vi "TLB Native Dynamic Events ver 0.18c.vi"() -> ()   [LabVIEW 2018]
uses:
  Labview Training Phase 2/Enum Controls/States for Action Engine.ctl
  TLB Type Definitions/State Type Definitions, for 0.26d versions and later.ctl
  TLB Type Definitions/Intruction Type Definitions.ctl
  TLB Type Definitions/Encoder cluster.ctl
  TLB Type Definitions/PING CLUSTER.ctl
  <vilib>/Studica/Studica Toolkit/NavX/NavX.lvlib
  <vilib>/Studica/Studica Toolkit/Background/DIO Channel.ctl
  Underlying VI's/NavX VI/navX type def.ctl
  <vilib>/Studica/Studica Toolkit/Background/I2C Channel.ctl
  TLB Type Definitions/Vision cluster.ctl
  <vilib>/NI_Real-Time Target Support.lvlib
  TLB Type Definitions/Stepper cluster.ctl
  Experimental VI's/Archived VI's/MOTOR CONTROL NO PID Type Def.ctl
  Underlying VI's/I2C Master VI/I2C MASTER Type Def.ctl
  Underlying VI's/I2C Master VI/I2C_MASTER_WRITE_NEW Type Def.ctl
  <vilib>/userdefined/High Color/IMAQdx.ctl
  Underlying VI's/I2C Master VI/Arduino_Interfacing.ctl
  TLB Type Definitions/Yaw Cluster.ctl
  TLB Type Definitions/Time cluster.ctl
  TLB Type Definitions/Y Stepper cluster.ctl
  Underlying VI's/Modified webcam FGV/Webcam AE.ctl
  Underlying VI's/Elasped Timer/Elapsed timer control.ctl
  Underlying VI's/Motor Control VI with PID/MOTOR CONTROL WITH PID AE DATA MODE TYPE DEF.ctl
  Underlying VI's/Motor Control VI with PID/MOTOR CONTROL WITH PID AE DIRECTION TYPE DEF.ctl
  TLB Type Definitions/IR Sensor Type Def.ctl
  <vilib>/myRIO/Common/Instrument Driver Framework/myRIO v1.0/AI/typedefs/AI Channels Enum.ctl
  <vilib>/myRIO/Common/Instrument Driver Framework/myRIO v1.0/AI/typedefs/AI Channels List.ctl
  TLB Type Definitions/Motor Speed Cluster.ctl
  Underlying VI's/IMAQ Create Reference AE/IMAQ Reference AE.ctl
  TLB Type Definitions/Line Sensor Cluster.ctl
  Underlying VI's/Line Sensor AE/Line Sensor AE Type Def.ctl
  <vilib>/Utility/RT CPU Load.ctl
  <vilib>/Studica/Studica Toolkit/NavX/TypeDefs/Flags/Z900_navX_Flags_CalibrationStatusTypeDef.ctl
  <vilib>/Studica/Studica Toolkit/NavX/TypeDefs/Flags/Z900_navX_Flags_OpStatusTypeDef.ctl
panel:
  out "Status":T3 {"OP Status" items=["INITIALIZING", "SELFTEST_IN_PROGRESS", "ERROR", "IMU_AUTOCAL_IN_PROGRESS", "NORMAL"]; "Calibration Status" items=["IMU_CAL_STATE_MASK"=3, "IMU_CAL_STATE_INPROGRESS"=0, "IMU_CAL_STATE_ACCUMULATE"=1, "IMU_CAL_STATE_COMPLETE"=2]}
  out "General Errors":errorcluster
  in  "Red LED":bool
  out "Arm IR Sensor":dbl
  out "Table obstruct":bool
  out "x-y":dbl
  out "Left IR Sensor":dbl
  out "Obstacle detected":bool
  out "Speed & distance":T4
  out "Object Center Coordinates":cluster{"x":sgl, "y":sgl}
  out "Object detection cluster":T5
  out "Time up flag":bool
  out "Task selection":u8
  in  "Object recognition mode":enum16{"Ball", "Soap", "Gel", "Pipe", "None"}(ring)
  out "NavX Readings":T6
  out "Arduino Data":T7
  out "CPU loads":T8[](array[typedef]) {"ISR (%)" format="%#.2f"; "Idle (%)" format="%#.2f"; "Background (%)" format="%#.2f"; "Normal (%)" format="%#.2f"; "Above Normal (%)" format="%#.2f"; "High (%)" format="%#.2g"; "Timed Structures (%)" format="%#.2g"; "Time Critical (%)" format="%#.2g"; "Total (%)" format="%#.2g"}
  out "TASK ENABLE":bool
  out "Rising Edge":bool
  in  "Green LED":bool
  out "State Logic":T9=enum."Startup"
  out "elements":T10[](array[typedef])
  in  "STOP TASK":bool
  in  "OK Button":bool
  in  "STOP":bool
  out "Queue Errors":errorcluster
  out "Action Queue Items":i32
  out "State Logic Queue Items":i32
  out "Action Queues items":string[](array[string])=["Hardware reset", "Software reset", ""]
  out "Action State":string
  # "System Health Status Update"
  # "VISION"
  # "TLB FRAMEWORK STATUS"
  # "Test Programme written by Calvin Loke    Dated: 28 Aug 2019\nTest Programme revised by Dr Alex See   Dated 30 Aug 2019\n\nRevision date: 20/03/2020\nProgramme version:   TLB Native Dynamic Events ver 0.14a"
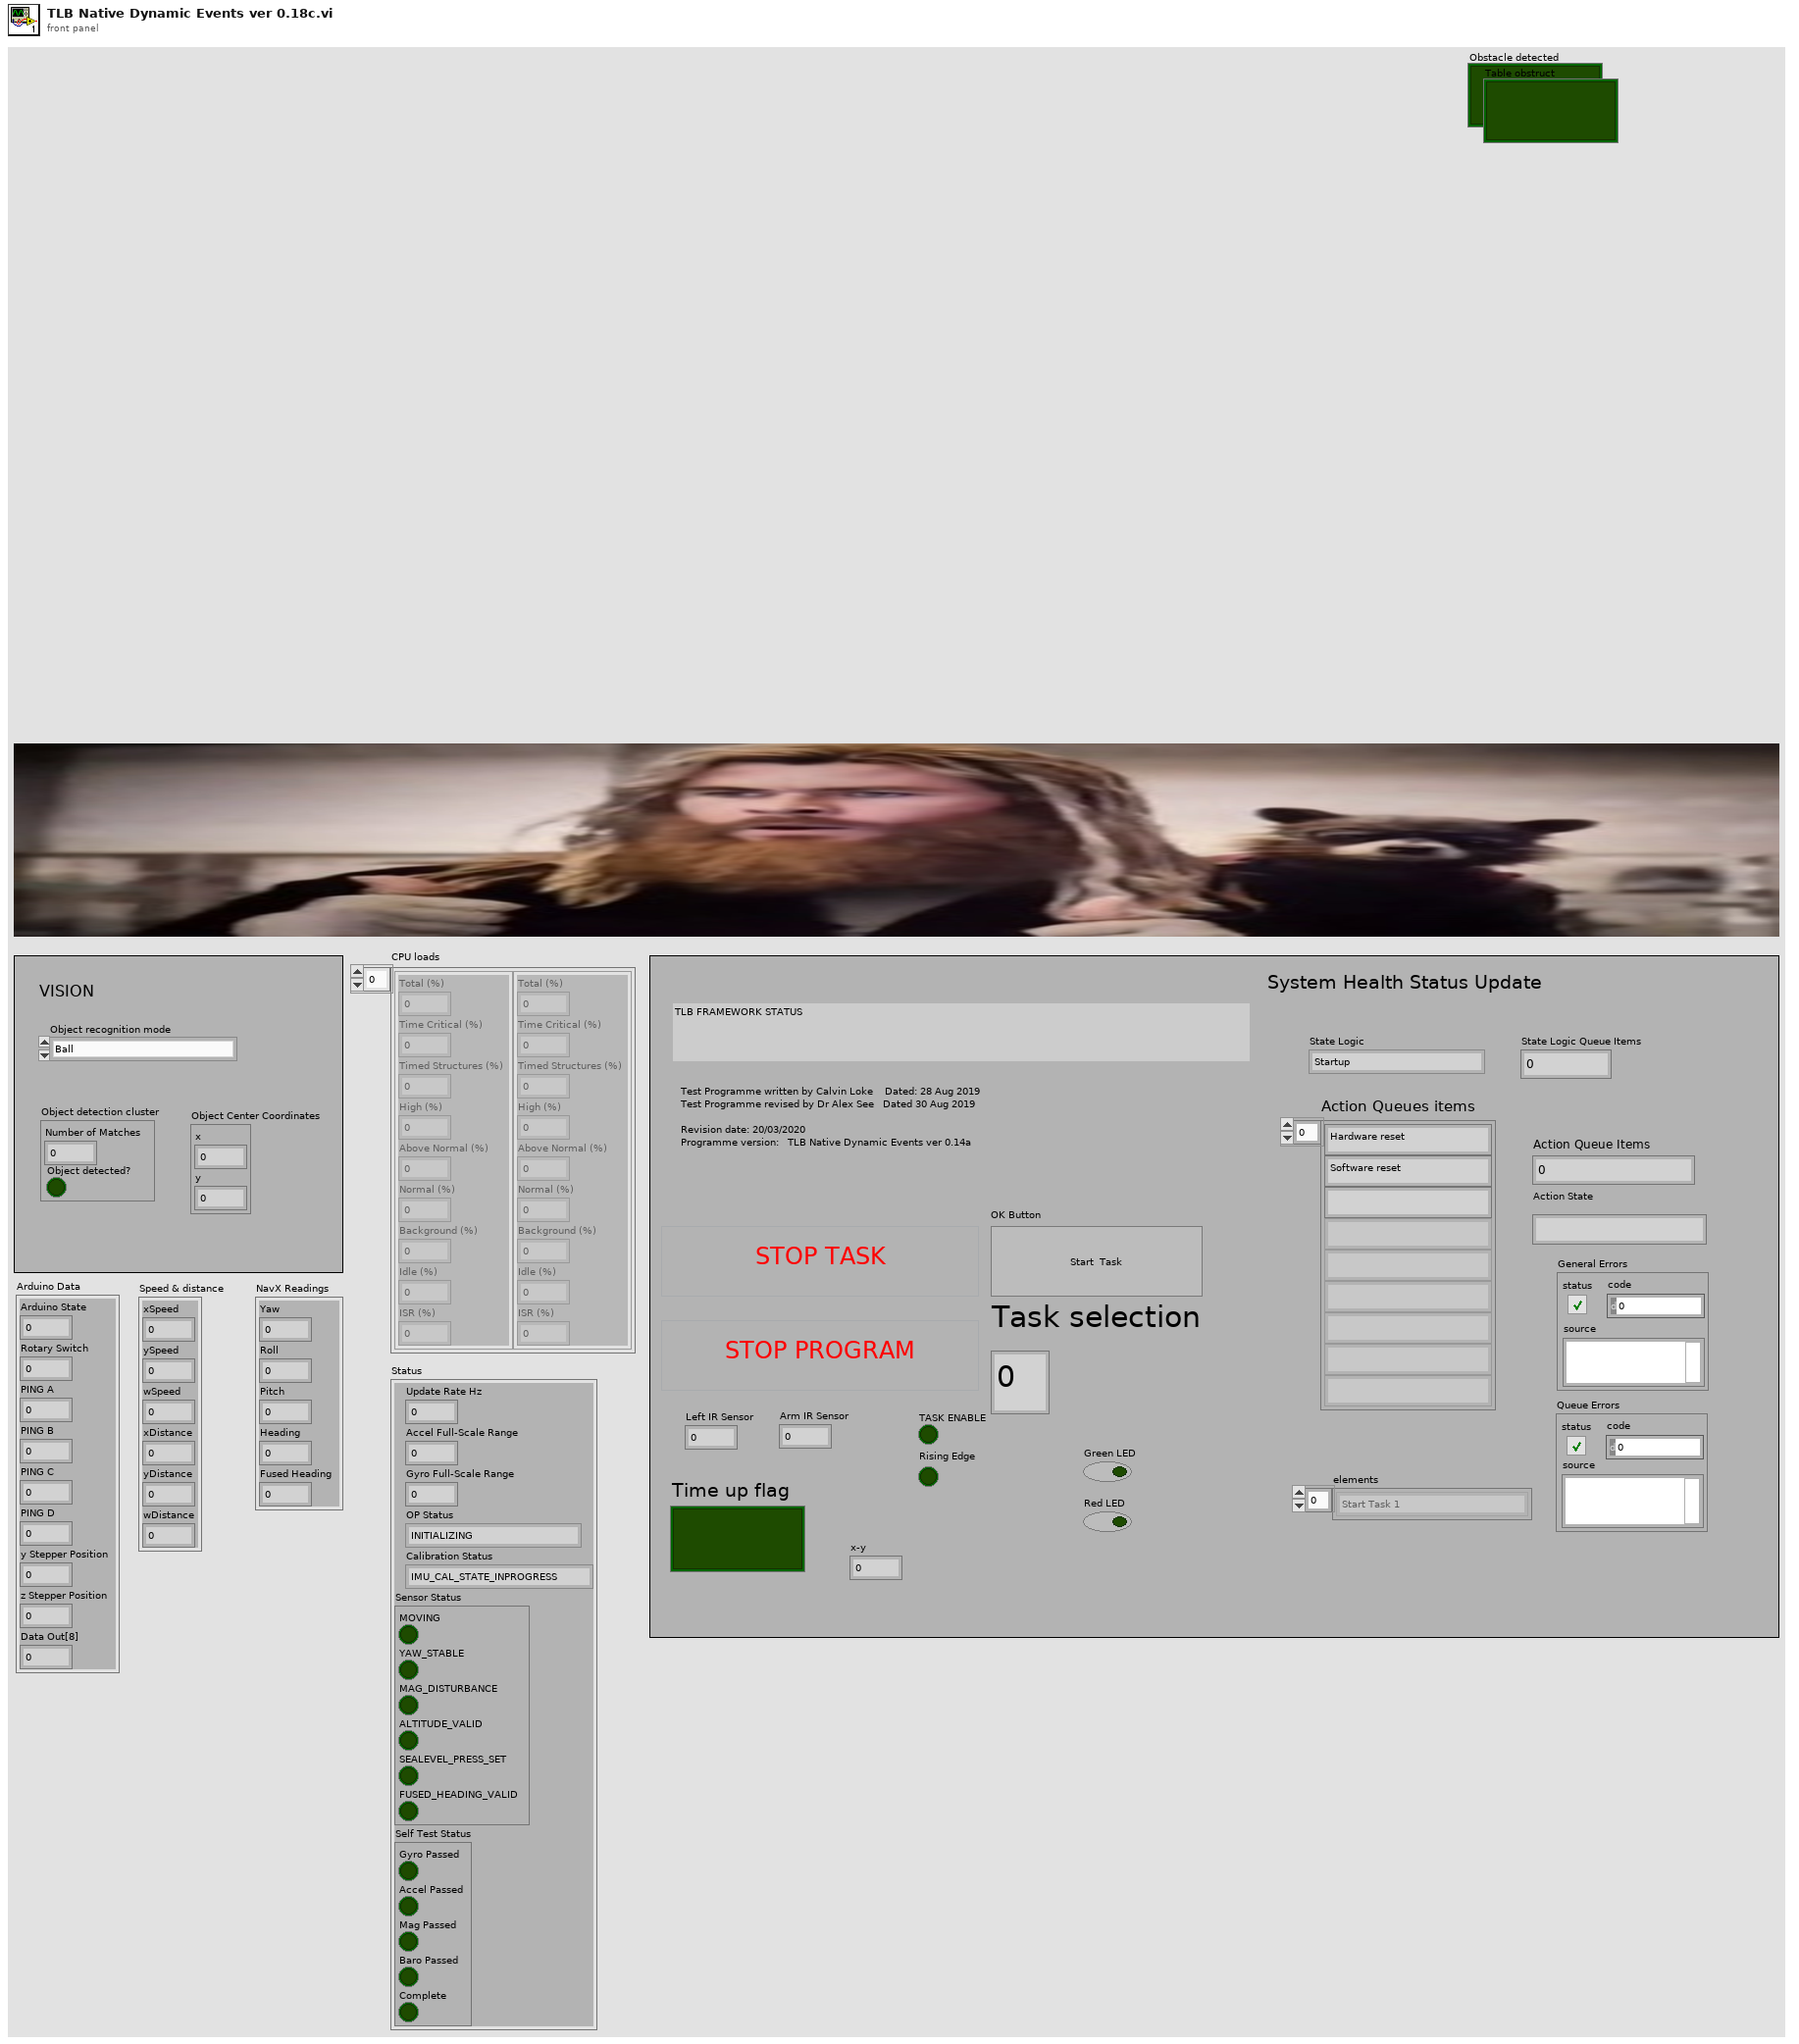
[diagram p1: front panel]
types:
  T1 = typedef "NavX.lvlib/Z900_navX_Flags_OpStatusTypeDef.ctl" = u8
  T2 = typedef "NavX.lvlib/Z900_navX_Flags_CalibrationStatusTypeDef.ctl" = u8
  T3 = cluster{"Update Rate Hz":u8, "Accel Full-Scale Range":u8, "Gyro Full-Scale Range":u16, "OP Status":T1, "Calibration Status":T2, "Sensor Status":cluster{"MOVING":bool, "YAW_STABLE":bool, "MAG_DISTURBANCE":bool, "ALTITUDE_VALID":bool, "SEALEVEL_PRESS_SET":bool, "FUSED_HEADING_VALID":bool}, "Self Test Status":cluster{"Gyro Passed":bool, "Accel Passed":bool, "Mag Passed":bool, "Baro Passed":bool, "Complete":bool}}
  T4 = cluster{"xSpeed":dbl, "ySpeed":dbl, "wSpeed":dbl, "xDistance":dbl, "yDistance":dbl, "wDistance":dbl}
  T5 = cluster{"Number of Matches":i32, "Object detected?":bool}
  T6 = cluster{"Yaw":dbl, "Roll":dbl, "Pitch":dbl, "Heading":dbl, "Fused Heading":dbl}
  T7 = cluster{"Arduino State":u8, "Rotary Switch":u8, "PING A":u8, "PING B":u8, "PING C":u8, "PING D":u8, "y Stepper Position":u8, "z Stepper Position":u8, "Data Out[8]":u8}
  T8 = typedef "NI_Real-Time Target Support.lvlib/RT CPU Load.ctl" = cluster{"Total (%)":dbl, "Time Critical (%)":dbl, "Timed Structures (%)":dbl, "High (%)":dbl, "Above Normal (%)":dbl, "Normal (%)":dbl, "Background (%)":dbl, "Idle (%)":dbl, "ISR (%)":dbl}
  T9 = typedef "State Type Definitions.ctl" = enum16{"None", "Startup", "Move to Angle", "True Stop", "Idle", "Shutdown", "Task 1A", "Task 1B", "Task 2:Raise Arm", "Task 2:Sensor Mode", "Task 2:Reverse Mode", "Task 3", "Task 4_A", "Task 4_B", "Task 4_C", "Task 4_D", "Task 5A", "Task 5B", "Task 5C", "Task 5D", "Task 5E: POSITION ARM", "Task 5F: ARM GRAB HEIGHT", "Task 5G: CLOSE CLAW", "Task 5H: RAISE ARM", "Task 6_A", "Task 6_B", "Task 7", "Task 8A: RAISE ARM", "Task 8B: MOVE TO BOX", "Task 8C: CAM BURST", "Task 8D: PROCESS IMAGE", "Task 8E: ROBOT ADJUST", "Task 8F: CAM BURST 2", "Task 8G: PROCESS IMAGE 2", "Task 8H: ARM ADJUST", "Task 8I: ARM GRAB HEIGHT", "Task 8J: CLOSE CLAW", "Task 8K: RAISE MY SWORD", "Task 9A: Raise Arm", "Task 9B: Rotate to Angle", "Task 9C: Detect Box", "Task 9D: MOVE FORWARD", "Task 9E: MOVE LEFT", "Task 9F: SCAN IMAGE", "Task 9G: PROCESS COLOUR", "Task 9H: MOVE RIGHT", "Task 9I: SCAN IMAGE", "Task 9J: PROCESS COLOUR", "Task 9K: ROTATE 90 CW", "Task 9L: MOVE FORWARD", "Task 9M: MOVE RIGHT", "Task 9N: SCAN IMAGE", "Task 9O: PROCESS COLOUR", "Task 9P: MOVE RIGHT", "Task 9Q: SCAN IMAGE", "Task 9R: PROCESS COLOUR", "Task A1: Raise Arm", "Task A2: Rotate to Angle", "Task A3: Move Forward", "Task A4: Rotate CW 90"}
  T10 = typedef "Intruction Type Definitions.ctl" = enum16{"None", "Start Task 1", "Start Task 2", "Start Task 3", "Start Task 4", "Start Task 5", "Start Task 6", "Start Task 7", "Start Task 8 - BALL", "Start Task 8 - Gel", "Start Task 8 - Pipe", "Start Task 8 - Soap", "Start Task 9", "Start Task A", "Start Task B", "Exit"}
  T11 = typedef "Line Sensor Cluster.ctl" = cluster{"Line Detected?":bool, "S1":dbl, "S2":dbl, "S3":dbl, "S4":dbl}
  T12 = typedef "Motor Speed Cluster.ctl" = cluster{"ySpeed":dbl, "xSpeed":dbl, "wSpeed":dbl}
  T13 = typedef "IR Sensor Type Def.ctl" = cluster{"Left IR Sensor":dbl, "Arm IR Sensor":dbl, "Bottom IR Sensor":dbl}
  T14 = typedef "Y Stepper cluster.ctl" = cluster{"yStepper desired":u8}
  T15 = typedef "Time cluster.ctl" = cluster{"Time up flag":bool, "SET TIME TO CHECK":dbl}
  T16 = typedef "Yaw Cluster.ctl" = cluster{"Yaw":dbl, "Compass":dbl}
  T17 = typedef "Stepper cluster.ctl" = cluster{"y Stepper Position":u8, "z Stepper Position":u8}
  T18 = typedef "DIO Channel.ctl" = enum16{"Not Connected", "A/DIO1", "A/DIO2", "A/DIO3", "A/DIO4", "A/DIO5", "A/DIO6", "A/DIO7", "A/DIO13", "B/DIO1", "B/DIO2", "B/DIO3", "B/DIO4", "B/DIO5", "B/DIO6", "B/DIO7", "B/DIO13", "C/DIO0", "C/DIO1", "C/DIO2", "C/DIO3", "C/DIO4", "C/DIO5", "C/DIO6", "C/DIO7"}
  T19 = typedef "Vision cluster.ctl" = cluster{"Recognized Object":bool, "Object X coordinate":dbl, "Object Y coordinate":dbl}
  T20 = typedef "PING CLUSTER.ctl" = cluster{"PING_A":u8, "PING_B":u8, "PING_C":u8, "PING_D":u8}
  T21 = typedef "Encoder cluster.ctl" = cluster{"xDistance":dbl, "yDistance":dbl, "wDistance":dbl}
  T22 = cluster{"DIO Channel":T18, "FPGA VI Reference Out":refnum<k20>}
  T23 = typedef "navX type def.ctl" = enum16{"Get i2C reference", "Read Values", "Zero Yaw"}
  T24 = typedef "Arduino_Interfacing.ctl" = enum16{"Initialize", "Write to Arduino", "Read From Arduino"}
  T25 = typedef "I2C Channel.ctl" = enum16{"Not Connected", "A", "B"}
  T26 = typedef "States for Action Engine.ctl" = enum16{"Initialize", "Write", "Read"}
  T27 = cluster{"I2C Ref Out":cluster{"I2C Channel":T25, "FPGA VI Reference Out":refnum<k20>}, "Connected":bool, "Slave Address (7-bit)":u8, "Registry":u8[]}
  T28 = typedef "Intruction Type Definitions.ctl" = enum16{"None", "Start Task 1", "Start Task 2", "Start Task 3", "Start Task 4", "Start Task 5", "Start Task 6", "Start Task 7", "Start Task 8", "Start Task 9", "Start Task A", "Start Task B", "Exit"}
  T29 = typedef "State Type Definitions.ctl" = enum16{"None", "Startup", "Move to Angle", "True Stop", "Idle", "Shutdown", "Task 1", "Task 2:Raise Arm", "Task 2:Sensor Mode", "Task 2:Reverse Mode", "Task 3", "Task 4_A", "Task 4_B", "Task 4_C", "Task 4_D", "Task 5A: ARM CAM HEIGHT", "Task 5B: MOVE TO BOX", "Task 5C: CAM BURST", "Task 5D: PROCESS IMAGE", "Task 5E: POSITION ARM", "Task 5F: ARM GRAB HEIGHT", "Task 5G: CLOSE CLAW", "Task 5H: RAISE ARM", "Task 6_A", "Task 6_B", "Task 7", "Task 8A: RAISE ARM", "Task 8B: MOVE TO BOX", "Task 8C: CAM BURST", "Task 8D: PROCESS IMAGE", "Task 8E: ROBOT ADJUST", "Task 8F: CAM BURST 2", "Task 8G: PROCESS IMAGE 2", "Task 8H: ARM ADJUST", "Task 8I: ARM GRAB HEIGHT", "Task 8J: CLOSE CLAW", "Task 8K: RAISE MY SWORD", "Task 9A: Raise Arm", "Task 9B: Rotate to Angle", "Task 9C: Rotation alignmnet", "Task 9D: Move Forward", "Task A: RAISE ARM TO HEIGHT", "Task A: MOVE FORWARD"}
  T30 = typedef "MOTOR CONTROL WITH PID AE DIRECTION TYPE DEF.ctl" = enum16{"y-axis movement", "x-axis movement", "rotation", "stop", "reset encoders"}
  T31 = typedef "MOTOR CONTROL WITH PID AE DATA MODE TYPE DEF.ctl" = enum16{"Init AE", "Write to AE", "Read from AE"}
  T32 = typedef "Line Sensor AE Type Def.ctl" = enum16{"INIT AE", "READ FROM LINE SENSORS"}
  T33 = typedef "IMAQ Reference AE.ctl" = enum16{"Initialize AE", "Get IMAQ Reference", "Dispose Processing Buffer"}
  T34 = typedef "Elapsed timer control.ctl" = enum16{"Start", "Pause", "Initialize"}
  T35 = typedef "I2C_MASTER_WRITE_NEW Type Def.ctl" = enum16{"Ultrasonic sensors", "Stepper origin", "zStepper 13.3k", "zStepper 13k", "zStepper 12k", "zStepper 11k", "zStepper 10k", "zStepper 9k", "zStepper 8k", "zStepper 7k", "zStepper 6k", "zStepper 5k", "zStepper 4k", "zStepper 3k", "zStepper 2k", "zStepper 1k", "zStepper 900", "zStepper 800", "zStepper 700", "zStepper 600", "zStepper 500", "zStepper 400", "zStepper 300", "zStepper 200", "zStepper 100", "zStepper 0", "yStepper control", "Open Claw", "Close Claw", "Soft Reset"}
  T36 = typedef "Webcam AE.ctl" = enum16{"Initialize Camera", "Open Camera", "Continuous Acquisition", "Close Camera", "Retrieve Image", "Dispose Camera Image Buffer"}
  T37 = typedef "IMAQdx.ctl" = refnum<k21>
  T38 = typedef "Webcam AE.ctl" = enum16{"Initialize Camera", "Open Camera", "Continuous Acquisition", "Close Camera", "Retrieve Image", "Dispose Image Buffers"}
  T39 = typedef "IMAQ Reference AE.ctl" = enum16{"Initialize AE", "Get IMAQ Reference", "Destroy ALL IMAQ"}
  T40 = typedef "MOTOR CONTROL NO PID Type Def.ctl" = enum16{"Init", "Front Back", "Left Right", "Rotate", "Stop", "Latch"}
  T41 = typedef "AI Channels List.ctl" = T42[]
  T42 = typedef "AI Channels Enum.ctl" = enum16{"Not Connected", "AudioIn/Left", "AudioIn/Right", "C/AI0", "C/AI1", "A/AI0", "A/AI1", "A/AI2", "A/AI3", "A/AI4", "A/AI5", "A/AI6", "A/AI7", "B/AI0", "B/AI1", "B/AI2", "B/AI3", "B/AI4", "B/AI5", "B/AI6", "B/AI7", "AI/AI0", "AI/AI1", "AI/AI2", "AI/AI3", "A/AI0 (DIFF)", "A/AI1 (DIFF)", "A/AI2 (DIFF)", "A/AI3 (DIFF)", "B/AI0 (DIFF)", "B/AI1 (DIFF)", "B/AI2 (DIFF)", "B/AI3 (DIFF)"}
  T43 = cluster{"S1":dbl, "S2":dbl, "S3":dbl, "S4":dbl, "Array[4]":dbl, "Array[5]":dbl, "Array[6]":dbl, "Array[7]":dbl, "Array[8]":dbl}
  T44 = typedef "I2C MASTER Type Def.ctl" = enum16{"Last State", "Mode 0", "Mode 1", "Mode 2", "Mode 3", "Mode 4", "Mode 5", "Mode 6", "Mode 7", "Mode 8", "Mode 9", "Mode 10"}
  T45 = typedef "IMAQ Image.ctl" = refnum<image>
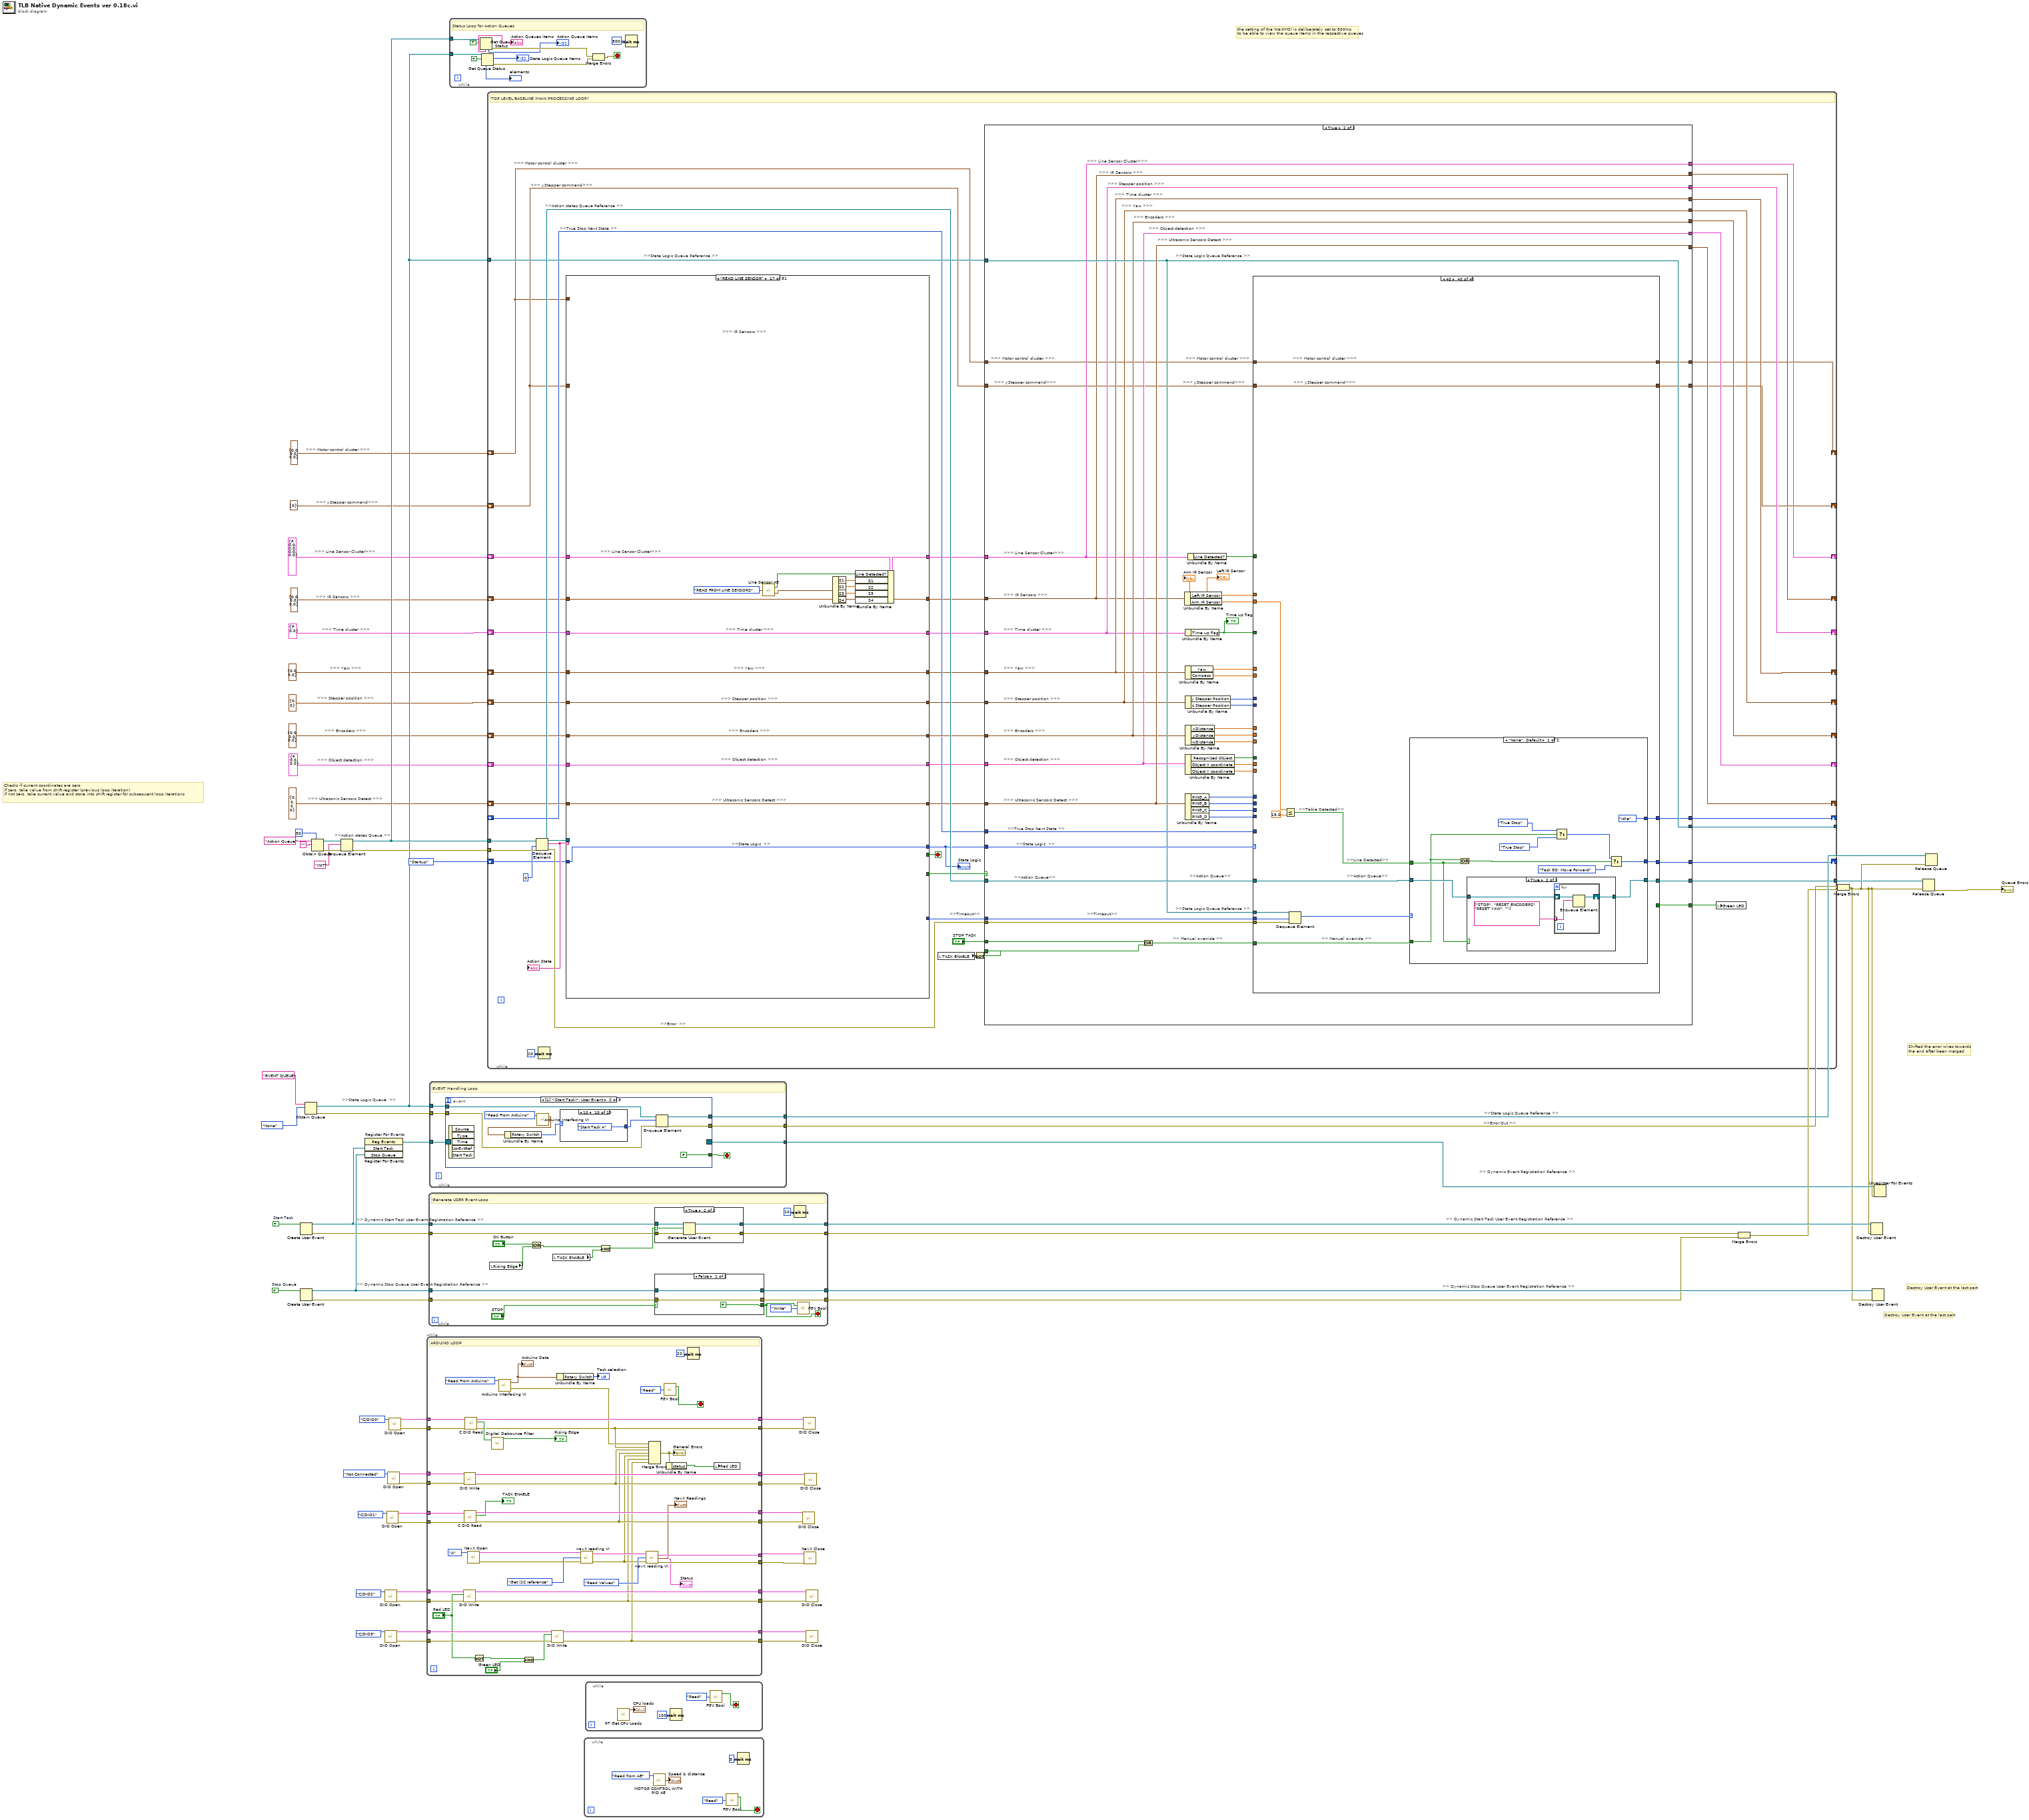
[diagram p0: block diagram]
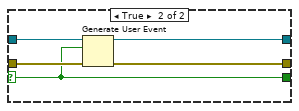
[diagram p2: hidden frame]
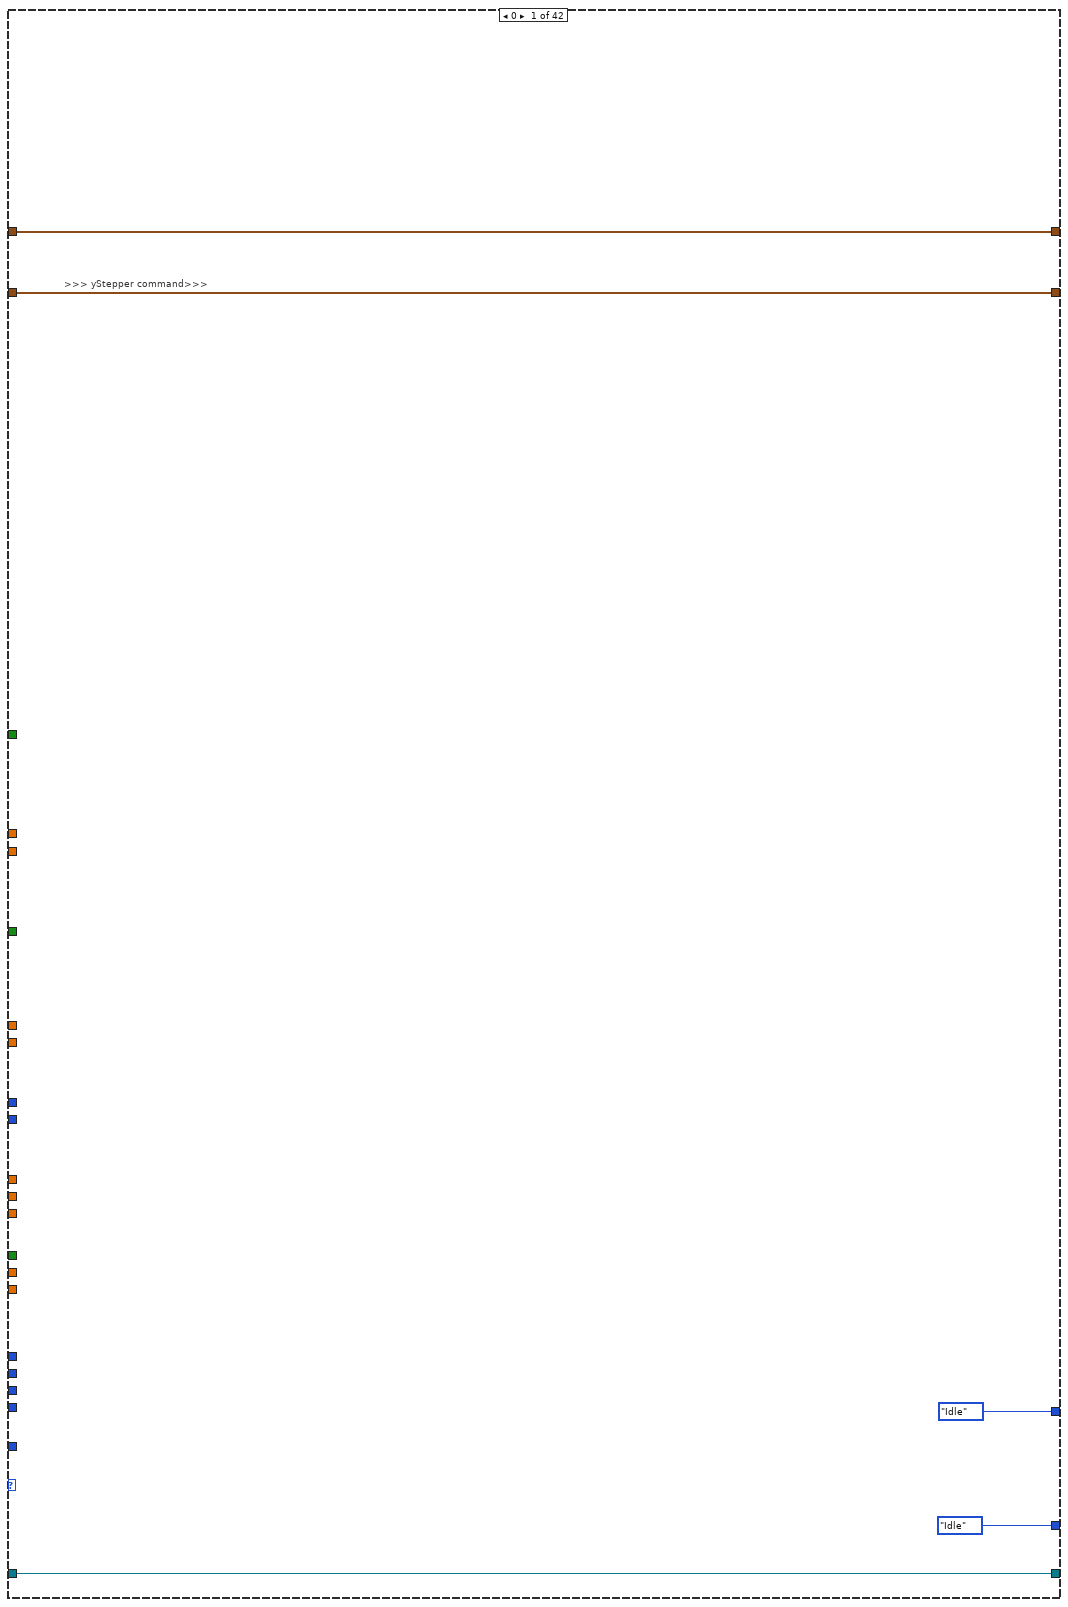
[diagram p5: hidden frame]
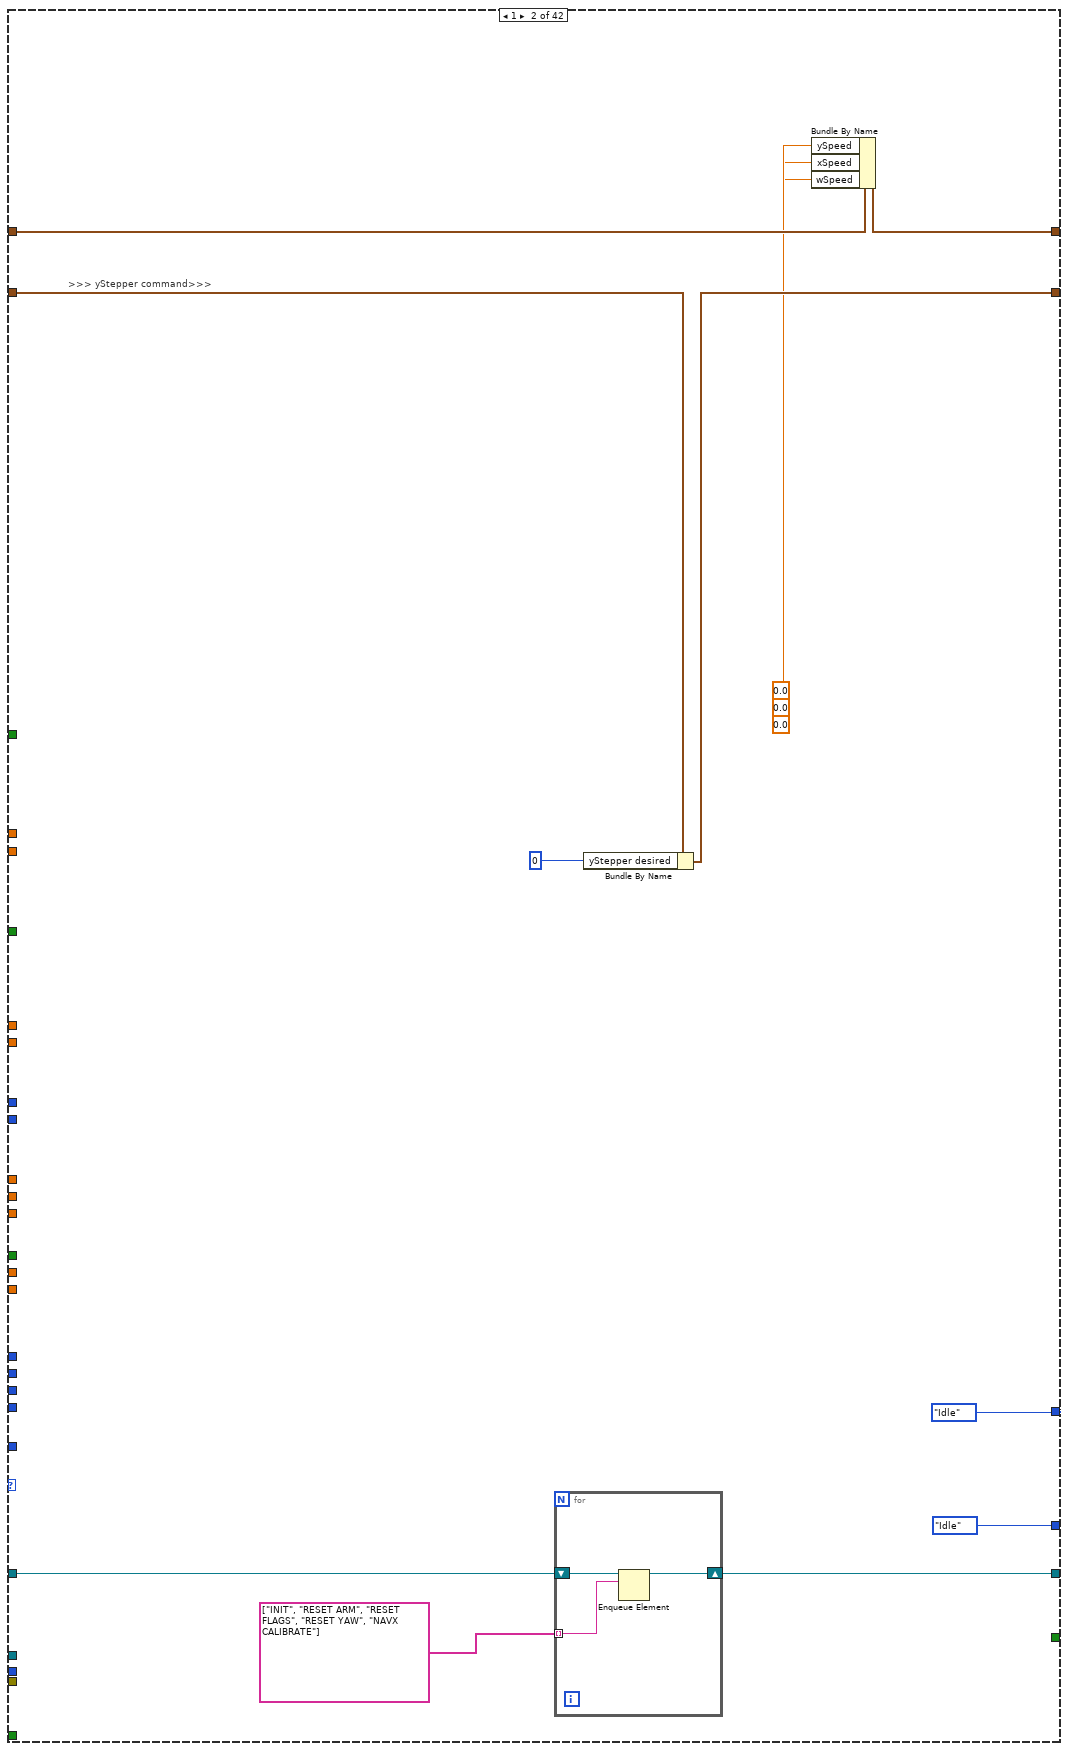
[diagram p6: hidden frame]
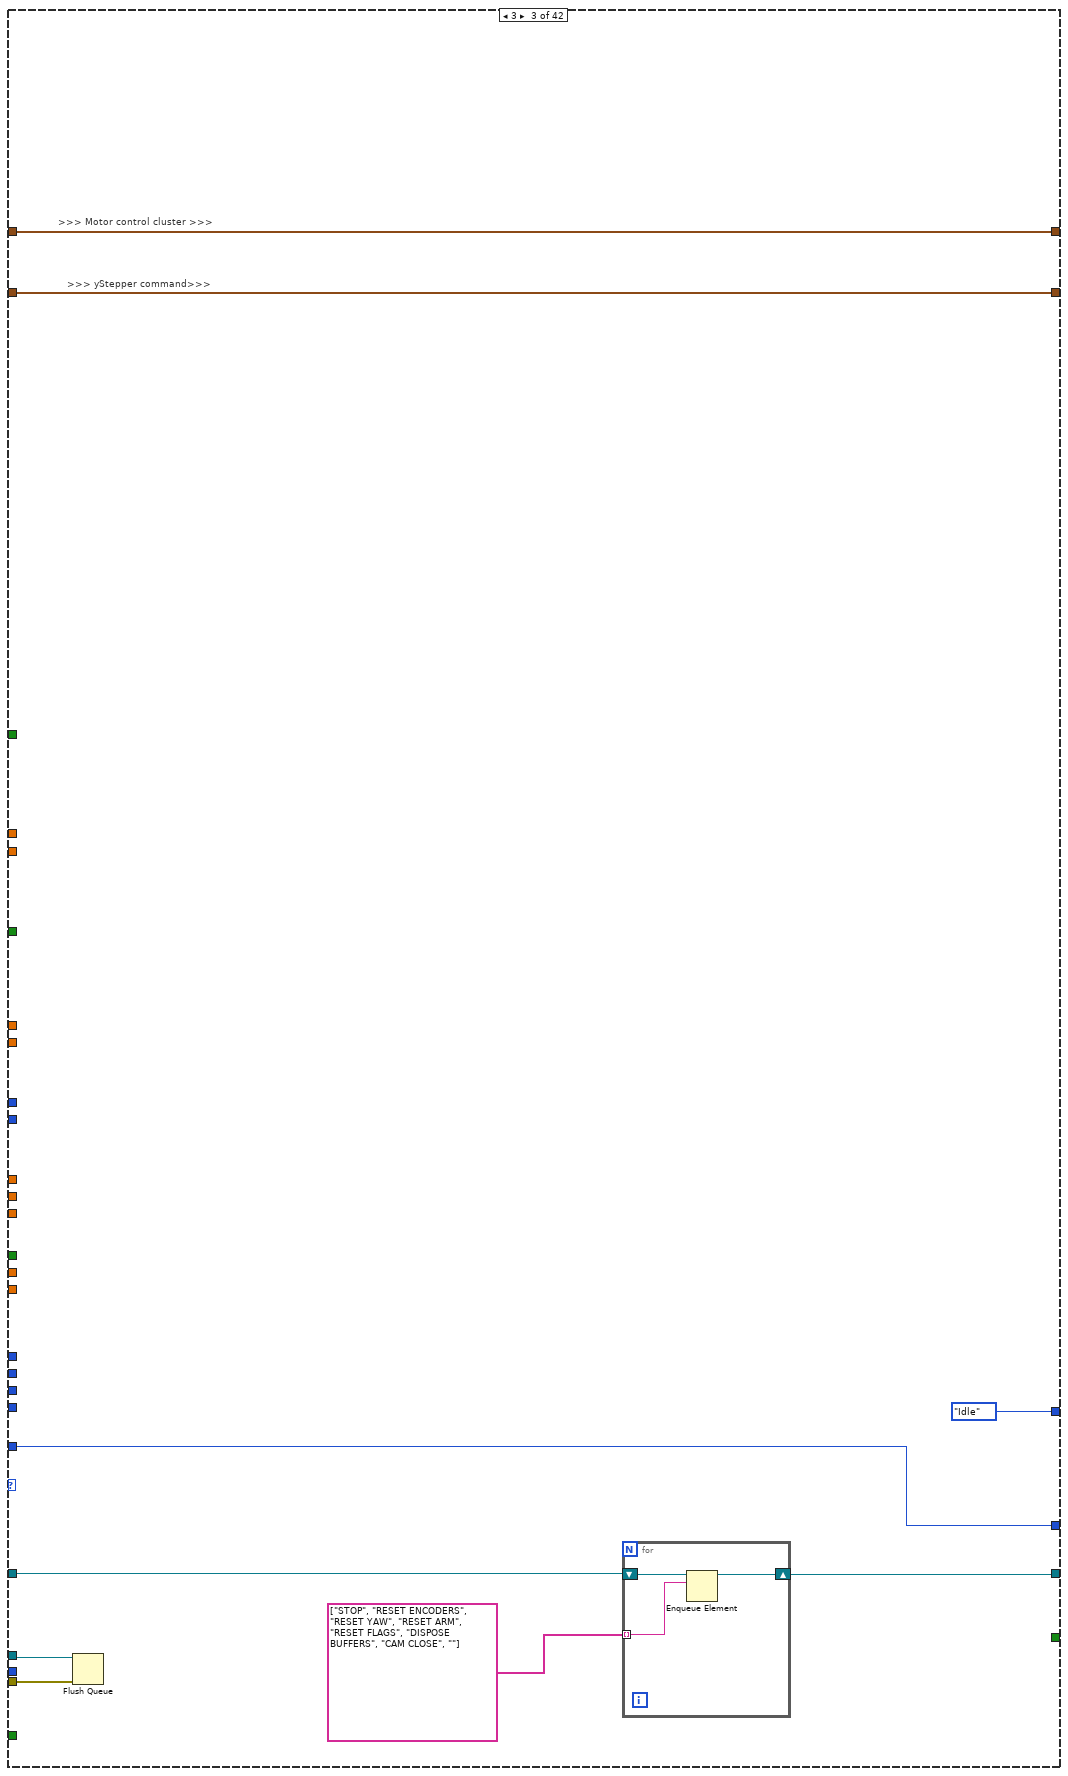
[diagram p7: hidden frame]
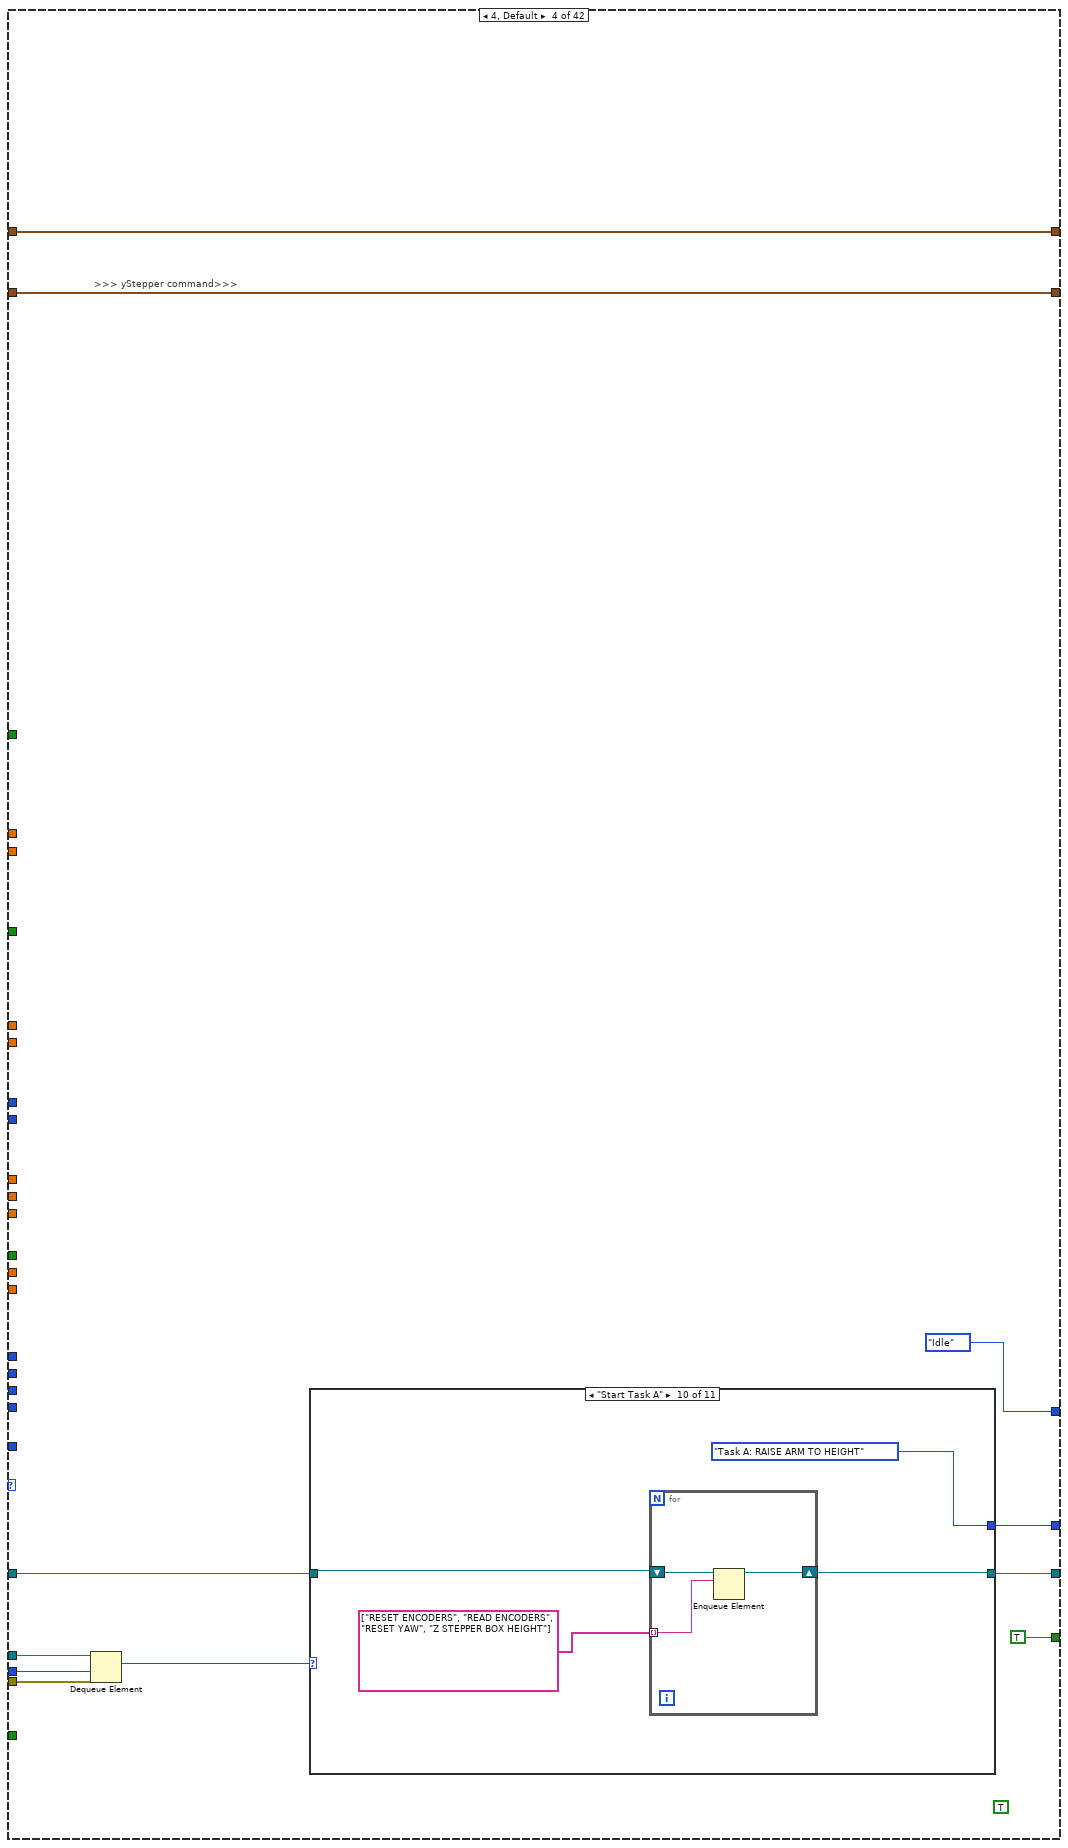
[diagram p8: hidden frame]
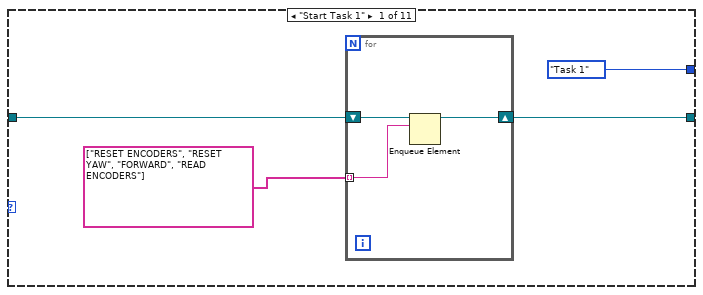
[diagram p9: hidden frame]
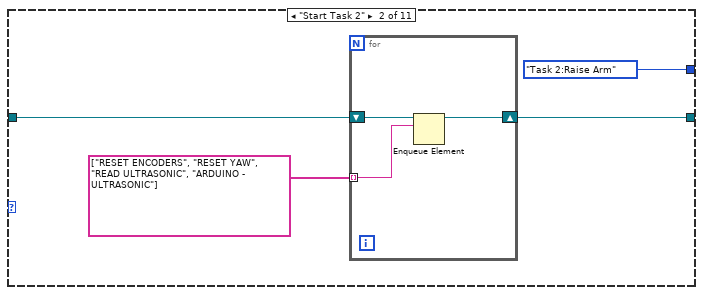
[diagram p10: hidden frame]
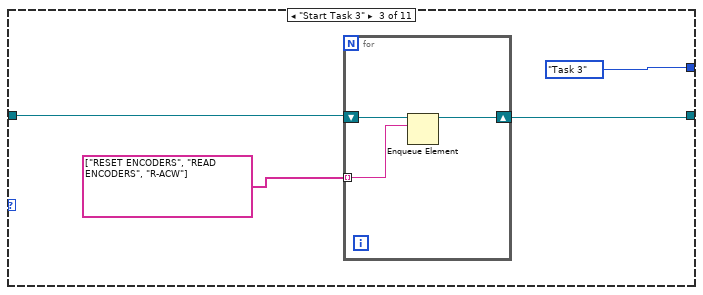
[diagram p11: hidden frame]
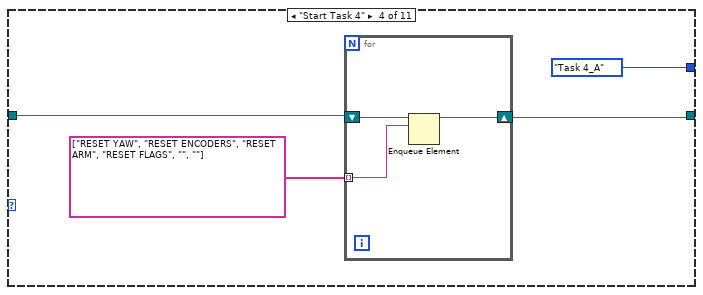
[diagram p12: hidden frame]
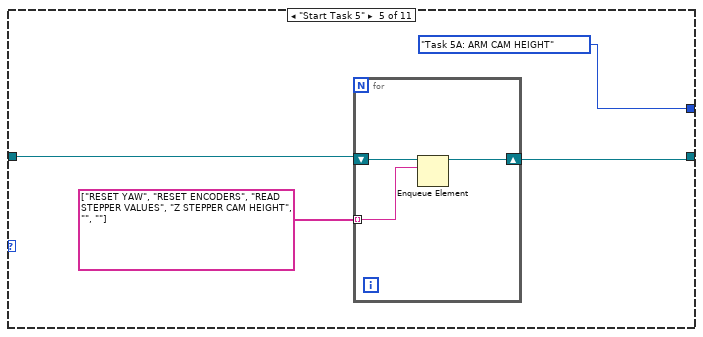
[diagram p13: hidden frame]
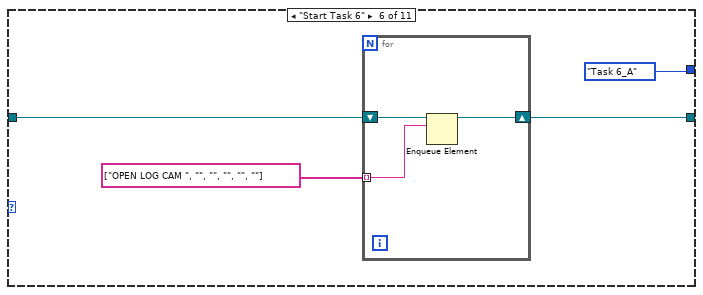
[diagram p14: hidden frame]
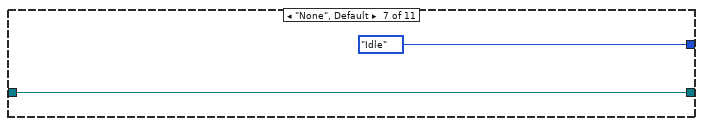
[diagram p15: hidden frame]
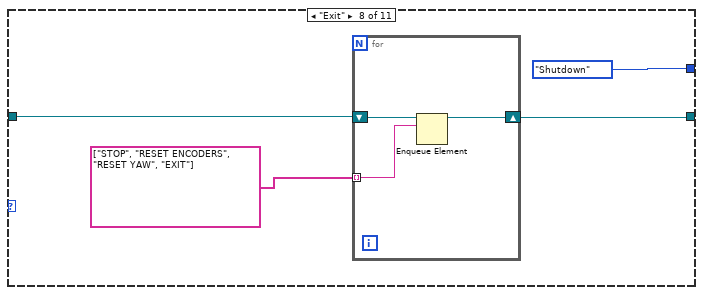
[diagram p16: hidden frame]
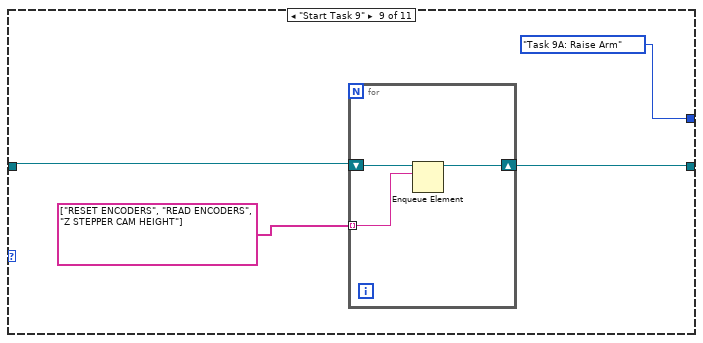
[diagram p17: hidden frame]
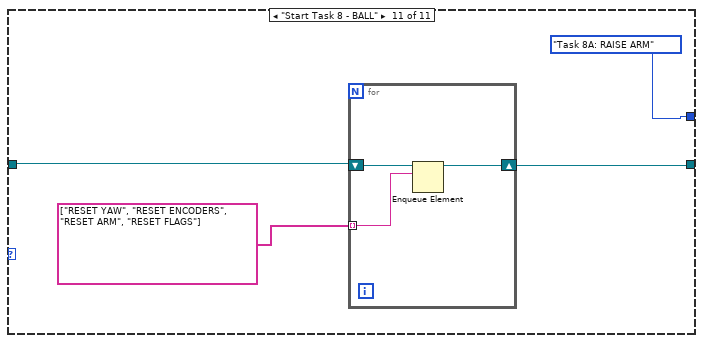
[diagram p18: hidden frame]
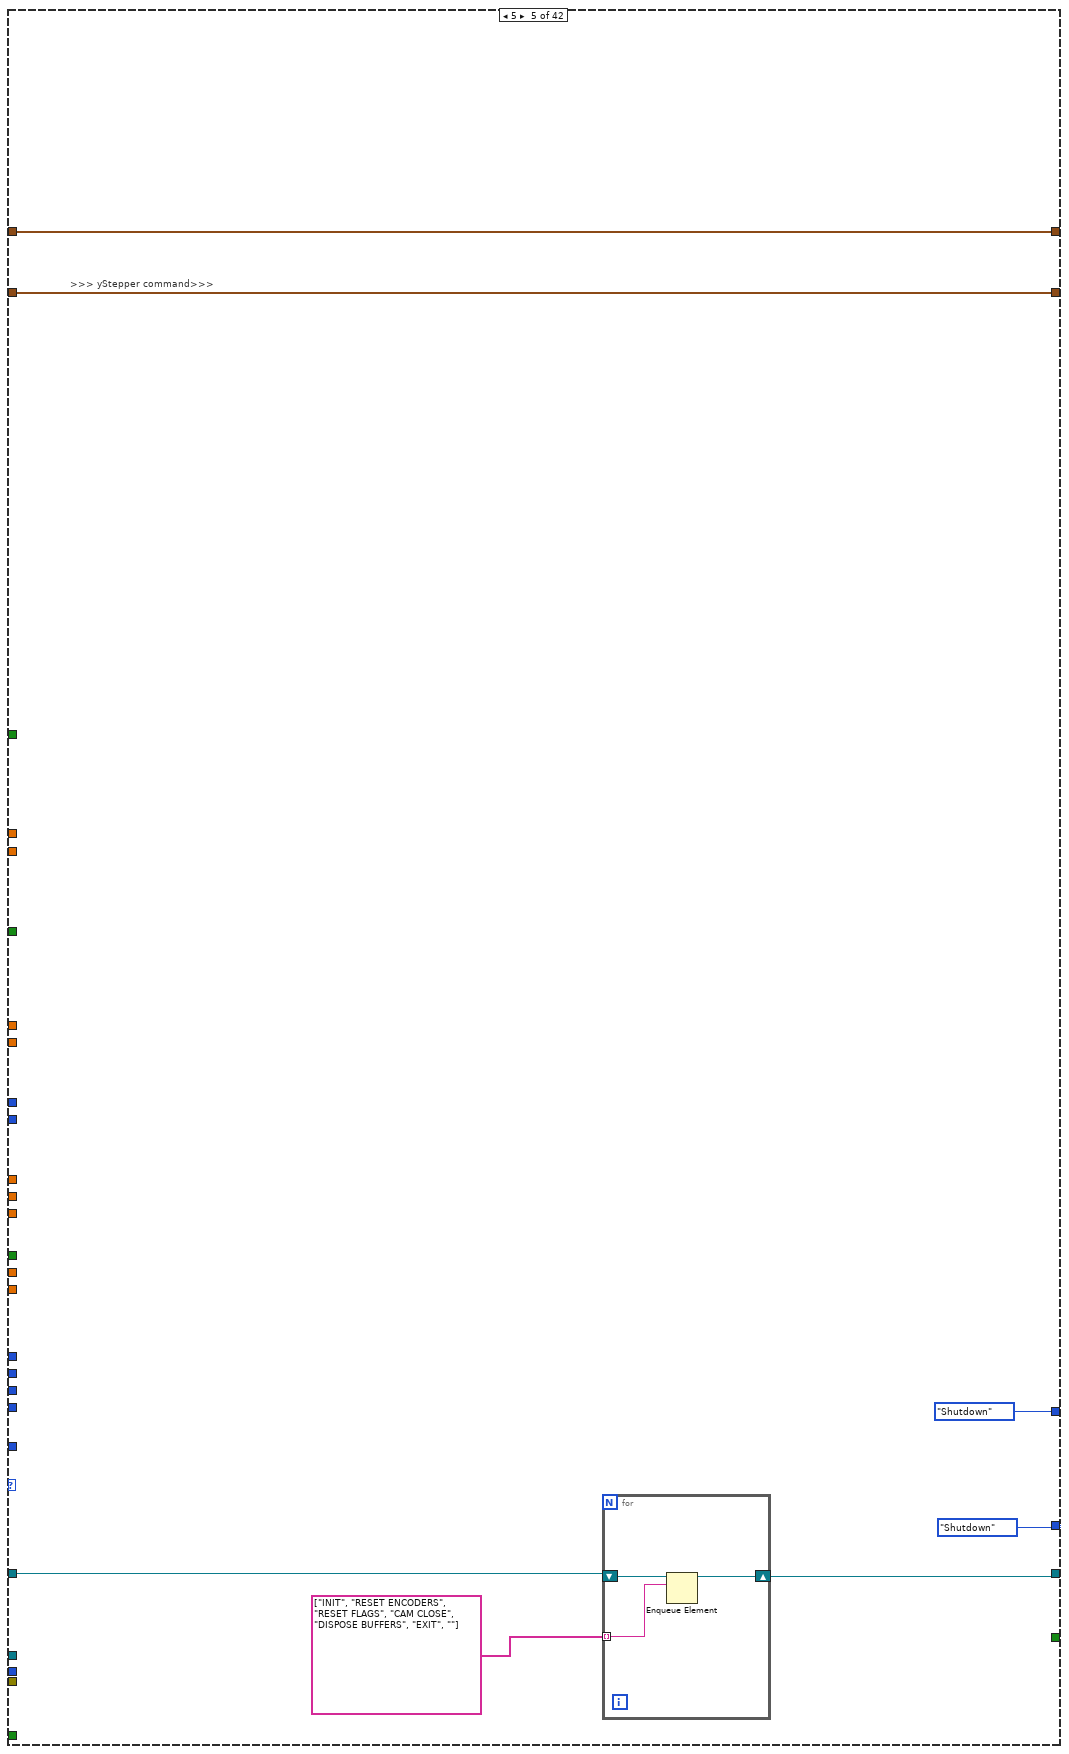
[diagram p19: hidden frame]
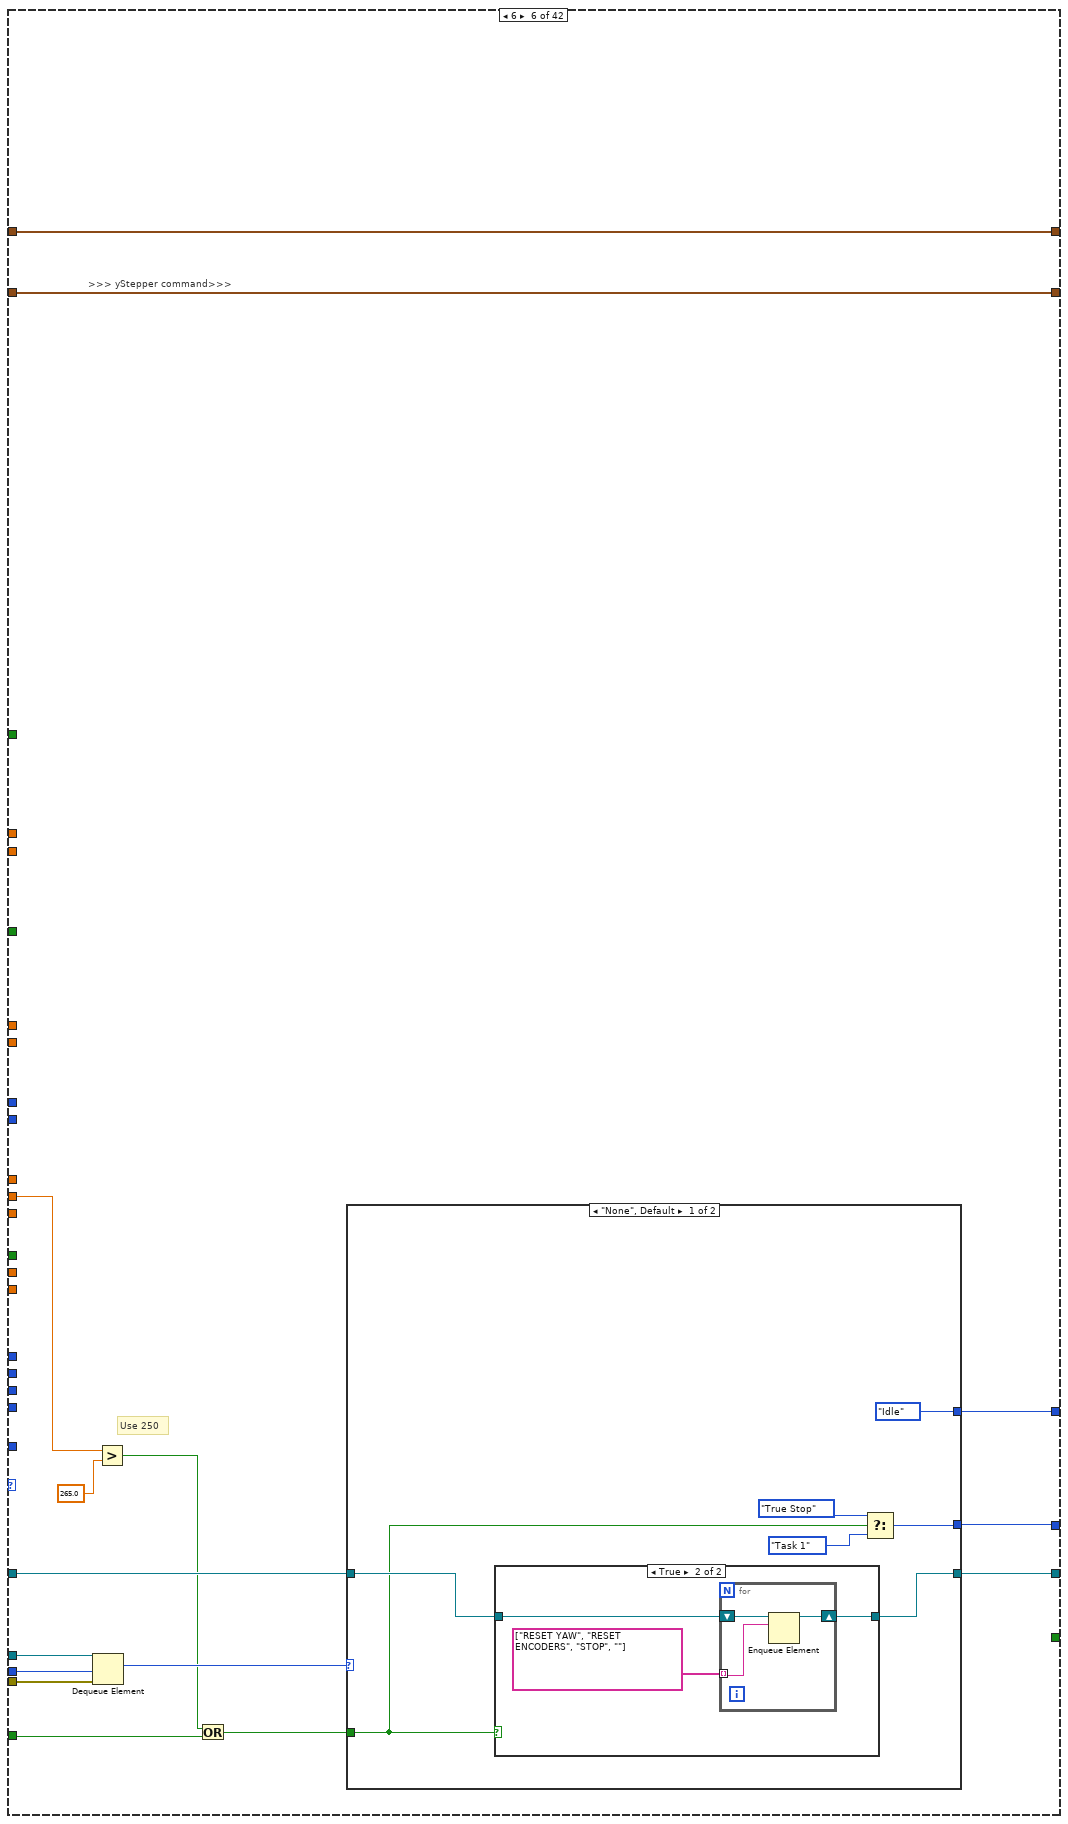
[diagram p20: hidden frame]
diagram:
  w68 = TRUE  # Stop Queue
  w67 = TRUE  # Start Task
  # ">>> Line Sensor Cluster>>>"
  # ">>> Motor control cluster >>>"
  # ">>> IR Sensors >>>"
  # "Checks if current coordinates are zero\nif zero, take value from shift register (previous loop iteration)\nif not zero, take current value and store into shift register for subsequent loop iterations"
  # ">>> yStepper command>>>"
  # ">>> Time cluster >>>"
  # ">>> Yaw >>>"
  # ">>> Stepper position >>>"
  # ">>> Encoders >>>"
  # ">>> Object detection >>>"
  # ">>> Ultrasonic Sensors Detect >>>"
  # "the setting of the Wait(MS) is deliberately set to 500ms\nto be able to view the queue items in the respective queues"
  # ">>Error Out >>"
  # ">> Dynamic Stop Queue User Event Registration Reference >>"
  # ">> Dynamic Start Task User Event Registration Reference >>"
  # ">> Dynamic Stop Queue User Event Registration Reference >>"
  # ">> Dynamic Start Task User Event Registration Reference >>"
  # ">> Dynamic Event Registration Reference >>"
  # ">>Action states Queue >>"
  # ">>State Logic Queue  >>"
  # ">>State Logic Queue Reference >>"
  # "Destroy User Event at the last part"
  # "Destroy User Event at the last part"
  # "Shifted the error wires towards\nthe end after been merged"
  n1 = Create User Event(user event datatype=w67) -> (user event=w59:refnum<user-event>, error out=w64:errorcluster)  [unwired: 1 in]
  n2 = Create User Event(user event datatype=w68) -> (user event=w60:refnum<user-event>, error out=w63:errorcluster)  [unwired: 1 in]
  n3 = Obtain Queue(name (unnamed)="EVENT QUEUE", element data type=Intruction_Type_Definitions."None" ("Enum")) -> (queue out=w45:refnum<queue>, error out=w51:errorcluster)  [unwired: 3 in, 1 out]
  n4 = Obtain Queue(max queue size (-1, unlimited)=50, name (unnamed)="Action Queue", element data type="") -> (queue out=w54:refnum<queue>, error out=w50:errorcluster)  [unwired: 2 in, 1 out]
  n5 = Enqueue Element(queue=w54, element="INIT", error in (no error)=w50) -> (queue out=w46:refnum<queue>, error out=w49:errorcluster)  [unwired: 1 in, 1 out]
  n6 = register-events "Register For Events"(w59, w60) -> (reference out=w58:refnum<event-registration>)  [unwired: 2 in, 1 out]
  n7 = call <vilib>:"DIO Open.vi"("DIO Channel"=DIO_Channel."C/DIO2") -> ("error out"=w18:errorcluster, "DIO Info Out"=w19:T22)  [unwired: 9 in]
  n8 = call <vilib>:"DIO Open.vi"("DIO Channel"=DIO_Channel."C/DIO3") -> ("error out"=w13:errorcluster, "DIO Info Out"=w14:T22)  [unwired: 9 in]
  n9 = call <vilib>:"DIO Open.vi"("DIO Channel"=DIO_Channel."C/DIO1") -> ("error out"=w23:errorcluster, "DIO Info Out"=w24:T22)  [unwired: 9 in]
  n10 = call <vilib>:"DIO Open.vi"("DIO Channel"=DIO_Channel."Not Connected") -> ("error out"=w28:errorcluster, "DIO Info Out"=w30:T22)  [unwired: 9 in]
  n11 = call <vilib>:"DIO Open.vi"("DIO Channel"=DIO_Channel."C/DIO0") -> ("error out"=w33:errorcluster, "DIO Info Out"=w36:T22)  [unwired: 9 in]
  n12 = while {
    tunnel: w36 -> [w112]
    tunnel: [w111] -> w34
    tunnel: w33 -> [w110]
    tunnel: [w81] -> w32
    tunnel: w30 -> [w107]
    tunnel: [w106] -> w29
    tunnel: w28 -> [w105]
    tunnel: [w80] -> w27
    tunnel: [w104] -> w25
    tunnel: w24 -> [w103]
    tunnel: w23 -> [w102]
    tunnel: [w79] -> w22
    tunnel: w19 -> [w96]
    tunnel: w18 -> [w95]
    tunnel: [w94] -> w17
    tunnel: [w77] -> w16
    tunnel: w14 -> [w93]
    tunnel: w13 -> [w92]
    tunnel: [w91] -> w12
    tunnel: [w76] -> w11
    tunnel: [w88] -> w8
    tunnel: [w87] -> w9
    stop <- w114 stop-if-true
    # "ARDUINO LOOP"
    n13 = call <vilib>:"DIO Write.vi"("error in (no error)"=w95, "Input"="Red LED", "DIO Info In"=w96) -> ("error out"=w77:errorcluster, "DIO Info Out"=w94:T22)  [unwired: 7 in]
    n14 = call <vilib>:"DIO Write.vi"("error in (no error)"=w105, "DIO Info In"=w107) -> ("error out"=w80:errorcluster, "DIO Info Out"=w106:T22)  [unwired: 8 in]
    n15 = call <vilib>:"C DIO Read.vi"("error in (no error)"=w102, "DIO Info In in"=w103) -> ("error out"=w79:errorcluster, "IN"=→"TASK ENABLE":bool, "DIO Info In out"=w104:T22)  [unwired: 7 in]
    n16 = call <vilib>:"C DIO Read.vi"("error in (no error)"=w110, "DIO Info In in"=w112) -> ("error out"=w81:errorcluster, "IN"=w109:bool, "DIO Info In out"=w111:T22)  [unwired: 7 in]
    n17 = call <vilib>:"NavX Open.vi"("I2C Channel"=I2C_Channel."A") -> ("error out"=w98:errorcluster, "NavX Info"=w100:T27)  [unwired: 9 in]
    n18 = Not(x="Red LED") -> (.not. x?=w70:bool)
    n19 = call "Digital Debounce Filter.vi"("Boolean input"=w109) -> ("Rising Edge"=→"Rising Edge":bool)  [unwired: 1 in, 2 out]
    n20 = call "Arduino Interfacing VI.vi"("AE Mode"=Arduino_Interfacing."Read From Arduino") -> ("error out"=w82:errorcluster, "Arduino Data"=w84:T7)  [unwired: 3 in]
    "Arduino Data" <- w84
    n21 = And(x=w70, y="Green LED") -> (x .and. y?=w73:bool)
    n22 = call <vilib>:"DIO Write.vi"("error in (no error)"=w92, "Input"=w73, "DIO Info In"=w93) -> ("error out"=w76:errorcluster, "DIO Info Out"=w91:T22)  [unwired: 7 in]
    n23 = Unbundle By Name(w84) -> ("Rotary Switch"=→"Task selection":u8)
    n24 = call "navX reading VI.vi"("NavX Info In"=w100, "Mode"=navX_type_def."Get i2C reference", "error in (no error)"=w98) -> ("NavX Info Out"=w89:T27, "Error Out"=w78:errorcluster)  [unwired: 2 out]
    n25 = call "navX reading VI.vi"("NavX Info In"=w89, "Mode"=navX_type_def."Read Values", "error in (no error)"=w78) -> ("NavX Info Out"=w88:T27, "NavX Readings"=→"NavX Readings":T6, "Status"=→"Status":T3, "Error Out"=w87:errorcluster)
    n26 = Merge Errors(w82, w81, w80, w79, w78, w77, w76) -> (w74:errorcluster)
    "General Errors" <- w74
    n27 = call "FGV Bool.vi"("Init/Read/Write State"=States_for_Action_Engine."Read") -> ("Output node"=w114:bool)  [unwired: 2 in, 1 out]
    n28 = Unbundle By Name(w74) -> ("status"=w71:bool)
    n29 = Wait (ms)(milliseconds to wait=u32 20) -> ()  [unwired: 1 out]
    n30 = local write "Red LED"(w71) -> ()
  }
  n31 = while {
    tunnel: w59 -> [w132]
    tunnel: w60 -> [w131]
    tunnel: [w130] -> w66
    tunnel: [w129] -> w65
    tunnel: w64 -> [w128]
    tunnel: [w127] -> w62
    tunnel: w63 -> [w126]
    tunnel: [w125] -> w61
    stop <- w123 stop-if-true
    # "Generate USER Event Loop"
    n32 = local read "Rising Edge"() -> (w120:bool)
    n33 = Or(x="OK Button", y=w120) -> (x .or. y?=w119:bool)
    n34 = local read "TASK ENABLE"() -> (w118:bool)
    n35 = And(x=w119, y=w118) -> (x .and. y?=w117:bool)
    n36 = case shown="True" w117 {
      selector: w117 -> [_ w143]
      tunnel: w132 -> [w142 w147]
      tunnel: [w142 w146] -> w129
      tunnel: w128 -> [w141 w145]
      tunnel: [w141 w144] -> w127
      frame False {
      }
      frame True {
        n37 = Generate User Event(user event=w147, event data cluster=w143, error in=w145) -> (user event out=w146:refnum<user-event>, error out=w144:errorcluster)  [unwired: 1 in]
      }
    }
    n38 = case shown="False" "STOP" {
      selector: "STOP" -> [_ w136]
      tunnel: w131 -> [w135 w140]
      tunnel: [w135 w139] -> w130
      tunnel: w126 -> [w134 w138]
      tunnel: [w134 w137] -> w125
      tunnel: [FALSE w136] -> w123
      frame False {
      }
      frame True {
        n39 = Generate User Event(user event=w140, event data cluster=w136, error in=w138) -> (user event out=w139:refnum<user-event>, error out=w137:errorcluster)  [unwired: 1 in]
      }
    }
    n40 = Wait (ms)(milliseconds to wait=u32 10) -> ()  [unwired: 1 out]
    n41 = call "FGV Bool.vi"("Init/Read/Write State"=States_for_Action_Engine."Write", "Input Node"=w123) -> ()  [unwired: 1 in, 2 out]
  }
  n42 = while {
    tunnel: w58 -> [w154]
    tunnel: [w153] -> w57
    tunnel: w45 -> [w151]
    tunnel: [w150] -> w56
    tunnel: w51 -> [w149]
    tunnel: [w148] -> w48
    stop <- w152 stop-if-true
    # "EVENT Handling Loop"
    n43 = event shown="[1] <Start Task>: User Event" {
      selector: w154 -> [_ _ _]
      dyn-events: [_ _ _] -> w153
      timeout: _ -> [_ _ _]
      tunnel: [FALSE FALSE w185] -> w152
      tunnel: w151 -> [w159 w168 w183]
      tunnel: [w158 w167 w184] -> w150
      tunnel: w149 -> [w157 w166 w182]
      tunnel: [w156 w165 w181] -> w148
      event Timeout {
        n44 = event-data() -> ()  [unwired: 1 in, 3 out]
        n45 = Enqueue Element(queue=w159, element=Intruction_Type_Definitions."None" ("Enum"), error in (no error)=w157) -> (queue out=w158:refnum<queue>, error out=w156:errorcluster)  [unwired: 1 in, 1 out]
      }
      event User Event {
        n46 = event-data() -> ()  [unwired: 1 in, 5 out]
        n47 = call "Arduino Interfacing VI.vi"("AE Mode"=Arduino_Interfacing."Read From Arduino") -> ("Arduino Data"=w162:T7)  [unwired: 3 in, 1 out]
        n48 = Unbundle By Name(w162) -> ("Rotary Switch"=w161:u8)
        n49 = case shown="10" w161 {
          tunnel: [Intruction_Type_Definitions."None" ("Enum") Intruction_Type_Definitions."Start Task 1" ("Enum") Intruction_Type_Definitions."Start Task 2" ("Enum") Intruction_Type_Definitions."Start Task 3" ("Enum") Intruction_Type_Definitions."Start Task 4" ("Enum") Intruction_Type_Definitions."Start Task 5" ("Enum") Intruction_Type_Definitions."Start Task 6" ("Enum") Intruction_Type_Definitions."Start Task 8" ("Enum") Intruction_Type_Definitions."Start Task 9" ("Enum") Intruction_Type_Definitions."Start Task A" ("Enum")] -> w164
          frame 0, Default {
          }
          frame 1 {
          }
          frame 2 {
          }
          frame 3 {
          }
          frame 4 {
          }
          frame 5 {
          }
          frame 6 {
          }
          frame 8 {
          }
          frame 9 {
          }
          frame 10 {
          }
        }
        n50 = Enqueue Element(queue=w168, element=w164, error in (no error)=w166) -> (queue out=w167:refnum<queue>, error out=w165:errorcluster)  [unwired: 1 in, 1 out]
      }
      event User Event {
        n51 = event-data() -> ("Stop Queue"=w185:bool)  [unwired: 1 in, 4 out]
        n52 = Enqueue Element At Opposite End(queue=w183, element=Intruction_Type_Definitions."Exit" ("Enum"), error in (no error)=w182) -> (queue out=w184:refnum<queue>, error out=w181:errorcluster)  [unwired: 1 in, 1 out]
      }
    }
  }
  n53 = while {
    tunnel: w46 -> [w195]
    tunnel: w45 -> [w192]
    stop <- w189 stop-if-true
    # "Status Loop for Action Queues"
    n54 = Get Queue Status(queue=w195, return elements? (F)=TRUE) -> (error out=w191:errorcluster, # elements in queue=→"Action Queue Items":i32, elements=→"Action Queues items":string[])  [unwired: 1 in, 5 out]
    n55 = Get Queue Status(queue=w192, return elements? (F)=TRUE) -> (# pending remove=→"State Logic Queue Items":i32, error out=w190:errorcluster, elements=→"elements":T10[])  [unwired: 1 in, 5 out]
    n56 = Merge Errors(w191, w190) -> (w189:errorcluster)
    n57 = Wait (ms)(milliseconds to wait=u32 500) -> ()  [unwired: 1 out]
  }
  n58 = while {
    tunnel: w45 -> [w235]
    tunnel: w46 -> [w247]
    tunnel: w49 -> [w245]
    tunnel: [w244] -> _
    tunnel: [w243] -> w39
    shift-right: [w236] -> _
    shift-left: T20 {"PING_A"=0, "PING_B"=0, "PING_C"=0, "PING_D"=0} -> [w238]
    shift-right: [w229] -> _
    shift-left: State_Type_Definitions."Startup" ("Enum") -> [w232]
    shift-right: [w225] -> _
    shift-left: T21 {"xDistance"=0.0, "yDistance"=0.0, "wDistance"=0.0} -> [w227]
    shift-right: [w222] -> _
    shift-left: _ -> [w221]
    shift-right: [w218] -> _
    shift-left: T19 {"Recognized Object"=FALSE, "Object X coordinate"=0.0, "Object Y coordinate"=0.0} -> [w220]
    shift-right: [w215] -> _
    shift-left: T17 {"y Stepper Position"=0, "z Stepper Position"=0} -> [w217]
    shift-right: [w212] -> _
    shift-left: T16 {"Yaw"=0.0, "Compass"=0.0} -> [w214]
    shift-right: [w209] -> _
    shift-left: T15 {"Time up flag"=FALSE, "SET TIME TO CHECK"=0.0} -> [w211]
    shift-right: [w207] -> _
    shift-left: T14 {"yStepper desired"=0} -> [w208]
    shift-right: [w203] -> _
    shift-left: T13 {"Left IR Sensor"=0.0, "Arm IR Sensor"=0.0, "Bottom IR Sensor"=0.0} -> [w205]
    shift-right: [w201] -> _
    shift-left: T12 {"ySpeed"=0.0, "xSpeed"=0.0, "wSpeed"=0.0} -> [w202]
    shift-right: [w198] -> _
    shift-left: T11 {"Line Detected?"=FALSE, "S1"=0.0, "S2"=0.0, "S3"=0.0, "S4"=0.0} -> [w200]
    stop <- w234 stop-if-true
    # ">>> Motor control cluster >>>"
    # ">>> yStepper command>>>"
    # ">>True Stop Next State >>"
    # ">>Error  >>"
    # ">>Timeout>>"
    # ">>Action states Queue Reference >>"
    # ">>State Logic Queue Reference >>"
    # "TOP LEVEL BASELINE (MAIN PROCESSING LOOP)"
    n59 = Dequeue Element(queue=w247, timeout in ms (-1)=0, error in (no error)=w245) -> (queue out=w239:refnum<queue>, element=w246:string, error out=w240:errorcluster)  [unwired: 1 out]
    "Action State" <- w246
    n60 = Wait (ms)(milliseconds to wait=u32 20) -> ()  [unwired: 1 out]
    n61 = case shown="\"READ LINE SENSOR\"" w246 {
      tunnel: [_ _ _ _ _ _ _ _ _ _ _ _ _ _ _ _ _ _ _ _ 0 w2354 _ _ _ _ _ _ _ _ _ _ _ _ _ _ _ _ _ _ _ _ _ _ _ _ _ _ _ _ _] -> w242
      tunnel: w239 -> [_ _ _ _ _ _ _ _ _ _ _ _ _ _ _ _ _ _ _ _ _ _ _ _ _ _ _ _ _ _ _ _ _ _ _ _ _ _ _ _ _ _ _ _ _ _ _ _ _ _ _]
      tunnel: w238 -> [w2071 w2081 w2094 w2106 w2124 w2136 w2148 w2161 w2175 w2188 w2200 w2208 w2224 w2239 w2252 w2263 w2285 w2293 w2321 w2332 w2344 w2355 w2365 w2376 w2407 w2419 w2428 w2438 w2449 w2462 w2476 w2486 w2496 w2514 w2523 w2537 w2545 w2556 w2567 w2578 w2586 w2602 w2610 w2627 w2634 w2647 w2660 w2673 w2686 w2699 w2711]
      tunnel: [w2071 w2081 w2094 w2106 w2124 w2136 w2148 w2161 w2175 w2188 w2200 w2208 w2224 w2240 w2252 w2263 w2285 w2293 w2322 w2332 w2344 w2355 w2365 w2376 w2406 w2419 w2428 w2438 w2449 w2462 w2476 w2486 w2496 w2514 w2523 w2537 w2545 w2556 w2567 w2578 w2586 w2602 w2610 w2627 w2634 w2647 w2660 w2673 w2686 w2699 w2711] -> w237
      tunnel: [TRUE TRUE _ _ _ _ _ _ _ _ _ _ _ _ _ _ _ _ _ _ _ _ _ _ _ _ _ _ _ _ _ _ _ _ _ _ _ _ _ _ _ _ _ _ _ _ _ _ _ _ _] -> w234
      tunnel: w232 -> [w2069 w2079 w2093 w2105 w2123 w2135 w2147 w2160 w2174 w2187 w2199 w2207 w2223 w2238 w2251 w2261 w2278 w2292 w2320 w2331 w2341 w2352 w2364 w2375 w2405 w2418 w2427 w2437 w2441 w2461 w2475 w2485 w2495 w2513 w2522 w2531 w2544 w2555 w2566 w2577 w2585 w2593 w2609 w2626 w2633 w2646 w2659 w2672 w2685 w2698 w2710]
      tunnel: [_ _ _ _ _ _ _ _ _ _ _ _ _ _ _ _ _ _ _ _ _ TRUE _ _ _ _ _ _ _ _ _ _ _ _ _ _ _ _ _ _ _ _ _ _ _ _ _ _ _ _ _] -> w231
      tunnel: [w2069 w2079 w2093 w2105 w2123 w2135 w2147 w2160 w2174 w2187 w2199 w2207 w2223 w2238 w2251 w2261 w2278 w2292 w2320 w2331 w2341 w2352 w2364 w2375 w2405 w2418 w2427 w2437 w2441 w2461 w2475 w2485 w2495 w2513 w2522 w2531 w2544 w2555 w2566 w2577 w2585 w2593 w2609 w2626 w2633 w2646 w2659 w2672 w2685 w2698 w2710] -> w230
      tunnel: w227 -> [w2068 w2078 w2092 w2108 w2122 w2134 w2146 w2159 w2173 w2186 w2198 w2209 w2222 w2237 w2253 w2265 w2280 w2294 w2319 w2333 w2340 w2351 w2366 w2377 w2395 w2417 w2430 w2439 w2446 w2463 w2477 w2487 w2497 w2515 w2525 w2535 w2547 w2558 w2569 w2580 w2588 w2597 w2612 w2629 w2636 w2649 w2662 w2675 w2688 w2701 w2713]
      tunnel: [w2068 w2078 w2092 w2108 w2122 w2134 w2146 w2159 w2173 w2186 w2198 w2209 w2221 w2237 w2253 w2265 w2280 w2294 w2318 w2333 w2340 w2351 w2366 w2377 w2394 w2417 w2430 w2439 w2446 w2463 w2477 w2487 w2497 w2515 w2525 w2535 w2547 w2558 w2569 w2580 w2588 w2597 w2612 w2629 w2636 w2649 w2662 w2675 w2688 w2701 w2713] -> w226
      tunnel: w220 -> [w2067 w2077 w2091 w2107 w2121 w2133 w2145 w2158 w2172 w2185 w2196 w2206 w2220 w2236 w2246 w2264 w2279 w2291 w2310 w2330 w2339 w2350 w2363 w2374 w2400 w2415 w2429 w2436 w2447 w2460 w2474 w2481 w2494 w2508 w2524 w2536 w2546 w2557 w2568 w2579 w2587 w2596 w2611 w2628 w2635 w2648 w2661 w2674 w2687 w2700 w2712]
      tunnel: [w2067 w2077 w2091 w2107 w2121 w2133 w2145 w2158 w2172 w2185 w2196 w2206 w2220 w2236 w2246 w2264 w2279 w2291 w2309 w2330 w2339 w2350 w2363 w2374 w2399 w2415 w2429 w2436 w2447 w2460 w2474 w2481 w2494 w2507 w2524 w2536 w2546 w2557 w2568 w2579 w2587 w2596 w2611 w2628 w2635 w2648 w2661 w2674 w2687 w2700 w2712] -> w219
      tunnel: w217 -> [w2066 w2076 w2090 w2109 w2120 w2132 w2144 w2157 w2171 w2184 w2195 w2205 w2219 w2235 w2254 w2266 w2281 w2290 w2315 w2329 w2338 w2349 w2362 w2373 w2390 w2414 w2426 w2435 w2445 w2459 w2473 w2484 w2493 w2516 w2526 w2534 w2543 w2554 w2565 w2576 w2589 w2598 w2613 w2625 w2637 w2650 w2663 w2676 w2689 w2702 w2714]
      tunnel: [w2066 w2076 w2090 w2109 w2120 w2132 w2144 w2157 w2171 w2184 w2195 w2205 w2219 w2235 w2254 w2266 w2281 w2290 w2314 w2329 w2338 w2349 w2362 w2373 w2389 w2414 w2426 w2435 w2445 w2459 w2473 w2484 w2493 w2516 w2526 w2534 w2543 w2554 w2565 w2576 w2589 w2598 w2613 w2624 w2637 w2650 w2663 w2676 w2689 w2702 w2714] -> w216
      tunnel: w214 -> [w2065 w2075 w2088 w2110 w2118 w2130 w2143 w2155 w2169 w2182 w2194 w2204 w2218 w2228 w2249 w2267 w2282 w2289 w2305 w2328 w2337 w2348 w2361 w2372 w2386 w2413 w2423 w2434 w2444 w2458 w2472 w2483 w2492 w2517 w2527 w2533 w2542 w2551 w2562 w2573 w2590 w2599 w2614 w2619 w2638 w2651 w2664 w2677 w2690 w2703 w2715]
      tunnel: [w2065 w2075 w2088 w2110 w2118 w2130 w2143 w2155 w2169 w2182 w2194 w2204 w2218 w2228 w2248 w2267 w2282 w2289 w2304 w2328 w2337 w2348 w2361 w2372 w2385 w2413 w2423 w2434 w2444 w2458 w2472 w2483 w2492 w2517 w2527 w2533 w2542 w2551 w2562 w2573 w2590 w2599 w2614 w2619 w2638 w2651 w2664 w2677 w2690 w2703 w2715] -> w213
      tunnel: w211 -> [w2063 w2074 w2089 w2111 w2119 w2131 w2142 w2156 w2170 w2183 w2193 w2203 w2217 w2227 w2245 w2268 w2283 w2288 w2301 w2325 w2336 w2347 w2360 w2371 w2383 w2411 w2422 w2433 w2443 w2457 w2471 w2482 w2491 w2518 w2528 w2532 w2541 w2550 w2561 w2572 w2591 w2600 w2615 w2618 w2632 w2645 w2658 w2671 w2684 w2697 w2709]
      tunnel: [w2063 w2074 w2089 w2111 w2119 w2131 w2142 w2156 w2170 w2183 w2193 w2203 w2217 w2227 w2245 w2268 w2283 w2288 w2301 w2325 w2336 w2347 w2360 w2371 w2382 w2411 w2422 w2433 w2443 w2457 w2471 w2482 w2491 w2518 w2528 w2532 w2541 w2550 w2561 w2572 w2591 w2600 w2615 w2618 w2632 w2643 w2656 w2669 w2682 w2695 w2708] -> w210
      tunnel: w208 -> [_ _ _ _ _ _ _ _ _ _ _ _ _ _ _ _ _ _ _ _ _ _ _ _ _ _ _ _ _ _ _ _ _ _ _ _ _ _ _ _ _ _ w2606 _ _ _ _ _ _ _ _]
      tunnel: [w2062 w2073 w2083 w2101 w2113 w2126 w2138 w2150 w2165 w2177 w2190 w2202 w2211 w2226 w2242 w2259 w2284 w2287 w2298 w2324 w2335 w2346 w2359 w2368 w2379 w2410 w2421 w2432 w2448 w2451 w2465 w2479 w2489 w2501 w2520 w2538 w2540 w2549 w2560 w2571 w2582 w2601 w2604 w2617 w2631 w2640 w2653 w2666 w2679 w2692 w2705] -> w204
      tunnel: w205 -> [w2062 w2073 w2083 w2101 w2113 w2126 w2138 w2150 w2165 w2177 w2190 w2202 w2211 w2226 w2242 w2260 w2284 w2287 w2298 w2324 w2335 w2346 w2359 w2368 w2379 w2410 w2421 w2432 w2448 w2451 w2465 w2479 w2489 w2501 w2520 w2538 w2540 w2549 w2560 w2571 w2582 w2601 w2604 w2617 w2631 w2640 w2653 w2666 w2679 w2692 w2705]
      tunnel: w202 -> [_ _ _ _ _ _ _ _ w2164 _ _ _ _ _ _ _ _ _ _ _ _ _ _ _ _ _ _ _ _ _ _ _ _ _ _ _ _ _ _ _ _ _ _ _ _ _ _ _ _ _ _]
      tunnel: w200 -> [w2061 w2072 w2082 w2095 w2112 w2125 w2137 w2149 w2162 w2176 w2189 w2201 w2210 w2225 w2241 w2255 w2277 w2286 w2296 w2323 w2334 w2345 w2358 w2367 w2378 w2409 w2420 w2431 w2440 w2450 w2464 w2478 w2488 w2498 w2519 w2529 w2539 w2548 w2559 w2570 w2581 w2592 w2603 w2616 w2630 w2639 w2652 w2665 w2678 w2691 w2704]
      tunnel: [w2061 w2072 w2082 w2095 w2112 w2125 w2137 w2149 w2162 w2176 w2189 w2201 w2210 w2225 w2241 w2255 w2276 w2286 w2296 w2323 w2334 w2345 w2358 w2367 w2378 w2409 w2420 w2431 w2440 w2450 w2464 w2478 w2488 w2498 w2519 w2529 w2539 w2548 w2559 w2570 w2581 w2592 w2603 w2616 w2630 w2639 w2652 w2665 w2678 w2691 w2704] -> w199
      frame "Exit" {
        # ">>State Logic  >>"
        # ">>> Time cluster >>>"
        # ">>> Yaw >>>"
        # ">>> Stepper position >>>"
        # ">>> Encoders >>>"
        # ">>> Object detection >>>"
        # ">>> Ultrasonic Sensors Detect >>>"
        n62 = call "Imaq Dispose"("All Images? (No)"=TRUE) -> ()  [unwired: 5 in, 1 out]
      }
      frame "----Movement States----" {
        # ">>State Logic  >>"
        # ">>> Time cluster >>>"
        # ">>> Yaw >>>"
        # ">>> Stepper position >>>"
        # ">>> Encoders >>>"
        # ">>> Object detection >>>"
        # ">>> Ultrasonic Sensors Detect >>>"
      }
      frame "FORWARD" {
        # ">>State Logic  >>"
        # ">>> Time cluster >>>"
        # ">>> Yaw >>>"
        # ">>> Stepper position >>>"
        # ">>> Encoders >>>"
        # ">>> Object detection >>>"
        # ">>> Ultrasonic Sensors Detect >>>"
        n63 = Unbundle By Name(w2088) -> ("Yaw"=w2084:dbl)
        n64 = call "MOTOR CONTROL WITH PID AE.vi"("Yaw"=w2084, "Speed"=50.0, "Direction"=MOTOR_CONTROL_WITH_PID_AE_DIRECTION_TYPE_DEF."y-axis movement", "AE Mode"=MOTOR_CONTROL_WITH_PID_AE_DATA_MODE_TYPE_DEF."Write to AE") -> ()  [unwired: 1 out]
      }
      frame "FORWARD - IR ASSIST" {
        # ">>State Logic  >>"
        # ">>> Time cluster >>>"
        # ">>> Yaw >>>"
        # ">>> Stepper position >>>"
        # ">>> Encoders >>>"
        # ">>> Object detection >>>"
        # ">>> Ultrasonic Sensors Detect >>>"
        n65 = Unbundle By Name(w2101) -> ("Left IR Sensor"=w2100:dbl)
        n66 = Subtract(x=w2100, y=15.0) -> (x-y=w2098:dbl)
        n67 = Multiply(x=w2098, y=0.5) -> (x*y=w2096:dbl)
        n68 = call "MOTOR CONTROL WITH PID AE.vi"("Yaw"=w2096, "Speed"=30.0, "Direction"=MOTOR_CONTROL_WITH_PID_AE_DIRECTION_TYPE_DEF."y-axis movement", "AE Mode"=MOTOR_CONTROL_WITH_PID_AE_DATA_MODE_TYPE_DEF."Write to AE") -> ()  [unwired: 1 out]
      }
      frame "LEFT" {
        # ">>State Logic  >>"
        # ">>> Time cluster >>>"
        # ">>> Yaw >>>"
        # ">>> Stepper position >>>"
        # ">>> Encoders >>>"
        # ">>> Object detection >>>"
        # ">>> Ultrasonic Sensors Detect >>>"
        n69 = Unbundle By Name(w2118) -> ("Yaw"=w2115:dbl)
        n70 = call "MOTOR CONTROL WITH PID AE.vi"("Yaw"=w2115, "Speed"=-25.0, "Direction"=MOTOR_CONTROL_WITH_PID_AE_DIRECTION_TYPE_DEF."x-axis movement", "AE Mode"=MOTOR_CONTROL_WITH_PID_AE_DATA_MODE_TYPE_DEF."Write to AE") -> ()  [unwired: 1 out]
      }
      frame "R-ACW" {
        # ">>> IR Sensors >>>"
        # ">>> Time cluster >>>"
        # ">>> Yaw >>>"
        # ">>> Stepper position >>>"
        # ">>> Encoders >>>"
        # ">>> Object detection >>>"
        # ">>> Ultrasonic Sensors Detect >>>"
        n71 = call "MOTOR CONTROL WITH PID AE.vi"("Speed"=-10.0, "Direction"=MOTOR_CONTROL_WITH_PID_AE_DIRECTION_TYPE_DEF."rotation", "AE Mode"=MOTOR_CONTROL_WITH_PID_AE_DATA_MODE_TYPE_DEF."Write to AE") -> ()  [unwired: 1 in, 1 out]
      }
      frame "R-CW" {
        (unwired) -0.2 ("Speed")
        # ">>> Time cluster >>>"
        # ">>> Yaw >>>"
        # ">>> Stepper position >>>"
        # ">>> Encoders >>>"
        # ">>> Object detection >>>"
        # ">>> Ultrasonic Sensors Detect >>>"
        n72 = call "MOTOR CONTROL WITH PID AE.vi"("Speed"=10.0, "Direction"=MOTOR_CONTROL_WITH_PID_AE_DIRECTION_TYPE_DEF."rotation", "AE Mode"=MOTOR_CONTROL_WITH_PID_AE_DATA_MODE_TYPE_DEF."Write to AE") -> ()  [unwired: 1 in, 1 out]
      }
      frame "RIGHT" {
        # ">>> Time cluster >>>"
        # ">>> Yaw >>>"
        # ">>> Stepper position >>>"
        # ">>> Encoders >>>"
        # ">>> Object detection >>>"
        # ">>> Ultrasonic Sensors Detect >>>"
        n73 = Unbundle By Name(w2155) -> ("Yaw"=w2151:dbl)
        n74 = call "MOTOR CONTROL WITH PID AE.vi"("Yaw"=w2151, "Speed"=50.0, "Direction"=MOTOR_CONTROL_WITH_PID_AE_DIRECTION_TYPE_DEF."x-axis movement", "AE Mode"=MOTOR_CONTROL_WITH_PID_AE_DATA_MODE_TYPE_DEF."Write to AE") -> ()  [unwired: 1 out]
      }
      frame "X AXIS - SLOW" {
        # ">>> IR Sensors >>>"
        # ">>> Time cluster >>>"
        # ">>> Yaw >>>"
        # ">>> Stepper position >>>"
        # ">>> Encoders >>>"
        # ">>> Object detection >>>"
        # ">>> Ultrasonic Sensors Detect >>>"
        n75 = Unbundle By Name(w2164) -> ("xSpeed"=w2163:dbl)
        n76 = Unbundle By Name(w2169) -> ("Yaw"=w2166:dbl)
        n77 = call "MOTOR CONTROL WITH PID AE.vi"("Yaw"=w2166, "Speed"=w2163, "Direction"=MOTOR_CONTROL_WITH_PID_AE_DIRECTION_TYPE_DEF."x-axis movement", "AE Mode"=MOTOR_CONTROL_WITH_PID_AE_DATA_MODE_TYPE_DEF."Write to AE") -> ()  [unwired: 1 out]
      }
      frame "REVERSE" {
        # ">>> Time cluster >>>"
        # ">>> Yaw >>>"
        # ">>> Stepper position >>>"
        # ">>> Encoders >>>"
        # ">>> Object detection >>>"
        # ">>> Ultrasonic Sensors Detect >>>"
        n78 = Unbundle By Name(w2182) -> ("Yaw"=w2178:dbl)
        n79 = call "MOTOR CONTROL WITH PID AE.vi"("Yaw"=w2178, "Speed"=-50.0, "Direction"=MOTOR_CONTROL_WITH_PID_AE_DIRECTION_TYPE_DEF."y-axis movement", "AE Mode"=MOTOR_CONTROL_WITH_PID_AE_DATA_MODE_TYPE_DEF."Write to AE") -> ()  [unwired: 1 out]
      }
      frame "STOP" {
        n80 = Wait (ms)(milliseconds to wait=u32 100) -> ()  [unwired: 1 out]
        n81 = call "MOTOR CONTROL WITH PID AE.vi"("Direction"=MOTOR_CONTROL_WITH_PID_AE_DIRECTION_TYPE_DEF."stop", "AE Mode"=MOTOR_CONTROL_WITH_PID_AE_DATA_MODE_TYPE_DEF."Write to AE") -> ()  [unwired: 2 in, 1 out]
      }
      frame "----SENSOR READING---- " {
      }
      frame "READ ENCODERS" {
        # ">>> Time cluster >>>"
        # ">>> Yaw >>>"
        # ">>> Stepper position >>>"
        # ">>> Object detection >>>"
        # ">>> Current encoder distance >>>"
        # ">>> Ultrasonic Sensors Detect >>>"
        n82 = call "MOTOR CONTROL WITH PID AE.vi"("AE Mode"=MOTOR_CONTROL_WITH_PID_AE_DATA_MODE_TYPE_DEF."Read from AE") -> ("Speed & distance"=w2215:T4)  [unwired: 3 in]
        n83 = Unbundle By Name(w2215) -> ("xDistance"=w2214:dbl, "yDistance"=w2213:dbl, "wDistance"=w2212:dbl)
        n84 = Bundle By Name(cluster=w2222, "xDistance"=w2214, "yDistance"=w2213, "wDistance"=w2212) -> (w2221:T21)
      }
      frame "READ ULTRASONIC" {
        (unwired) navX_type_def."Read Values" ("Mode")
        (unwired) MOTOR_CONTROL_NO_PID_Type_Def."Latch" ("Direction")
        # ">>State Logic  >>"
        # ">>> Time cluster >>>"
        # ">>> Ultrasonic Sensors Detect >>>"
        # ">>> Object detection >>>"
        # ">>> Encoders >>>"
        # ">>> Stepper position >>>"
        # ">>> Yaw >>>"
        n85 = call "Arduino Interfacing VI.vi"("AE Mode"=Arduino_Interfacing."Read From Arduino") -> ("Arduino Data"=w2233:T7)  [unwired: 3 in, 1 out]
        n86 = Unbundle By Name(w2233) -> ("PING A"=w2232:u8, "PING B"=w2231:u8, "PING C"=w2230:u8, "PING D"=w2229:u8)
        n87 = Bundle By Name(cluster=w2239, "PING_A"=w2232, "PING_B"=w2231, "PING_C"=w2230, "PING_D"=w2229) -> (w2240:T20)
      }
      frame "READ NAVX" {
        # ">>> Time cluster >>>"
        # ">>> Yaw >>>"
        # ">>> Ultrasonic Sensors Detect >>>"
        # ">>> Object detection >>>"
        # ">>> Encoders >>>"
        # ">>> Stepper position >>>"
        n88 = call "navX reading VI.vi"("Mode"=navX_type_def."Read Values") -> ("NavX Readings"=w2244:T6)  [unwired: 2 in, 3 out]
        n89 = Unbundle By Name(w2244) -> ("Heading"=w2243:dbl)
        n90 = Unbundle By Name(w2244) -> ("Yaw"=w2247:dbl)
        n91 = Bundle By Name(cluster=w2249, "Yaw"=w2247, "Compass"=w2243) -> (w2248:T16)
      }
      frame "READ IR" {
        w2257 = T41 [enum."B/AI1"] items=["Not Connected", "AudioIn/Left", "AudioIn/Right", "C/AI0", "C/AI1", "A/AI0", "A/AI1", "A/AI2", "A/AI3", "A/AI4", "A/AI5", "A/AI6", "A/AI7", "B/AI0", "B/AI1", "B/AI2", "B/AI3", "B/AI4", "B/AI5", "B/AI6", "B/AI7", "AI/AI0", "AI/AI1", "AI/AI2", "AI/AI3", "A/AI0 (DIFF)", "A/AI1 (DIFF)", "A/AI2 (DIFF)", "A/AI3 (DIFF)", "B/AI0 (DIFF)", "B/AI1 (DIFF)", "B/AI2 (DIFF)", "B/AI3 (DIFF)"] ("AI Channel")
        w2262 = T41 [enum."B/AI0"] items=["Not Connected", "AudioIn/Left", "AudioIn/Right", "C/AI0", "C/AI1", "A/AI0", "A/AI1", "A/AI2", "A/AI3", "A/AI4", "A/AI5", "A/AI6", "A/AI7", "B/AI0", "B/AI1", "B/AI2", "B/AI3", "B/AI4", "B/AI5", "B/AI6", "B/AI7", "AI/AI0", "AI/AI1", "AI/AI2", "AI/AI3", "A/AI0 (DIFF)", "A/AI1 (DIFF)", "A/AI2 (DIFF)", "A/AI3 (DIFF)", "B/AI0 (DIFF)", "B/AI1 (DIFF)", "B/AI2 (DIFF)", "B/AI3 (DIFF)"] ("AI Channel")
        # ">>State Logic  >>"
        # ">>> Time cluster >>>"
        # ">>> Ultrasonic Sensors Detect >>>"
        # ">>> Object detection >>>"
        # ">>> Encoders >>>"
        # ">>> Stepper position >>>"
        # ">>> Yaw >>>"
        n92 = call <vilib>:"Sharp IR.vi"("AI Channel"=w2262) -> ("Sharp IR Distance"=w2258:dbl)  [unwired: 8 in, 2 out]
        n93 = call <vilib>:"Sharp IR.vi"("AI Channel"=w2257) -> ("Sharp IR Distance"=w2256:dbl)  [unwired: 8 in, 2 out]
        n94 = Bundle By Name(cluster=w2260, "Left IR Sensor"=w2258, "Arm IR Sensor"=w2256) -> (w2259:T13)
      }
      frame "READ LINE SENSOR" {
        # ">>> IR Sensors >>>"
        # ">>> Line Sensor Cluster>>>"
        # ">>State Logic  >>"
        # ">>> Time cluster >>>"
        # ">>> Object detection >>>"
        # ">>> Yaw >>>"
        # ">>> Ultrasonic Sensors Detect >>>"
        # ">>> Encoders >>>"
        # ">>> Stepper position >>>"
        n95 = call "Line Sensor AE.vi"("AE State"=Line_Sensor_AE_Type_Def."READ FROM LINE SENSORS") -> ("Line Detected?"=w2274:bool, "Line Sensor Raw Values"=w2273:T43)
        n96 = Unbundle By Name(w2273) -> ("S1"=w2272:dbl, "S2"=w2271:dbl, "S3"=w2270:dbl, "S4"=w2269:dbl)
        n97 = Bundle By Name(cluster=w2277, "Line Detected?"=w2274, "S1"=w2272, "S2"=w2271, "S3"=w2270, "S4"=w2269) -> (w2276:T11)
      }
      frame "----SYSTEM MODES----" {
        (unwired) I2C_MASTER_Type_Def."Last State" ("Arduino Mode")
        # ">>> Object detection >>>"
        # ">>> Yaw >>>"
        # ">>> Ultrasonic Sensors Detect >>>"
        # ">>> Encoders >>>"
        # ">>> Stepper position >>>"
      }
      frame "INIT" {
        w2316 = u8 0
        w2317 = 0.0
        # ">>> IR Sensors >>>"
        # ">>> IR Sensors >>>"
        # ">>> Line Sensor Cluster>>>"
        # ">>> Time cluster >>>"
        # ">>> Object detection >>>"
        # ">>> Yaw >>>"
        # ">>> Ultrasonic Sensors Detect >>>"
        # ">>> Encoders >>>"
        # ">>> Stepper position >>>"
        # ">>State Logic  >>"
        n98 = call "Arduino Interfacing VI.vi"("AE Mode"=Arduino_Interfacing."Initialize") -> ()  [unwired: 3 in, 2 out]
        n99 = call "FGV Bool.vi"("Init/Read/Write State"=States_for_Action_Engine."Initialize") -> ()  [unwired: 2 in, 2 out]
        n100 = call "Elasped Timer.vi"("Action"=Elapsed_timer_control."Initialize") -> ()  [unwired: 7 in, 4 out]
        n101 = call "MOTOR CONTROL WITH PID AE.vi"("AE Mode"=MOTOR_CONTROL_WITH_PID_AE_DATA_MODE_TYPE_DEF."Init AE") -> ()  [unwired: 3 in, 1 out]
        n102 = call "IMAQ Reference AE.vi"("IMAQ AE States"=IMAQ_Reference_AE."Initialize AE") -> ()  [unwired: 1 in, 2 out]
        n103 = call "Line Sensor AE.vi"("AE State"=Line_Sensor_AE_Type_Def."INIT AE") -> ()  [unwired: 2 out]
        n104 = Bundle By Name(cluster=w2310, "Recognized Object"=FALSE, "Object X coordinate"=0.0, "Object Y coordinate"=0.0) -> (w2309:T19)
        n105 = Bundle By Name(cluster=w2315, "y Stepper Position"=u8 0, "z Stepper Position"=u8 0) -> (w2314:T17)
        n106 = Bundle By Name(cluster=w2319, "xDistance"=w2317, "yDistance"=w2317, "wDistance"=w2317) -> (w2318:T21)
        n107 = Bundle By Name(cluster=w2321, "PING_A"=w2316, "PING_B"=w2316, "PING_C"=w2316, "PING_D"=w2316) -> (w2322:T20)
        n108 = Bundle By Name(cluster=w2305, "Yaw"=0.0) -> (w2304:T16)
      }
      frame "ARDUINO - ULTRASONIC" {
        # ">>> Time cluster >>>"
        # ">>> Line Sensor Cluster>>>"
        # ">>> Object detection >>>"
        # ">>> Yaw >>>"
        # ">>> Ultrasonic Sensors Detect >>>"
        # ">>> Encoders >>>"
        # ">>> Stepper position >>>"
        # ">>State Logic  >>"
        n109 = call "Arduino Interfacing VI.vi"("Data to Write"=I2C_MASTER_WRITE_NEW_Type_Def."Ultrasonic sensors", "AE Mode"=Arduino_Interfacing."Write to Arduino") -> ()  [unwired: 2 in, 2 out]
      }
      frame "NAVX CALIBRATE" {
        # ">>> Object detection >>>"
        # ">>> Yaw >>>"
        # ">>> Ultrasonic Sensors Detect >>>"
        # ">>> Encoders >>>"
        # ">>> Stepper position >>>"
        # ">>State Logic  >>"
        # "Adds a 15 second delay to the startup process \nfor the NavX to calibrate"
        n110 = Wait (ms)(milliseconds to wait=u32 1000) -> ()  [unwired: 1 out]
      }
      frame "NO ACTION", Default {
        (unwired) u8 0 ("y Stepper value")
        (unwired) TRUE ("Latch")
        (unwired) navX_type_def."Read Values" ("Mode")
        (unwired) MOTOR_CONTROL_NO_PID_Type_Def."Latch" ("Direction")
        # ">>> Object detection >>>"
        # ">>> Yaw >>>"
        # ">>> Ultrasonic Sensors Detect >>>"
        # ">>> Encoders >>>"
        # ">>> Stepper position >>>"
        # ">>State Logic  >>"
        n111 = case shown="4" w2352 {
          tunnel: [0 100] -> w2354
          frame 1, Default {
          }
          frame 4 {
          }
        }
      }
      frame "----RESET CASES----" {
        (unwired) I2C_MASTER_Type_Def."Last State" ("Arduino Mode")
        # ">>> Object detection >>>"
        # ">>> Yaw >>>"
        # ">>> Ultrasonic Sensors Detect >>>"
        # ">>> Encoders >>>"
        # ">>> Stepper position >>>"
        # ">>State Logic  >>"
      }
      frame "RESET ENCODERS" {
        # ">>> Object detection >>>"
        # ">>> Yaw >>>"
        # ">>> Ultrasonic Sensors Detect >>>"
        # ">>> Encoders >>>"
        # ">>> Stepper position >>>"
        # ">>State Logic  >>"
        n112 = call "MOTOR CONTROL WITH PID AE.vi"("Direction"=MOTOR_CONTROL_WITH_PID_AE_DIRECTION_TYPE_DEF."reset encoders", "AE Mode"=MOTOR_CONTROL_WITH_PID_AE_DATA_MODE_TYPE_DEF."Write to AE") -> ()  [unwired: 2 in, 1 out]
      }
      frame "RESET FLAGS" {
        (unwired) I2C_MASTER_Type_Def."Last State" ("Arduino Mode")
        # "Resets any software variables\nand/or non-critical states"
        n113 = Wait (ms)(milliseconds to wait=u32 20) -> ()  [unwired: 1 out]
        n114 = Bundle By Name(cluster=w2383, "Time up flag"=FALSE, "SET TIME TO CHECK"=0.0) -> (w2382:T15)
        n115 = Bundle By Name(cluster=w2400, "Recognized Object"=FALSE, "Object X coordinate"=0.0, "Object Y coordinate"=0.0) -> (w2399:T19)
        n116 = Bundle By Name(cluster=w2390, "y Stepper Position"=u8 0, "z Stepper Position"=u8 0) -> (w2389:T17)
        n117 = Bundle By Name(cluster=w2395, "xDistance"=0.0, "yDistance"=0.0, "wDistance"=0.0) -> (w2394:T21)
        n118 = Bundle By Name(cluster=w2407, "PING_A"=u8 0, "PING_B"=u8 0, "PING_C"=u8 0, "PING_D"=u8 0) -> (w2406:T20)
        n119 = Bundle By Name(cluster=w2386, "Yaw"=0.0) -> (w2385:T16)
      }
      frame "RESET YAW" {
        n120 = Wait (ms)(milliseconds to wait=u32 100) -> ()  [unwired: 1 out]
        n121 = call "navX reading VI.vi"("Mode"=navX_type_def."Zero Yaw") -> ()  [unwired: 2 in, 4 out]
      }
      frame "RESET ARM" {
        n122 = call "Arduino Interfacing VI.vi"("Data to Write"=I2C_MASTER_WRITE_NEW_Type_Def."Soft Reset", "AE Mode"=Arduino_Interfacing."Write to Arduino") -> ()  [unwired: 2 in, 2 out]
      }
      frame "--------CAM STATES-------" {
      }
      frame "OPEN IMAQ REF" {
        # ">>State Logic  >>"
        # ">>> Time cluster >>>"
        # ">>> Object detection >>>"
        # ">>> Yaw >>>"
        # ">>> Ultrasonic Sensors Detect >>>"
        # ">>> Encoders >>>"
        # ">>> Stepper position >>>"
        # ">>> IR Sensors >>>"
        n123 = call "IMAQ Reference AE.vi"("IMAQ AE States"=IMAQ_Reference_AE."Initialize AE") -> ()  [unwired: 1 in, 2 out]
      }
      frame "OPEN LOG CAM" {
        n124 = call "Webcam AE.vi"("Session In"=T37 "cam0", "Camera states"=Webcam_AE."Initialize Camera") -> ("error out"=w2454:errorcluster, "Session Out"=w2453:T37)  [unwired: 1 in, 1 out]
        n125 = call "Webcam AE.vi"("error in (no error)"=w2454, "Session In"=w2453, "Camera states"=Webcam_AE."Open Camera") -> ()  [unwired: 3 out]
      }
      frame "OPEN LIFE CAM" {
        n126 = call "Webcam AE.vi"("Session In"=T37 "cam1", "Camera states"=Webcam_AE."Initialize Camera") -> ("error out"=w2468:errorcluster, "Session Out"=w2467:T37)  [unwired: 1 in, 1 out]
        n127 = call "Webcam AE.vi"("error in (no error)"=w2468, "Session In"=w2467, "Camera states"=Webcam_AE."Open Camera") -> ()  [unwired: 3 out]
      }
      frame "CAM ACQ" {
        # ">>State Logic  >>"
        # ">>> Time cluster >>>"
        # ">>> Yaw >>>"
        # ">>> Stepper position >>>"
        # ">>> Encoders >>>"
        # ">>> Object detection >>>"
        # ">>> Ultrasonic Sensors Detect >>>"
        n128 = call "Webcam AE.vi"("Camera states"=Webcam_AE."Continuous Acquisition") -> ()  [unwired: 2 in, 3 out]
      }
      frame "CAM CLOSE" {
        # ">>State Logic  >>"
        # ">>> Time cluster >>>"
        # ">>> Yaw >>>"
        # ">>> Stepper position >>>"
        # ">>> Encoders >>>"
        # ">>> Object detection >>>"
        # ">>> Ultrasonic Sensors Detect >>>"
        n129 = call "Webcam AE.vi"("Camera states"=Webcam_AE."Close Camera") -> ()  [unwired: 2 in, 3 out]
      }
      frame "PROCESS IMAGE" {
        # ">>State Logic  >>"
        # ">>> Time cluster >>>"
        # ">>> Yaw >>>"
        # ">>> Stepper position >>>"
        # ">>> Encoders >>>"
        # ">>> Object detection >>>"
        # ">>> Ultrasonic Sensors Detect >>>"
        n130 = call "Webcam AE.vi"("Camera states"=Webcam_AE."Retrieve Image") -> ("error out"=w2509:errorcluster, "Image Out"=w2511:T45)  [unwired: 2 in, 1 out]
        n131 = call "IMAQ Reference AE.vi"("IMAQ AE States"=IMAQ_Reference_AE."Get IMAQ Reference") -> ("Image Out"=w2499:T45)  [unwired: 1 in, 1 out]
        n132 = call "Object Detection SubVI.vi"("Error In"=w2509, "Mode"="Object recognition mode", "Image Dest"=w2499, "Image in"=w2511) -> ("Object Center Coordinates"=w2506:cluster{"x":sgl, "y":sgl}, "Object detection cluster"=w2502:T5)  [unwired: 2 out]
        "Object detection cluster" <- w2502
        "Object Center Coordinates" <- w2506
        n133 = Unbundle By Name(w2502) -> ("Object detected?"=w2503:bool)
        n134 = Unbundle By Name(w2506) -> ("x"=w2505:sgl, "y"=w2504:sgl)
        n135 = Bundle By Name(cluster=w2508, "Recognized Object"=w2503, "Object X coordinate"=w2505, "Object Y coordinate"=w2504) -> (w2507:T19)
      }
      frame "DISPOSE BUFFERS" {
        # ">>> Line Sensor Cluster>>>"
        # ">>> IR Sensors >>>"
        # ">>State Logic  >>"
        # ">>> Time cluster >>>"
        # ">>> Yaw >>>"
        # ">>> Stepper position >>>"
        # ">>> Encoders >>>"
        # ">>> Object detection >>>"
        # ">>> Ultrasonic Sensors Detect >>>"
        n136 = call "Webcam AE.vi"("Camera states"=Webcam_AE."Dispose Image Buffers") -> ()  [unwired: 2 in, 3 out]
      }
      frame "DISPOSE ALL BUFFERS" {
        # ">>State Logic  >>"
        # ">>> IR Sensors >>>"
        # ">>> Time cluster >>>"
        # ">>> Object detection >>>"
        # ">>> Yaw >>>"
        # ">>> Ultrasonic Sensors Detect >>>"
        # ">>> Encoders >>>"
        # ">>> Stepper position >>>"
        n137 = call "IMAQ Reference AE.vi"("IMAQ AE States"=IMAQ_Reference_AE."Destroy ALL IMAQ") -> ()  [unwired: 1 in, 2 out]
      }
      frame "-----ARM ACTIONS-----" {
      }
      frame "CLOSE CLAW" {
        n138 = call "Arduino Interfacing VI.vi"("Data to Write"=I2C_MASTER_WRITE_NEW_Type_Def."Close Claw", "AE Mode"=Arduino_Interfacing."Write to Arduino") -> ()  [unwired: 2 in, 2 out]
      }
      frame "OPEN CLAW" {
        n139 = call "Arduino Interfacing VI.vi"("Data to Write"=I2C_MASTER_WRITE_NEW_Type_Def."Open Claw", "AE Mode"=Arduino_Interfacing."Write to Arduino") -> ()  [unwired: 2 in, 2 out]
      }
      frame "Z STEPPER CAM HEIGHT" {
        n140 = call "Arduino Interfacing VI.vi"("Data to Write"=I2C_MASTER_WRITE_NEW_Type_Def."zStepper 6k", "AE Mode"=Arduino_Interfacing."Write to Arduino") -> ()  [unwired: 2 in, 2 out]
      }
      frame "Z STEPPER GRAB HEIGHT" {
        # ">>State Logic  >>"
        # ">>> Time cluster >>>"
        # ">>> Yaw >>>"
        # ">>> Stepper position >>>"
        # ">>> Encoders >>>"
        # ">>> Object detection >>>"
        # ">>> Ultrasonic Sensors Detect >>>"
        n141 = call "Arduino Interfacing VI.vi"("Data to Write"=I2C_MASTER_WRITE_NEW_Type_Def."zStepper 100", "AE Mode"=Arduino_Interfacing."Write to Arduino") -> ()  [unwired: 2 in, 2 out]
      }
      frame "Z STEPPER BOX HEIGHT" {
        # ">>> IR Sensors >>>"
        # ">>> Time cluster >>>"
        # ">>> Yaw >>>"
        # ">>> Stepper position >>>"
        # ">>> Encoders >>>"
        # ">>> Object detection >>>"
        # ">>> Ultrasonic Sensors Detect >>>"
        n142 = call "Arduino Interfacing VI.vi"("Data to Write"=I2C_MASTER_WRITE_NEW_Type_Def."zStepper 4k", "AE Mode"=Arduino_Interfacing."Write to Arduino") -> ()  [unwired: 2 in, 2 out]
      }
      frame "Y STEPPER CONTROL" {
        # ">>State Logic  >>"
        # ">>> yStepper command>>>"
        # ">>> Time cluster >>>"
        # ">>> Yaw >>>"
        # ">>> Stepper position >>>"
        # ">>> Encoders >>>"
        # ">>> Object detection >>>"
        # ">>> Ultrasonic Sensors Detect >>>"
        n143 = Unbundle By Name(w2606) -> ("yStepper desired"=w2605:u8)
        n144 = call "Arduino Interfacing VI.vi"("y Stepper value"=w2605, "Data to Write"=I2C_MASTER_WRITE_NEW_Type_Def."yStepper control", "AE Mode"=Arduino_Interfacing."Write to Arduino") -> ()  [unwired: 1 in, 2 out]
      }
      frame "READ STEPPER VALUES" {
        # ">>State Logic  >>"
        # ">>> Time cluster >>>"
        # ">>> Yaw >>>"
        # ">>> Stepper position >>>"
        # ">>> Encoders >>>"
        # ">>> Object detection >>>"
        # ">>> Ultrasonic Sensors Detect >>>"
        n145 = call "Arduino Interfacing VI.vi"("AE Mode"=Arduino_Interfacing."Read From Arduino") -> ("Arduino Data"=w2622:T7)  [unwired: 3 in, 1 out]
        n146 = Unbundle By Name(w2622) -> ("y Stepper Position"=w2621:u8, "z Stepper Position"=w2620:u8)
        n147 = Bundle By Name(cluster=w2625, "y Stepper Position"=w2621, "z Stepper Position"=w2620) -> (w2624:T17)
      }
      frame " -----TIMING-----" {
        # ">>State Logic  >>"
        # ">>> Time cluster >>>"
        # ">>> Yaw >>>"
        # ">>> Stepper position >>>"
        # ">>> Encoders >>>"
        # ">>> Object detection >>>"
        # ">>> Ultrasonic Sensors Detect >>>"
      }
      frame "SET TIMER 1" {
        # ">>State Logic  >>"
        # ">>> Time cluster >>>"
        # ">>> Yaw >>>"
        # ">>> Stepper position >>>"
        # ">>> Encoders >>>"
        # ">>> Object detection >>>"
        # ">>> Ultrasonic Sensors Detect >>>"
        n148 = call "Elasped Timer.vi"("Time Setting"=1.0, "Action"=Elapsed_timer_control."Initialize") -> ()  [unwired: 6 in, 4 out]
        n149 = Bundle By Name(cluster=w2645, "Time up flag"=FALSE) -> (w2643:T15)
      }
      frame "SET TIMER 2" {
        # ">>State Logic  >>"
        # ">>> Time cluster >>>"
        # ">>> Yaw >>>"
        # ">>> Stepper position >>>"
        # ">>> Encoders >>>"
        # ">>> Object detection >>>"
        # ">>> Ultrasonic Sensors Detect >>>"
        n150 = call "Elasped Timer.vi"("Time Setting"=2.0, "Action"=Elapsed_timer_control."Initialize") -> ()  [unwired: 6 in, 4 out]
        n151 = Bundle By Name(cluster=w2658, "Time up flag"=FALSE) -> (w2656:T15)
      }
      frame "SET TIMER 3" {
        # ">>State Logic  >>"
        # ">>> Time cluster >>>"
        # ">>> Yaw >>>"
        # ">>> Stepper position >>>"
        # ">>> Encoders >>>"
        # ">>> Object detection >>>"
        # ">>> Ultrasonic Sensors Detect >>>"
        n152 = call "Elasped Timer.vi"("Time Setting"=3.0, "Action"=Elapsed_timer_control."Initialize") -> ()  [unwired: 6 in, 4 out]
        n153 = Bundle By Name(cluster=w2671, "Time up flag"=FALSE) -> (w2669:T15)
      }
      frame "SET TIMER 4" {
        # ">>State Logic  >>"
        # ">>> Time cluster >>>"
        # ">>> Yaw >>>"
        # ">>> Stepper position >>>"
        # ">>> Encoders >>>"
        # ">>> Object detection >>>"
        # ">>> Ultrasonic Sensors Detect >>>"
        n154 = call "Elasped Timer.vi"("Time Setting"=4.0, "Action"=Elapsed_timer_control."Initialize") -> ()  [unwired: 6 in, 4 out]
        n155 = Bundle By Name(cluster=w2684, "Time up flag"=FALSE) -> (w2682:T15)
      }
      frame "SET TIMER 5" {
        # ">>State Logic  >>"
        # ">>> Time cluster >>>"
        # ">>> Yaw >>>"
        # ">>> Stepper position >>>"
        # ">>> Encoders >>>"
        # ">>> Object detection >>>"
        # ">>> Ultrasonic Sensors Detect >>>"
        n156 = call "Elasped Timer.vi"("Time Setting"=5.0, "Action"=Elapsed_timer_control."Initialize") -> ()  [unwired: 6 in, 4 out]
        n157 = Bundle By Name(cluster=w2697, "Time up flag"=FALSE) -> (w2695:T15)
      }
      frame "START TIMER" {
        # ">>State Logic  >>"
        # ">>> Time cluster >>>"
        # ">>> Yaw >>>"
        # ">>> Stepper position >>>"
        # ">>> Encoders >>>"
        # ">>> Object detection >>>"
        # ">>> Ultrasonic Sensors Detect >>>"
        n158 = call "Elasped Timer.vi"("Action"=Elapsed_timer_control."Start") -> ("Time Out?!"=w2706:bool)  [unwired: 7 in, 3 out]
        n159 = Bundle By Name(cluster=w2709, "Time up flag"=w2706) -> (w2708:T15)
      }
    }
    "State Logic" <- w230
    n160 = local read "TASK ENABLE"() -> (w224:bool)
    n161 = Not(x=w224) -> (.not. x?=w223:bool)
    n162 = case shown="True" w231 {
      tunnel: w235 -> [w261 w299]
      tunnel: w239 -> [w257 w301]
      tunnel: [w261 w299] -> w244
      tunnel: [w257 w302] -> w243
      tunnel: w240 -> [_ w297]
      tunnel: w242 -> [_ w298]
      tunnel: w237 -> [w260 w304]
      tunnel: [w260 w304] -> w236
      tunnel: "STOP TASK" -> [_ w287]
      tunnel: w230 -> [w259 w303]
      tunnel: [w259 w300] -> w229
      tunnel: w226 -> [w258 w293]
      tunnel: [w258 w293] -> w225
      tunnel: w223 -> [_ w288]
      tunnel: [w256 w285] -> w222
      tunnel: w221 -> [w256 w284]
      tunnel: w219 -> [w255 w281]
      tunnel: [w255 w281] -> w218
      tunnel: w216 -> [w254 w277]
      tunnel: [w254 w277] -> w215
      tunnel: w213 -> [w253 w275]
      tunnel: [w253 w275] -> w212
      tunnel: w210 -> [w252 w273]
      tunnel: [w252 w273] -> w209
      tunnel: w208 -> [w251 w272]
      tunnel: [w251 w271] -> w207
      tunnel: [_ w269] -> w206
      tunnel: w204 -> [w250 w267]
      tunnel: [w250 w267] -> w203
      tunnel: w202 -> [w249 w266]
      tunnel: [w249 w265] -> w201
      tunnel: w199 -> [w248 w262]
      tunnel: [w248 w262] -> w198
      frame False {
        # ">>> Line Sensor Cluster>>>"
        # ">>> Line Sensor Cluster>>>"
        # ">>> Motor control cluster >>>"
        # ">>> yStepper command>>>"
        # ">>> Motor control cluster >>>"
        # ">>> yStepper command>>>"
        # ">>> Motor control cluster >>>"
        # ">>> IR Sensors >>>"
        # ">>> IR Sensors >>>"
        # ">>> yStepper command>>>"
        # ">>> Time cluster >>>"
        # ">>> Yaw >>>"
        # ">>> Stepper position >>>"
        # ">>> Encoders >>>"
        # ">>> Object detection >>>"
        # ">>> Ultrasonic Sensors Detect >>>"
        # ">>> Time cluster >>>"
        # ">>> Yaw >>>"
        # ">>> Stepper position >>>"
        # ">>> Encoders >>>"
        # ">>> Object detection >>>"
        # ">>> Ultrasonic Sensors Detect >>>"
      }
      frame True {
        # ">>> IR Sensors >>>"
        # ">>> Line Sensor Cluster>>>"
        # ">>> Line Sensor Cluster>>>"
        # ">>> Motor control cluster >>>"
        # ">>> yStepper command>>>"
        # ">>> IR Sensors >>>"
        # ">>> Motor control cluster >>>"
        # ">>State Logic Queue Reference >>"
        # ">>Timeout>>"
        # ">>> yStepper command>>>"
        # ">>> Time cluster >>>"
        # ">>> Object detection >>>"
        # ">>> Yaw >>>"
        # ">>> Ultrasonic Sensors Detect >>>"
        # ">>> Encoders >>>"
        # ">>> Stepper position >>>"
        # ">>State Logic  >>"
        # ">>True Stop Next State >>"
        # ">>Action Queue>>"
        # ">> Manual override >>"
        # ">>> Time cluster >>>"
        # ">>> Yaw >>>"
        # ">>> Stepper position >>>"
        # ">>> Encoders >>>"
        # ">>> Object detection >>>"
        # ">>> Ultrasonic Sensors Detect >>>"
        # ">>Action Queue>>"
        # ">>State Logic Queue Reference >>"
        n163 = Or(x=w287, y=w288) -> (x .or. y?=w286:bool)
        n164 = Unbundle By Name(w267) -> ("Left IR Sensor"=w268:dbl, "Arm IR Sensor"=w264:dbl)
        "Left IR Sensor" <- w268
        "Arm IR Sensor" <- w264
        n165 = Unbundle By Name(w273) -> ("Time up flag"=w274:bool)
        "Time up flag" <- w274
        n166 = Unbundle By Name(w275) -> ("Yaw"=w276:dbl, "Compass"=w270:dbl)
        n167 = Unbundle By Name(w277) -> ("y Stepper Position"=w279:u8, "z Stepper Position"=w278:u8)
        n168 = Unbundle By Name(w293) -> ("xDistance"=w290:dbl, "yDistance"=w291:dbl, "wDistance"=w292:dbl)
        n169 = Unbundle By Name(w281) -> ("Recognized Object"=w280:bool, "Object X coordinate"=w283:dbl, "Object Y coordinate"=w282:dbl)
        n170 = Unbundle By Name(w304) -> ("PING_A"=w296:u8, "PING_B"=w295:u8, "PING_C"=w294:u8, "PING_D"=w289:u8)
        n171 = Unbundle By Name(w262) -> ("Line Detected?"=w263:bool)
        n172 = case shown="40" w303 {
          tunnel: [w308 w319 w332 w342 w424 w438 w474 w527 w569 w616 w659 w713 w760 w800 w860 w905 w945 w993 w1035 w1087 w1124 w1175 w1218 w1261 w1290 w1307 w1352 w1392 w1440 w1492 w1530 w1578 w1620 w1672 w1709 w1760 w1795 w1843 w1885 w1930 w1973 w2027] -> w302
          tunnel: w301 -> [w308 w322 w333 w345 w426 w439 w483 w525 w573 w617 w665 w706 w763 w807 w850 w908 w951 w992 w1038 w1077 w1130 w1165 w1213 w1252 w1290 w1297 w1355 w1398 w1439 w1491 w1536 w1577 w1623 w1662 w1715 w1750 w1799 w1850 w1890 w1935 w1977 w2025]
          tunnel: [State_Type_Definitions."Idle" ("Enum") State_Type_Definitions."Idle" ("Enum") w328 w344 State_Type_Definitions."Shutdown" ("Enum") w440 w481 w528 w570 w615 w660 w712 w761 w802 w859 w906 w952 w994 w1037 w1086 w1131 w1174 w1219 w1253 State_Type_Definitions."Idle" ("Enum") w1306 w1353 w1399 w1441 w1493 w1537 w1579 w1622 w1671 w1716 w1759 w1796 w1844 w1886 w1931 w1974 w2028] -> w300
          tunnel: w299 -> [_ _ w331 w348 _ w445 w477 w524 w574 w624 w664 w710 w764 w806 w857 w903 w950 w990 w1039 w1084 w1129 w1172 w1216 w1260 _ w1304 w1350 w1397 w1437 w1489 w1535 w1575 w1624 w1669 w1714 w1757 w1803 w1849 w1893 w1938 w1981 w2024]
          tunnel: w298 -> [_ _ _ w347 _ w444 w476 w523 w575 w623 w663 w709 w757 w805 w856 w902 w949 w989 w1040 w1083 w1128 w1171 w1215 w1258 _ w1303 w1349 w1396 w1436 w1488 w1534 w1574 w1625 w1668 w1713 w1756 w1798 w1848 w1892 w1937 w1976 w2023]
          tunnel: w297 -> [_ _ w330 w343 _ w443 w475 w522 w576 w622 w662 w708 w756 w804 w858 w904 w948 w988 w1041 w1085 w1127 w1173 w1214 w1259 _ w1305 w1351 w1395 w1435 w1487 w1533 w1573 w1626 w1670 w1712 w1758 w1802 w1847 w1891 w1936 w1980 w2022]
          tunnel: w286 -> [_ _ _ _ _ w437 w482 w521 w577 w619 w658 w711 w762 w808 w851 w909 w946 w991 w1042 w1078 w1125 w1166 w1217 w1256 _ w1298 w1356 w1393 w1438 w1490 w1531 w1576 w1627 w1663 w1710 w1751 w1801 w1842 w1889 w1934 w1979 w2021]
          tunnel: w296 -> [_ _ _ _ _ _ _ _ _ _ _ _ _ _ _ _ _ _ _ _ _ _ _ _ _ _ _ _ _ _ _ _ _ _ _ _ _ _ _ _ _ _]
          tunnel: w295 -> [_ _ _ _ _ _ _ w520 _ _ _ w702 w745 w798 _ w895 _ _ _ _ _ _ _ _ _ _ w1342 _ _ _ _ _ _ _ _ _ _ _ _ _ _ _]
          tunnel: w294 -> [_ _ _ _ _ _ _ w519 _ _ _ w703 w746 w799 _ w896 _ _ _ _ _ _ _ _ _ _ w1343 _ _ _ _ _ _ _ _ _ _ _ _ _ _ _]
          tunnel: w292 -> [_ _ _ _ _ _ _ _ _ w621 _ _ _ _ _ _ _ _ _ _ _ _ _ _ _ _ _ _ _ _ _ _ _ _ _ _ _ _ _ _ _ _]
          tunnel: w291 -> [_ _ _ _ _ w436 _ _ w568 _ _ _ _ w803 _ _ _ _ _ _ _ _ _ _ _ _ _ _ _ _ _ _ _ _ _ _ _ _ _ _ _ _]
          tunnel: w290 -> [_ _ _ _ _ _ _ _ _ _ _ _ w751 _ _ _ _ _ _ _ _ _ _ _ _ _ _ _ _ w1478 _ _ _ _ _ _ _ _ _ _ _ _]
          tunnel: w289 -> [_ _ _ _ _ _ _ _ _ _ _ _ _ _ _ _ _ _ _ _ _ _ _ _ _ _ _ _ _ _ _ _ _ _ _ _ _ _ _ _ _ _]
          tunnel: [State_Type_Definitions."Idle" ("Enum") State_Type_Definitions."Idle" ("Enum") State_Type_Definitions."Idle" ("Enum") State_Type_Definitions."Idle" ("Enum") State_Type_Definitions."Shutdown" ("Enum") w433 w480 w526 w571 w612 w657 w705 w759 w801 w861 w907 w944 w995 w1036 w1088 w1123 w1176 w1220 w1254 w1292 w1308 w1354 w1391 w1442 w1494 w1529 w1580 w1621 w1673 w1708 w1761 w1797 w1845 w1888 w1933 w1975 w2026] -> w285
          tunnel: w284 -> [_ _ w328 _ _ _ _ _ _ _ _ _ _ _ _ _ _ _ _ _ _ _ _ _ w1292 _ _ _ _ _ _ _ _ _ _ _ _ _ _ _ _ _]
          tunnel: w280 -> [_ _ _ _ _ _ _ _ _ _ _ _ _ _ _ _ _ _ _ _ _ _ _ w1255 _ _ _ _ _ _ _ _ _ _ _ _ _ _ _ _ _ _]
          tunnel: w283 -> [_ _ _ _ _ _ _ _ _ _ _ _ _ _ _ _ _ _ _ _ _ _ _ _ _ _ _ _ _ w1484 _ _ _ _ _ _ _ _ _ _ _ _]
          tunnel: w282 -> [_ _ _ _ _ _ _ _ _ _ _ _ _ _ _ _ _ _ w1031 _ _ _ _ _ _ _ _ _ _ _ _ _ w1616 _ _ _ _ _ _ _ _ _]
          tunnel: w279 -> [_ _ _ _ _ _ _ _ _ _ _ _ _ _ _ _ _ _ w1030 _ _ _ _ _ _ _ _ _ _ _ _ _ w1615 _ _ _ _ _ _ _ _ _]
          tunnel: w278 -> [_ _ _ _ _ _ w479 _ _ _ w655 _ _ _ w854 _ _ _ _ w1081 _ w1169 w1212 _ _ w1301 _ _ _ _ _ _ _ w1666 _ w1754 w1800 _ _ _ w1978 _]
          tunnel: w276 -> [_ _ _ _ _ _ _ _ _ _ _ _ _ _ _ _ _ _ _ _ _ _ _ _ _ _ _ _ _ _ _ _ _ _ _ _ _ _ _ _ _ _]
          tunnel: w274 -> [_ _ _ _ _ _ _ _ _ _ _ _ _ _ _ _ w942 w985 _ _ w1121 _ _ _ _ _ _ w1389 w1432 _ w1527 w1570 _ _ w1706 _ _ _ _ _ _ _]
          tunnel: w272 -> [w306 w317 w327 w340 w422 w432 w478 w518 w572 w611 w656 w704 w755 w797 w849 w900 w943 w986 w1033 w1076 w1122 w1164 w1209 w1251 w1293 w1296 w1347 w1390 w1433 w1485 w1528 w1571 w1618 w1661 w1707 w1749 w1794 w1846 w1887 w1932 w1972 w2020]
          tunnel: [w306 w316 w327 w340 w422 w432 w478 w518 w572 w611 w656 w704 w755 w797 w849 w900 w943 w986 w1032 w1076 w1122 w1164 w1209 w1251 w1293 w1296 w1347 w1390 w1433 w1485 w1528 w1571 w1617 w1661 w1707 w1749 w1794 w1846 w1887 w1932 w1972 w2020] -> w271
          tunnel: w270 -> [_ _ _ _ _ _ _ _ _ _ _ _ _ _ _ _ _ _ _ _ _ _ _ _ _ _ _ _ _ _ _ _ _ _ _ _ _ w1841 _ _ _ _]
          tunnel: [_ _ _ TRUE _ _ _ _ _ _ _ _ _ _ _ _ _ _ _ _ _ _ _ _ _ _ _ _ _ _ _ _ _ _ _ _ _ _ _ _ _ _] -> w269
          tunnel: w268 -> [_ _ _ _ _ _ _ _ _ _ _ _ _ _ _ _ _ _ _ _ _ _ _ _ _ _ _ _ _ _ _ _ _ _ _ _ _ _ _ _ _ _]
          tunnel: w266 -> [w305 w314 w326 w338 w421 w431 w473 w517 w565 w610 w652 w697 w744 w796 w848 w893 w941 w984 w1027 w1075 w1120 w1163 w1208 w1250 w1294 w1295 w1340 w1388 w1431 w1481 w1526 w1569 w1612 w1660 w1705 w1748 w1793 w1837 w1884 w1929 w1971 w2019]
          tunnel: [w305 w313 w326 w338 w421 w431 w473 w517 w565 w610 w652 w697 w744 w796 w848 w893 w941 w984 w1027 w1075 w1120 w1163 w1208 w1250 w1294 w1295 w1340 w1388 w1431 w1480 w1526 w1569 w1612 w1660 w1705 w1748 w1793 w1837 w1884 w1929 w1971 w2019] -> w265
          tunnel: w264 -> [_ _ _ _ _ _ _ _ _ _ _ _ _ _ _ _ _ _ _ _ _ _ _ _ _ _ _ _ _ _ _ _ _ _ _ _ _ _ _ w1927 _ w2018]
          tunnel: w263 -> [_ _ _ _ _ _ _ _ _ _ _ _ _ _ _ _ _ _ _ _ _ _ _ _ _ _ _ _ _ _ _ _ _ _ _ _ _ _ w1883 _ _ _]
          frame 0 {
            # ">>> yStepper command>>>"
          }
          frame 1 {
            # ">>> yStepper command>>>"
            n173 = for {
              shift-right: [w325] -> w319
              shift-left: w322 -> [w324]
              tunnel: string[] ["INIT", "RESET ARM", "RESET FLAGS", "RESET YAW", "NAVX CALIBRATE"] -> [w323] mode=indexing
              n174 = Enqueue Element(queue=w324, element=w323) -> (queue out=w325:refnum<queue>)  [unwired: 2 in, 2 out]
            }
            n175 = Bundle By Name(cluster=w317, "yStepper desired"=u8 0) -> (w316:T14)
            n176 = Bundle By Name(cluster=w314, "ySpeed"=0.0, "xSpeed"=0.0, "wSpeed"=0.0) -> (w313:T12)
          }
          frame 3 {
            # ">>> Motor control cluster >>>"
            # ">>> yStepper command>>>"
            n177 = Flush Queue(queue=w331, error in (no error)=w330) -> ()  [unwired: 3 out]
            n178 = for {
              shift-right: [w337] -> w332
              shift-left: w333 -> [w336]
              tunnel: string[] ["STOP", "RESET ENCODERS", "RESET YAW", "RESET ARM", "RESET FLAGS", "DISPOSE BUFFERS", "CAM CLOSE", ""] -> [w335] mode=indexing
              n179 = Enqueue Element(queue=w336, element=w335) -> (queue out=w337:refnum<queue>)  [unwired: 2 in, 2 out]
            }
          }
          frame 4, Default {
            (unwired) TRUE ("Green LED")
            # ">>> yStepper command>>>"
            n180 = Dequeue Element(queue=w348, timeout in ms (-1)=w347, error in (no error)=w343) -> (element=w346:T10)  [unwired: 3 out]
            n181 = case shown="\"Start Task A\"" w346 {
              tunnel: [w350 w357 w364 w371 w378 w385 w392 w394 w402 w409 w415] -> w342
              tunnel: w345 -> [w351 w358 w365 w372 w379 w386 w392 w395 w401 w408 w416]
              tunnel: [State_Type_Definitions."Task 1" ("Enum") State_Type_Definitions."Task 2:Raise Arm" ("Enum") State_Type_Definitions."Task 3" ("Enum") State_Type_Definitions."Task 4_A" ("Enum") State_Type_Definitions."Task 5A: ARM CAM HEIGHT" ("Enum") State_Type_Definitions."Task 6_A" ("Enum") State_Type_Definitions."Idle" ("Enum") State_Type_Definitions."Shutdown" ("Enum") State_Type_Definitions."Task 9A: Raise Arm" ("Enum") State_Type_Definitions."Task A: RAISE ARM TO HEIGHT" ("Enum") State_Type_Definitions."Task 8A: RAISE ARM" ("Enum")] -> w344
              frame "Start Task 1" {
                n182 = for {
                  shift-right: [w355] -> w350
                  shift-left: w351 -> [w354]
                  tunnel: string[] ["RESET ENCODERS", "RESET YAW", "FORWARD", "READ ENCODERS"] -> [w353] mode=indexing
                  n183 = Enqueue Element(queue=w354, element=w353) -> (queue out=w355:refnum<queue>)  [unwired: 2 in, 2 out]
                }
              }
              frame "Start Task 2" {
                n184 = for {
                  shift-right: [w362] -> w357
                  shift-left: w358 -> [w361]
                  tunnel: string[] ["RESET ENCODERS", "RESET YAW", "READ ULTRASONIC", "ARDUINO - ULTRASONIC"] -> [w360] mode=indexing
                  n185 = Enqueue Element(queue=w361, element=w360) -> (queue out=w362:refnum<queue>)  [unwired: 2 in, 2 out]
                }
              }
              frame "Start Task 3" {
                n186 = for {
                  shift-right: [w369] -> w364
                  shift-left: w365 -> [w368]
                  tunnel: string[] ["RESET ENCODERS", "READ ENCODERS", "R-ACW"] -> [w367] mode=indexing
                  n187 = Enqueue Element(queue=w368, element=w367) -> (queue out=w369:refnum<queue>)  [unwired: 2 in, 2 out]
                }
              }
              frame "Start Task 4" {
                n188 = for {
                  shift-right: [w376] -> w371
                  shift-left: w372 -> [w375]
                  tunnel: string[] ["RESET YAW", "RESET ENCODERS", "RESET ARM", "RESET FLAGS", "", ""] -> [w374] mode=indexing
                  n189 = Enqueue Element(queue=w375, element=w374) -> (queue out=w376:refnum<queue>)  [unwired: 2 in, 2 out]
                }
              }
              frame "Start Task 5" {
                n190 = for {
                  shift-right: [w383] -> w378
                  shift-left: w379 -> [w382]
                  tunnel: string[] ["RESET YAW", "RESET ENCODERS", "READ STEPPER VALUES", "Z STEPPER CAM HEIGHT", "", ""] -> [w381] mode=indexing
                  n191 = Enqueue Element(queue=w382, element=w381) -> (queue out=w383:refnum<queue>)  [unwired: 2 in, 2 out]
                }
              }
              frame "Start Task 6" {
                n192 = for {
                  shift-right: [w390] -> w385
                  shift-left: w386 -> [w389]
                  tunnel: string[] ["OPEN LOG CAM ", "", "", "", "", ""] -> [w388] mode=indexing
                  n193 = Enqueue Element(queue=w389, element=w388) -> (queue out=w390:refnum<queue>)  [unwired: 2 in, 2 out]
                }
              }
              frame "None", Default {
              }
              frame "Exit" {
                n194 = for {
                  shift-right: [w399] -> w394
                  shift-left: w395 -> [w398]
                  tunnel: string[] ["STOP", "RESET ENCODERS", "RESET YAW", "EXIT"] -> [w397] mode=indexing
                  n195 = Enqueue Element(queue=w398, element=w397) -> (queue out=w399:refnum<queue>)  [unwired: 2 in, 2 out]
                }
              }
              frame "Start Task 9" {
                n196 = for {
                  shift-right: [w406] -> w402
                  shift-left: w401 -> [w405]
                  tunnel: string[] ["RESET ENCODERS", "READ ENCODERS", "Z STEPPER CAM HEIGHT"] -> [w404] mode=indexing
                  n197 = Enqueue Element(queue=w405, element=w404) -> (queue out=w406:refnum<queue>)  [unwired: 2 in, 2 out]
                }
              }
              frame "Start Task A" {
                n198 = for {
                  shift-right: [w413] -> w409
                  shift-left: w408 -> [w412]
                  tunnel: string[] ["RESET ENCODERS", "READ ENCODERS", "RESET YAW", "Z STEPPER BOX HEIGHT"] -> [w411] mode=indexing
                  n199 = Enqueue Element(queue=w412, element=w411) -> (queue out=w413:refnum<queue>)  [unwired: 2 in, 2 out]
                }
              }
              frame "Start Task 8 - BALL" {
                n200 = for {
                  shift-right: [w420] -> w415
                  shift-left: w416 -> [w419]
                  tunnel: string[] ["RESET YAW", "RESET ENCODERS", "RESET ARM", "RESET FLAGS"] -> [w418] mode=indexing
                  n201 = Enqueue Element(queue=w419, element=w418) -> (queue out=w420:refnum<queue>)  [unwired: 2 in, 2 out]
                }
              }
            }
          }
          frame 5 {
            # ">>> yStepper command>>>"
            n202 = for {
              shift-right: [w430] -> w424
              shift-left: w426 -> [w429]
              tunnel: string[] ["INIT", "RESET ENCODERS", "RESET FLAGS", "CAM CLOSE", "DISPOSE BUFFERS", "EXIT", ""] -> [w428] mode=indexing
              n203 = Enqueue Element(queue=w429, element=w428) -> (queue out=w430:refnum<queue>)  [unwired: 2 in, 2 out]
            }
          }
          frame 6 {
            # ">>> yStepper command>>>"
            # "Use 250"
            n204 = Dequeue Element(queue=w445, timeout in ms (-1)=w444, error in (no error)=w443) -> (element=w442:T10)  [unwired: 3 out]
            n205 = Greater?(x=w436, y=265.0) -> (0:w434:bool)
            n206 = Or(x=w434, y=w437) -> (x .or. y?=w441:bool)
            n207 = case shown="\"None\", Default" w442 {
              tunnel: w441 -> [w448 _]
              tunnel: [w452 State_Type_Definitions."True Stop" ("Enum")] -> w440
              tunnel: w439 -> [w449 w467]
              tunnel: [w447 w466] -> w438
              tunnel: [State_Type_Definitions."Idle" ("Enum") State_Type_Definitions."Shutdown" ("Enum")] -> w433
              frame "None", Default {
                n208 = case shown="True" w448 {
                  tunnel: w449 -> [w455 w461]
                  tunnel: [w454 w459] -> w447
                  frame False {
                    n209 = for {
                      shift-right: [w457] -> w454
                      shift-left: w455 -> [w458]
                      tunnel: string[] ["READ ENCODERS", "READ NAVX", "FORWARD"] ("element") -> [w456] mode=indexing
                      n210 = Enqueue Element(queue=w458, element=w456) -> (queue out=w457:refnum<queue>)  [unwired: 2 in, 2 out]
                    }
                  }
                  frame True {
                    n211 = for {
                      shift-right: [w463] -> w459
                      shift-left: w461 -> [w464]
                      tunnel: string[] ["RESET YAW", "RESET ENCODERS", "STOP", ""] -> [w462] mode=indexing
                      n212 = Enqueue Element(queue=w464, element=w462) -> (queue out=w463:refnum<queue>)  [unwired: 2 in, 2 out]
                    }
                  }
                }
                n213 = Select(t=State_Type_Definitions."True Stop" ("Enum"), s=w448, f=State_Type_Definitions."Task 1" ("Enum")) -> (s? t:f=w452:u16)
              }
              frame "Exit" {
                n214 = for {
                  shift-right: [w471] -> w466
                  shift-left: w467 -> [w472]
                  tunnel: string[] ["STOP", "RESET ENCODERS", "RESET YAW", ""] -> [w470] mode=indexing
                  n215 = Enqueue Element(queue=w472, element=w470) -> (queue out=w471:refnum<queue>)  [unwired: 2 in, 2 out]
                }
              }
            }
          }
          frame 8 {
            # ">> Stepper height reeached >>"
            # ">>> yStepper command>>>"
            # ">> Manual override >>"
            n216 = Dequeue Element(queue=w477, timeout in ms (-1)=w476, error in (no error)=w475) -> (element=w486:T10)  [unwired: 3 out]
            n217 = Equal?(x=w479, y=u8 60) -> (x = y?=w484:bool)
            n218 = case shown="\"None\", Default" w486 {
              tunnel: [w497 State_Type_Definitions."True Stop" ("Enum")] -> w481
              tunnel: [w495 w512] -> w474
              tunnel: w483 -> [w494 _]
              tunnel: w482 -> [w488 _]
              tunnel: [State_Type_Definitions."Idle" ("Enum") State_Type_Definitions."Shutdown" ("Enum")] -> w480
              tunnel: w484 -> [w487 _]
              frame "None", Default {
                # ">> WIill proceed to part ii if not manual override >>"
                # ">>If ENABLE or Trigger is set to true>>"
                n219 = Or(x=w487, y=w488) -> (x .or. y?=w489:bool)
                n220 = case shown="True" w487 {
                  tunnel: [w500 w506] -> w495
                  tunnel: w494 -> [w499 w505]
                  frame False {
                    n221 = for {
                      shift-right: [w502] -> w500
                      shift-left: w499 -> [w503]
                      tunnel: string[] ["Z STEPPER CAM HEIGHT", "READ STEPPER VALUES"] ("element") -> [w501] mode=indexing
                      n222 = Enqueue Element(queue=w503, element=w501) -> (queue out=w502:refnum<queue>)  [unwired: 2 in, 2 out]
                    }
                  }
                  frame True {
                    n223 = for {
                      shift-right: [w508] -> w506
                      shift-left: w505 -> [w509]
                      tunnel: string[] ["ARDUINO - ULTRASONIC", "READ ULTRASONIC", "", "", "", ""] -> [w507] mode=indexing
                      n224 = Enqueue Element(queue=w509, element=w507) -> (queue out=w508:refnum<queue>)  [unwired: 2 in, 2 out]
                    }
                  }
                }
                n225 = Select(t=State_Type_Definitions."True Stop" ("Enum"), s=w488, f=State_Type_Definitions."Task 2:Sensor Mode" ("Enum")) -> (s? t:f=w491:T9)
                n226 = Select(t=w491, s=w489, f=State_Type_Definitions."Task 2:Raise Arm" ("Enum")) -> (s? t:f=w497:T9)
              }
              frame "Exit" {
                n227 = for {
                  shift-right: [w515] -> w512
                  shift-left: _ -> [w516]
                  tunnel: string[] ["STOP", "RESET ENCODERS", "RESET YAW", ""] -> [w514] mode=indexing
                  n228 = Enqueue Element(queue=w516, element=w514) -> (queue out=w515:refnum<queue>)  [unwired: 2 in, 2 out]
                }
              }
            }
          }
          frame 9 {
            w532 = u8 20 ("y")
            # ">>> yStepper command>>>"
            # ">>Object detected>>"
            n229 = Dequeue Element(queue=w524, timeout in ms (-1)=w523, error in (no error)=w522) -> (element=w533:T10)  [unwired: 3 out]
            n230 = Less?(x=w520, y=w532) -> (x < y?=w531:bool)
            n231 = Less?(x=w519, y=w532) -> (x < y?=w530:bool)
            n232 = Or(x=w531, y=w530) -> (x .or. y?=w529:bool)
            "Obstacle detected" <- w529
            n233 = case shown="\"None\", Default" w533 {
              tunnel: w529 -> [w536 _]
              tunnel: [w543 State_Type_Definitions."True Stop" ("Enum")] -> w528
              tunnel: w521 -> [w535 _]
              tunnel: w525 -> [w542 w559]
              tunnel: [w541 w560] -> w527
              tunnel: [State_Type_Definitions."Idle" ("Enum") State_Type_Definitions."Shutdown" ("Enum")] -> w526
              frame "None", Default {
                n234 = case shown="True" w536 {
                  tunnel: w542 -> [w546 w553]
                  tunnel: [w547 w552] -> w541
                  frame False {
                    n235 = for {
                      tunnel: string[] ["READ ULTRASONIC", "STOP"] ("element") -> [w548] mode=indexing
                      shift-right: [w550] -> w547
                      shift-left: w546 -> [w549]
                      n236 = Enqueue Element(queue=w549, element=w548) -> (queue out=w550:refnum<queue>)  [unwired: 2 in, 2 out]
                    }
                  }
                  frame True {
                    n237 = for {
                      shift-right: [w555] -> w552
                      shift-left: w553 -> [w556]
                      tunnel: string[] ["RESET ENCODERS", "READ NAVX", "READ ENCODERS"] -> [w554] mode=indexing
                      n238 = Enqueue Element(queue=w556, element=w554) -> (queue out=w555:refnum<queue>)  [unwired: 2 in, 2 out]
                    }
                  }
                }
                n239 = Or(x=w536, y=w535) -> (x .or. y?=w534:bool)
                n240 = Select(t=State_Type_Definitions."True Stop" ("Enum"), s=w535, f=State_Type_Definitions."Task 2:Reverse Mode" ("Enum")) -> (s? t:f=w537:T9)
                n241 = Select(t=w537, s=w534, f=State_Type_Definitions."Task 2:Sensor Mode" ("Enum")) -> (s? t:f=w543:T9)
              }
              frame "Exit" {
                n242 = for {
                  shift-right: [w563] -> w560
                  shift-left: w559 -> [w564]
                  tunnel: string[] ["STOP", "RESET ENCODERS", "RESET YAW", "ARDUINO MODE 0"] -> [w562] mode=indexing
                  n243 = Enqueue Element(queue=w564, element=w562) -> (queue out=w563:refnum<queue>)  [unwired: 2 in, 2 out]
                }
              }
            }
          }
          frame 10 {
            # ">>> yStepper command>>>"
            n244 = Dequeue Element(queue=w574, timeout in ms (-1)=w575, error in (no error)=w576) -> (element=w578:T10)  [unwired: 3 out]
            n245 = Less?(x=w568, y=-50.0) -> (x < y?=w566:bool)
            n246 = case shown="\"None\", Default" w578 {
              tunnel: [w588 State_Type_Definitions."True Stop" ("Enum")] -> w570
              tunnel: w577 -> [w581 _]
              tunnel: w573 -> [w587 w604]
              tunnel: [w586 w605] -> w569
              tunnel: [State_Type_Definitions."Idle" ("Enum") State_Type_Definitions."Shutdown" ("Enum")] -> w571
              tunnel: w566 -> [w579 _]
              frame "None", Default {
                n247 = case shown="False" w579 {
                  tunnel: w587 -> [w591 w598]
                  tunnel: [w592 w597] -> w586
                  frame False {
                    n248 = for {
                      tunnel: string[] ["READ ENCODERS", "REVERSE", "READ NAVX"] ("element") -> [w593] mode=indexing
                      shift-right: [w595] -> w592
                      shift-left: w591 -> [w594]
                      n249 = Enqueue Element(queue=w594, element=w593) -> (queue out=w595:refnum<queue>)  [unwired: 2 in, 2 out]
                    }
                  }
                  frame True {
                    n250 = for {
                      shift-right: [w600] -> w597
                      shift-left: w598 -> [w601]
                      tunnel: string[] ["STOP", "ARDUINO - ULTRASONIC", "READ ULTRASONIC", "RESET ENCODERS"] -> [w599] mode=indexing
                      n251 = Enqueue Element(queue=w601, element=w599) -> (queue out=w600:refnum<queue>)  [unwired: 2 in, 2 out]
                    }
                  }
                }
                n252 = Or(x=w579, y=w581) -> (x .or. y?=w580:bool)
                n253 = Select(t=State_Type_Definitions."True Stop" ("Enum"), s=w581, f=State_Type_Definitions."Task 2:Sensor Mode" ("Enum")) -> (s? t:f=w582:T9)
                n254 = Select(t=w582, s=w580, f=State_Type_Definitions."Task 2:Reverse Mode" ("Enum")) -> (s? t:f=w588:T9)
              }
              frame "Exit" {
                n255 = for {
                  shift-right: [w608] -> w605
                  shift-left: w604 -> [w609]
                  tunnel: string[] ["STOP", "RESET ENCODERS", "RESET YAW", "ARDUINO MODE 0"] -> [w607] mode=indexing
                  n256 = Enqueue Element(queue=w609, element=w607) -> (queue out=w608:refnum<queue>)  [unwired: 2 in, 2 out]
                }
              }
            }
          }
          frame 11 {
            # ">>> yStepper command>>>"
            n257 = Dequeue Element(queue=w624, timeout in ms (-1)=w623, error in (no error)=w622) -> (element=w613:T10)  [unwired: 3 out]
            n258 = Greater?(x=w621, y=160.0) -> (0:w618:bool)
            n259 = Or(x=w618, y=w619) -> (x .or. y?=w614:bool)
            n260 = case shown="\"None\", Default" w613 {
              tunnel: w614 -> [w627 _]
              tunnel: [w631 State_Type_Definitions."True Stop" ("Enum")] -> w615
              tunnel: w617 -> [w628 w647]
              tunnel: [w626 w646] -> w616
              tunnel: [State_Type_Definitions."Idle" ("Enum") State_Type_Definitions."Shutdown" ("Enum")] -> w612
              frame "None", Default {
                n261 = case shown="False" w627 {
                  tunnel: w628 -> [w634 w640]
                  tunnel: [w633 w638] -> w626
                  frame False {
                    n262 = for {
                      shift-right: [w636] -> w633
                      shift-left: w634 -> [w637]
                      tunnel: string[] ["READ ENCODERS", "R-CW"] ("element") -> [w635] mode=indexing
                      n263 = Enqueue Element(queue=w637, element=w635) -> (queue out=w636:refnum<queue>)  [unwired: 2 in, 2 out]
                    }
                  }
                  frame True {
                    n264 = for {
                      shift-right: [w642] -> w638
                      shift-left: w640 -> [w643]
                      tunnel: string[] ["RESET YAW", "RESET ENCODERS", "STOP", "ARDUINO MODE 0"] -> [w641] mode=indexing
                      n265 = Enqueue Element(queue=w643, element=w641) -> (queue out=w642:refnum<queue>)  [unwired: 2 in, 2 out]
                    }
                  }
                }
                n266 = Select(t=State_Type_Definitions."True Stop" ("Enum"), s=w627, f=State_Type_Definitions."Task 3" ("Enum")) -> (s? t:f=w631:T9)
              }
              frame "Exit" {
                n267 = for {
                  shift-right: [w650] -> w646
                  shift-left: w647 -> [w651]
                  tunnel: string[] ["STOP", "RESET ENCODERS", "RESET YAW", ""] -> [w649] mode=indexing
                  n268 = Enqueue Element(queue=w651, element=w649) -> (queue out=w650:refnum<queue>)  [unwired: 2 in, 2 out]
                }
              }
            }
          }
          frame 12 {
            # ">> Stepper height reeached >>"
            # ">>> yStepper command>>>"
            # ">> Manual override >>"
            n269 = Dequeue Element(queue=w664, timeout in ms (-1)=w663, error in (no error)=w662) -> (element=w661:T10)  [unwired: 3 out]
            n270 = Equal?(x=w655, y=u8 60) -> (x = y?=w653:bool)
            n271 = case shown="\"Exit\"" w661 {
              tunnel: [w676 State_Type_Definitions."True Stop" ("Enum")] -> w660
              tunnel: [w674 w692] -> w659
              tunnel: w665 -> [w673 w689]
              tunnel: w658 -> [w667 _]
              tunnel: [State_Type_Definitions."Idle" ("Enum") State_Type_Definitions."Shutdown" ("Enum")] -> w657
              tunnel: w653 -> [w666 _]
              frame "None", Default {
                # ">> WIill proceed to part ii if not manual override >>"
                # ">>If ENABLE or Trigger is set to true>>"
                n272 = Or(x=w666, y=w667) -> (x .or. y?=w668:bool)
                n273 = case shown="False" w666 {
                  tunnel: [w679 w685] -> w674
                  tunnel: w673 -> [w678 w684]
                  frame False {
                    n274 = for {
                      shift-right: [w681] -> w679
                      shift-left: w678 -> [w682]
                      tunnel: string[] ["Z STEPPER CAM HEIGHT", "READ STEPPER VALUES"] ("element") -> [w680] mode=indexing
                      n275 = Enqueue Element(queue=w682, element=w680) -> (queue out=w681:refnum<queue>)  [unwired: 2 in, 2 out]
                    }
                  }
                  frame True {
                    n276 = for {
                      shift-right: [w687] -> w685
                      shift-left: w684 -> [w688]
                      tunnel: string[] ["ARDUINO - ULTRASONIC", "READ ULTRASONIC", "FORWARD", "", "", ""] -> [w686] mode=indexing
                      n277 = Enqueue Element(queue=w688, element=w686) -> (queue out=w687:refnum<queue>)  [unwired: 2 in, 2 out]
                    }
                  }
                }
                n278 = Select(t=State_Type_Definitions."True Stop" ("Enum"), s=w667, f=State_Type_Definitions."Task 4_B" ("Enum")) -> (s? t:f=w670:T9)
                n279 = Select(t=w670, s=w668, f=State_Type_Definitions."Task 4_A" ("Enum")) -> (s? t:f=w676:T9)
              }
              frame "Exit" {
                n280 = for {
                  shift-right: [w695] -> w692
                  shift-left: w689 -> [w696]
                  tunnel: string[] ["STOP", "RESET ENCODERS", "RESET YAW", ""] -> [w694] mode=indexing
                  n281 = Enqueue Element(queue=w696, element=w694) -> (queue out=w695:refnum<queue>)  [unwired: 2 in, 2 out]
                }
              }
            }
          }
          frame 13 {
            w701 = u8 20
            # ">> Path blocked >>"
            # ">>> yStepper command>>>"
            # ">> Manual override >>"
            n282 = Dequeue Element(queue=w710, timeout in ms (-1)=w709, error in (no error)=w708) -> (element=w707:T10)  [unwired: 3 out]
            n283 = Less?(x=w703, y=w701) -> (x < y?=w698:bool)
            n284 = Less?(x=w702, y=w701) -> (x < y?=w699:bool)
            n285 = And(x=w699, y=w698) -> (x .and. y?=w700:bool)
            n286 = case shown="\"None\", Default" w707 {
              tunnel: [w724 State_Type_Definitions."True Stop" ("Enum")] -> w712
              tunnel: [w722 w739] -> w713
              tunnel: w706 -> [w721 _]
              tunnel: w711 -> [w715 _]
              tunnel: [State_Type_Definitions."Idle" ("Enum") State_Type_Definitions."Shutdown" ("Enum")] -> w705
              tunnel: w700 -> [w714 _]
              frame "None", Default {
                # ">> Manual override forces program to true stop >>"
                # ">>If ENABLE or Trigger is set to true>>"
                n287 = Or(x=w714, y=w715) -> (x .or. y?=w720:bool)
                n288 = case shown="True" w714 {
                  tunnel: [w727 w732] -> w722
                  tunnel: w721 -> [w726 w731]
                  frame False {
                    n289 = for {
                      shift-right: [w729] -> w727
                      shift-left: w726 -> [w730]
                      tunnel: string[] ["FORWARD", "READ ULTRASONIC", "READ NAVX"] ("element") -> [w728] mode=indexing
                      n290 = Enqueue Element(queue=w730, element=w728) -> (queue out=w729:refnum<queue>)  [unwired: 2 in, 2 out]
                    }
                  }
                  frame True {
                    n291 = for {
                      shift-right: [w735] -> w732
                      shift-left: w731 -> [w736]
                      tunnel: string[] ["STOP", "RESET YAW", "RESET ENCODERS", "RESET FLAGS"] -> [w734] mode=indexing
                      n292 = Enqueue Element(queue=w736, element=w734) -> (queue out=w735:refnum<queue>)  [unwired: 2 in, 2 out]
                    }
                  }
                }
                n293 = Select(t=State_Type_Definitions."True Stop" ("Enum"), s=w715, f=State_Type_Definitions."Task 4_C" ("Enum")) -> (s? t:f=w717:T9)
                n294 = Select(t=w717, s=w720, f=State_Type_Definitions."Task 4_B" ("Enum")) -> (s? t:f=w724:T9)
              }
              frame "Exit" {
                n295 = for {
                  shift-right: [w742] -> w739
                  shift-left: _ -> [w743]
                  tunnel: string[] ["STOP", "RESET ENCODERS", "RESET YAW", ""] -> [w741] mode=indexing
                  n296 = Enqueue Element(queue=w743, element=w741) -> (queue out=w742:refnum<queue>)  [unwired: 2 in, 2 out]
                }
              }
            }
          }
          frame 14 {
            w754 = u8 20
            # ">> xDistance travelled>>"
            # ">> Path NOT blocked >>"
            # ">>> yStepper command>>>"
            # ">> Manual override >>"
            n297 = Dequeue Element(queue=w764, timeout in ms (-1)=w757, error in (no error)=w756) -> (element=w758:T10)  [unwired: 3 out]
            n298 = Greater?(x=w746, y=w754) -> (0:w752:bool)
            n299 = Greater?(x=w751, y=80.0) -> (0:w749:bool)
            n300 = Greater?(x=w745, y=w754) -> (0:w753:bool)
            n301 = And(x=w753, y=w752) -> (x .and. y?=w748:bool)
            n302 = And(x=w749, y=w748) -> (x .and. y?=w747:bool)
            n303 = case shown="\"Exit\"" w758 {
              tunnel: [w775 State_Type_Definitions."True Stop" ("Enum")] -> w761
              tunnel: [w773 w791] -> w760
              tunnel: w763 -> [w772 w788]
              tunnel: w762 -> [w766 _]
              tunnel: [State_Type_Definitions."Idle" ("t") State_Type_Definitions."Shutdown" ("Enum")] -> w759
              tunnel: w747 -> [w765 _]
              frame "None", Default {
                # ">> Manual override forces program to true stop >>"
                # ">>If ENABLE or Trigger is set to true>>"
                n304 = Or(x=w765, y=w766) -> (x .or. y?=w771:bool)
                n305 = case shown="False" w765 {
                  tunnel: [w778 w783] -> w773
                  tunnel: w772 -> [w776 w782]
                  frame False {
                    n306 = for {
                      shift-right: [w780] -> w778
                      shift-left: w776 -> [w781]
                      tunnel: string[] ["RIGHT", "READ NAVX", "READ ENCODERS", "READ ULTRASONIC"] ("element") -> [w779] mode=indexing
                      n307 = Enqueue Element(queue=w781, element=w779) -> (queue out=w780:refnum<queue>)  [unwired: 2 in, 2 out]
                    }
                  }
                  frame True {
                    n308 = for {
                      shift-right: [w786] -> w783
                      shift-left: w782 -> [w787]
                      tunnel: string[] ["STOP", "RESET YAW", "RESET ENCODERS", "ARDUINO - ULTRASONIC"] -> [w785] mode=indexing
                      n309 = Enqueue Element(queue=w787, element=w785) -> (queue out=w786:refnum<queue>)  [unwired: 2 in, 2 out]
                    }
                  }
                }
                n310 = Select(t=State_Type_Definitions."True Stop" ("Enum"), s=w766, f=State_Type_Definitions."Task 4_D" ("Enum")) -> (s? t:f=w767:T9)
                n311 = Select(t=w767, s=w771, f=State_Type_Definitions."Task 4_C" ("Enum")) -> (s? t:f=w775:T9)
              }
              frame "Exit" {
                n312 = for {
                  shift-right: [w794] -> w791
                  shift-left: w788 -> [w795]
                  tunnel: string[] ["STOP", "RESET ENCODERS", "RESET YAW", ""] -> [w793] mode=indexing
                  n313 = Enqueue Element(queue=w795, element=w793) -> (queue out=w794:refnum<queue>)  [unwired: 2 in, 2 out]
                }
              }
            }
          }
          frame 15 {
            w815 = u8 20
            # ">> yDistance travelled>>"
            # ">> Path blocked >>"
            # ">>> yStepper command>>>"
            # ">> Manual override >>"
            n314 = Dequeue Element(queue=w806, timeout in ms (-1)=w805, error in (no error)=w804) -> (element=w816:T10)  [unwired: 3 out]
            n315 = Less?(x=w799, y=w815) -> (x < y?=w813:bool)
            n316 = Greater?(x=w803, y=200.0) -> (0:w811:bool)
            n317 = Less?(x=w798, y=w815) -> (x < y?=w814:bool)
            n318 = And(x=w814, y=w813) -> (x .and. y?=w810:bool)
            n319 = Or(x=w811, y=w810) -> (x .or. y?=w809:bool)
            n320 = case shown="\"None\", Default" w816 {
              tunnel: [w827 State_Type_Definitions."True Stop" ("Enum")] -> w802
              tunnel: [w825 w843] -> w800
              tunnel: w807 -> [w824 w840]
              tunnel: w808 -> [w818 _]
              tunnel: [State_Type_Definitions."Idle" ("t") State_Type_Definitions."Shutdown" ("Enum")] -> w801
              tunnel: w809 -> [w817 _]
              frame "None", Default {
                # ">> Manual override forces program to true stop >>"
                # ">>If ENABLE or Trigger is set to true>>"
                n321 = Or(x=w817, y=w818) -> (x .or. y?=w823:bool)
                n322 = case shown="True" w817 {
                  tunnel: [w830 w835] -> w825
                  tunnel: w824 -> [w828 w834]
                  frame False {
                    n323 = for {
                      shift-right: [w832] -> w830
                      shift-left: w828 -> [w833]
                      tunnel: string[] ["FORWARD", "READ NAVX", "READ ENCODERS", "READ ULTRASONIC"] ("element") -> [w831] mode=indexing
                      n324 = Enqueue Element(queue=w833, element=w831) -> (queue out=w832:refnum<queue>)  [unwired: 2 in, 2 out]
                    }
                  }
                  frame True {
                    n325 = for {
                      shift-right: [w838] -> w835
                      shift-left: w834 -> [w839]
                      tunnel: string[] ["STOP", "RESET YAW", "RESET ENCODERS", "RESET FLAGS"] -> [w837] mode=indexing
                      n326 = Enqueue Element(queue=w839, element=w837) -> (queue out=w838:refnum<queue>)  [unwired: 2 in, 2 out]
                    }
                  }
                }
                n327 = Select(t=State_Type_Definitions."True Stop" ("Enum"), s=w818, f=State_Type_Definitions."True Stop" ("Enum")) -> (s? t:f=w819:T9)
                n328 = Select(t=w819, s=w823, f=State_Type_Definitions."Task 4_D" ("Enum")) -> (s? t:f=w827:T9)
              }
              frame "Exit" {
                n329 = for {
                  shift-right: [w846] -> w843
                  shift-left: w840 -> [w847]
                  tunnel: string[] ["STOP", "RESET ENCODERS", "RESET YAW", ""] -> [w845] mode=indexing
                  n330 = Enqueue Element(queue=w847, element=w845) -> (queue out=w846:refnum<queue>)  [unwired: 2 in, 2 out]
                }
              }
            }
          }
          frame 15 {
            # ">>> yStepper command>>>"
            # ">> Manual override >>"
            n331 = Dequeue Element(queue=w857, timeout in ms (-1)=w856, error in (no error)=w858) -> (element=w855:T10)  [unwired: 3 out]
            n332 = Equal?(x=w854, y=u8 60) -> (x = y?=w852:bool)
            n333 = case shown="\"None\", Default" w855 {
              tunnel: [w868 State_Type_Definitions."True Stop" ("Enum")] -> w859
              tunnel: [w871 w888] -> w860
              tunnel: [State_Type_Definitions."Idle" ("Enum") State_Type_Definitions."Shutdown" ("Enum")] -> w861
              tunnel: w852 -> [w867 _]
              tunnel: w851 -> [w866 _]
              tunnel: w850 -> [w862 w885]
              frame "None", Default {
                # "Stays in Task 5_A until stepper reaches desired \nheight"
                # "T: Go back to idle, F: Continue with task\""
                # ">> Manual override >>"
                n334 = case shown="True" w867 {
                  tunnel: [w875 w881] -> w871
                  tunnel: w862 -> [w873 w879]
                  frame False {
                    n335 = for {
                      tunnel: string[] ["Z STEPPER CAM HEIGHT", "READ STEPPER VALUES"] ("element") -> [w876] mode=indexing
                      shift-right: [w878] -> w875
                      shift-left: w873 -> [w877]
                      n336 = Enqueue Element(queue=w877, element=w876) -> (queue out=w878:refnum<queue>)  [unwired: 2 in, 2 out]
                    }
                  }
                  frame True {
                    n337 = for {
                      shift-right: [w883] -> w881
                      shift-left: w879 -> [w884]
                      tunnel: string[] ["ARDUINO - ULTRASONIC", "READ ULTRASONIC", ""] -> [w882] mode=indexing
                      n338 = Enqueue Element(queue=w884, element=w882) -> (queue out=w883:refnum<queue>)  [unwired: 2 in, 2 out]
                    }
                  }
                }
                n339 = Or(x=w867, y=w866) -> (x .or. y?=w869:bool)
                n340 = Select(t=State_Type_Definitions."True Stop" ("Enum"), s=w866, f=State_Type_Definitions."Task 5B: MOVE TO BOX" ("Enum")) -> (s? t:f=w863:u16)
                n341 = Select(t=w863, s=w869, f=State_Type_Definitions."Task 5A: ARM CAM HEIGHT" ("Enum")) -> (s? t:f=w868:u16)
              }
              frame "Exit" {
                n342 = for {
                  shift-right: [w891] -> w888
                  shift-left: w885 -> [w892]
                  tunnel: string[] ["STOP", "RESET ENCODERS", "RESET YAW", "ARDUINO MODE 0"] -> [w890] mode=indexing
                  n343 = Enqueue Element(queue=w892, element=w890) -> (queue out=w891:refnum<queue>)  [unwired: 2 in, 2 out]
                }
              }
            }
          }
          frame 16 {
            w899 = u8 20 ("y")
            # ">>> yStepper command>>>"
            n344 = Less?(x=w896, y=w899) -> (x < y?=w897:bool)
            n345 = Dequeue Element(queue=w903, timeout in ms (-1)=w902, error in (no error)=w904) -> (element=w901:T10)  [unwired: 3 out]
            n346 = Less?(x=w895, y=w899) -> (x < y?=w898:bool)
            n347 = And(x=w898, y=w897) -> (x .and. y?=w894:bool)
            n348 = case shown="\"None\", Default" w901 {
              tunnel: [w916 State_Type_Definitions."True Stop" ("Enum")] -> w906
              tunnel: [w919 w936] -> w905
              tunnel: [State_Type_Definitions."Idle" ("Enum") State_Type_Definitions."Shutdown" ("Enum")] -> w907
              tunnel: w909 -> [w915 _]
              tunnel: w908 -> [w911 w933]
              tunnel: w894 -> [w910 _]
              frame "None", Default {
                # "Stays in Task 5_B to capture image over 5 seconds"
                # "T: Go back to idle, F: Continue with task\""
                # ">> Manual override >>"
                n349 = case shown="True" w910 {
                  tunnel: [w923 w929] -> w919
                  tunnel: w911 -> [w921 w927]
                  frame False {
                    n350 = for {
                      tunnel: string[] ["FORWARD", "READ ULTRASONIC", "READ NAVX"] ("element") -> [w924] mode=indexing
                      shift-right: [w926] -> w923
                      shift-left: w921 -> [w925]
                      n351 = Enqueue Element(queue=w925, element=w924) -> (queue out=w926:refnum<queue>)  [unwired: 2 in, 2 out]
                    }
                  }
                  frame True {
                    n352 = for {
                      shift-right: [w931] -> w929
                      shift-left: w927 -> [w932]
                      tunnel: string[] ["STOP", "RESET ENCODERS", "OPEN LOG CAM", "SET TIMER 5"] -> [w930] mode=indexing
                      n353 = Enqueue Element(queue=w932, element=w930) -> (queue out=w931:refnum<queue>)  [unwired: 2 in, 2 out]
                    }
                  }
                }
                n354 = Or(x=w910, y=w915) -> (x .or. y?=w917:bool)
                n355 = Select(t=State_Type_Definitions."True Stop" ("Enum"), s=w915, f=State_Type_Definitions."Task 5C: CAM BURST" ("Enum")) -> (s? t:f=w912:u16)
                n356 = Select(t=w912, s=w917, f=State_Type_Definitions."Task 5B: MOVE TO BOX" ("Enum")) -> (s? t:f=w916:u16)
              }
              frame "Exit" {
                n357 = for {
                  shift-right: [w939] -> w936
                  shift-left: w933 -> [w940]
                  tunnel: string[] ["STOP", "RESET ENCODERS", "RESET YAW", "ARDUINO MODE 0"] -> [w938] mode=indexing
                  n358 = Enqueue Element(queue=w940, element=w938) -> (queue out=w939:refnum<queue>)  [unwired: 2 in, 2 out]
                }
              }
            }
          }
          frame 17 {
            # ">>> Motor control cluster >>>"
            # ">>> yStepper command>>>"
            # ">> Manual override >>"
            n359 = Dequeue Element(queue=w950, timeout in ms (-1)=w949, error in (no error)=w948) -> (element=w947:T10)  [unwired: 3 out]
            n360 = case shown="\"None\", Default" w947 {
              tunnel: [w959 State_Type_Definitions."True Stop" ("Enum")] -> w952
              tunnel: [w962 w979] -> w945
              tunnel: [State_Type_Definitions."Idle" ("Enum") State_Type_Definitions."Shutdown" ("Enum")] -> w944
              tunnel: w946 -> [w953 _]
              tunnel: w951 -> [w958 w976]
              tunnel: w942 -> [w957 _]
              frame "None", Default {
                # ">> Is time up? >>"
                # "Determines if object is in range to pick up"
                # ">> Manual override >>"
                n361 = case shown="False" w957 {
                  tunnel: [w966 w972] -> w962
                  tunnel: w958 -> [w964 w970]
                  frame False {
                    n362 = for {
                      tunnel: string[] ["CAM ACQ", "START TIMER"] ("element") -> [w967] mode=indexing
                      shift-right: [w969] -> w966
                      shift-left: w964 -> [w968]
                      n363 = Enqueue Element(queue=w968, element=w967) -> (queue out=w969:refnum<queue>)  [unwired: 2 in, 2 out]
                    }
                  }
                  frame True {
                    n364 = for {
                      shift-right: [w974] -> w972
                      shift-left: w970 -> [w975]
                      tunnel: string[] ["CAM CLOSE", "PROCESS IMAGE", "SET TIMER 5"] -> [w973] mode=indexing
                      n365 = Enqueue Element(queue=w975, element=w973) -> (queue out=w974:refnum<queue>)  [unwired: 2 in, 2 out]
                    }
                  }
                }
                n366 = Or(x=w957, y=w953) -> (x .or. y?=w960:bool)
                n367 = Select(t=State_Type_Definitions."True Stop" ("Enum"), s=w953, f=State_Type_Definitions."Task 5D: PROCESS IMAGE" ("Enum")) -> (s? t:f=w955:u16)
                n368 = Select(t=w955, s=w960, f=State_Type_Definitions."Task 5C: CAM BURST" ("Enum")) -> (s? t:f=w959:u16)
              }
              frame "Exit" {
                n369 = for {
                  shift-right: [w982] -> w979
                  shift-left: w976 -> [w983]
                  tunnel: string[] ["STOP", "RESET ENCODERS", "RESET YAW", "ARDUINO MODE 0"] -> [w981] mode=indexing
                  n370 = Enqueue Element(queue=w983, element=w981) -> (queue out=w982:refnum<queue>)  [unwired: 2 in, 2 out]
                }
              }
            }
          }
          frame 18 {
            # ">>> yStepper command>>>"
            n371 = Dequeue Element(queue=w990, timeout in ms (-1)=w989, error in (no error)=w988) -> (element=w987:T10)  [unwired: 3 out]
            n372 = case shown="\"None\", Default" w987 {
              tunnel: [w1002 State_Type_Definitions."True Stop" ("Enum")] -> w994
              tunnel: [w1005 w1022] -> w993
              tunnel: [State_Type_Definitions."Idle" ("Enum") State_Type_Definitions."Shutdown" ("Enum")] -> w995
              tunnel: w991 -> [w1001 _]
              tunnel: w992 -> [w997 w1019]
              tunnel: w985 -> [w996 _]
              frame "None", Default {
                # ">> T: Breaks out of state loop; F: Stays in loop>>"
                # ">> Manual override >>"
                # ">> Checks if time is up>>"
                # "Stays in Task 5D until the object is detected"
                # "T: Go back to idle, F: Continue with task\""
                # ">> Manual override >>"
                n373 = case shown="True" w996 {
                  tunnel: [w1009 w1015] -> w1005
                  tunnel: w997 -> [w1007 w1013]
                  frame False {
                    n374 = for {
                      tunnel: string[] ["START TIMER", "PROCESS IMAGE", ""] ("element") -> [w1010] mode=indexing
                      shift-right: [w1012] -> w1009
                      shift-left: w1007 -> [w1011]
                      n375 = Enqueue Element(queue=w1011, element=w1010) -> (queue out=w1012:refnum<queue>)  [unwired: 2 in, 2 out]
                    }
                  }
                  frame True {
                    n376 = for {
                      shift-right: [w1017] -> w1015
                      shift-left: w1013 -> [w1018]
                      tunnel: string[] ["CAM CLOSE", "", ""] -> [w1016] mode=indexing
                      n377 = Enqueue Element(queue=w1018, element=w1016) -> (queue out=w1017:refnum<queue>)  [unwired: 2 in, 2 out]
                    }
                  }
                }
                n378 = Or(x=w996, y=w1001) -> (x .or. y?=w1003:bool)
                n379 = Select(t=State_Type_Definitions."True Stop" ("Enum"), s=w1001, f=State_Type_Definitions."Task 5E: POSITION ARM" ("Enum")) -> (s? t:f=w998:T9)
                n380 = Select(t=w998, s=w1003, f=State_Type_Definitions."Task 5D: PROCESS IMAGE" ("Enum")) -> (s? t:f=w1002:u16)
              }
              frame "Exit" {
                n381 = for {
                  shift-right: [w1025] -> w1022
                  shift-left: w1019 -> [w1026]
                  tunnel: string[] ["STOP", "RESET ENCODERS", "RESET YAW", "ARDUINO MODE 0"] -> [w1024] mode=indexing
                  n382 = Enqueue Element(queue=w1026, element=w1024) -> (queue out=w1025:refnum<queue>)  [unwired: 2 in, 2 out]
                }
              }
            }
          }
          frame 20 {
            # ">>> yStepper command>>>"
            n383 = Dequeue Element(queue=w1039, timeout in ms (-1)=w1040, error in (no error)=w1041) -> (element=w1043:T10)  [unwired: 3 out]
            n384 = formula code="if (pos < 100)\ny = 41;\n\nelse if (pos >= 100 && pos <= 140)\ny = 30;\n\nelse if (pos >= 141 && pos <= 170)\ny = 25;\n\nelse if (pos >= 171 &&pos <= 180) \ny = 20;\n\nelse if (pos >= 181&& pos <= 200)\ny = 15;\n\nelse if (pos >= 201 && pos <= 230)\ny = 10;\n\nelse if (pos >= 231 && pos <= 320)\ny = 8;\n\nelse if (pos > 320)\ny = 0;"("pos"=w1031) -> ("y"=w1034:dbl)
            n385 = To Unsigned Byte Integer(number=w1034) -> (unsigned 8bit integer=w1029:u8)
            n386 = Equal?(x=w1030, y=w1029) -> (x = y?=w1028:bool)
            n387 = case shown="\"None\", Default" w1043 {
              tunnel: [w1050 State_Type_Definitions."True Stop" ("Enum")] -> w1037
              tunnel: [w1053 w1070] -> w1035
              tunnel: [State_Type_Definitions."Idle" ("Enum") State_Type_Definitions."Shutdown" ("Enum")] -> w1036
              tunnel: w1042 -> [w1049 _]
              tunnel: w1038 -> [w1045 w1067]
              tunnel: w1028 -> [w1044 _]
              frame "None", Default {
                # ">> T: Breaks out of state loop; F: Stays in loop>>"
                # ">> Manual override >>"
                # ">> Checks if time is up>>"
                # "Stays in Task 5D until the object is detected"
                # "T: Go back to idle, F: Continue with task\""
                # ">> Manual override >>"
                n388 = case shown="False" w1044 {
                  tunnel: [w1057 w1063] -> w1053
                  tunnel: w1045 -> [w1055 w1061]
                  frame False {
                    n389 = for {
                      tunnel: string[] ["READ STEPPER VALUES", "Y STEPPER CONTROL", ""] ("element") -> [w1058] mode=indexing
                      shift-right: [w1060] -> w1057
                      shift-left: w1055 -> [w1059]
                      n390 = Enqueue Element(queue=w1059, element=w1058) -> (queue out=w1060:refnum<queue>)  [unwired: 2 in, 2 out]
                    }
                  }
                  frame True {
                    n391 = for {
                      shift-right: [w1065] -> w1063
                      shift-left: w1061 -> [w1066]
                      tunnel: string[] ["CAM CLOSE", "DISPOSE BUFFERS", ""] -> [w1064] mode=indexing
                      n392 = Enqueue Element(queue=w1066, element=w1064) -> (queue out=w1065:refnum<queue>)  [unwired: 2 in, 2 out]
                    }
                  }
                }
                n393 = Or(x=w1044, y=w1049) -> (x .or. y?=w1051:bool)
                n394 = Select(t=State_Type_Definitions."True Stop" ("Enum"), s=w1049, f=State_Type_Definitions."Task 5F: ARM GRAB HEIGHT" ("Enum")) -> (s? t:f=w1046:T9)
                n395 = Select(t=w1046, s=w1051, f=State_Type_Definitions."Task 5E: POSITION ARM" ("Enum")) -> (s? t:f=w1050:T9)
              }
              frame "Exit" {
                n396 = for {
                  shift-right: [w1073] -> w1070
                  shift-left: w1067 -> [w1074]
                  tunnel: string[] ["STOP", "RESET ENCODERS", "RESET YAW", "ARDUINO MODE 0"] -> [w1072] mode=indexing
                  n397 = Enqueue Element(queue=w1074, element=w1072) -> (queue out=w1073:refnum<queue>)  [unwired: 2 in, 2 out]
                }
              }
            }
            n398 = Bundle By Name(cluster=w1033, "yStepper desired"=w1029) -> (w1032:T14)
          }
          frame 21 {
            # ">>> Motor control cluster >>>"
            # ">>> yStepper command>>>"
            # ">> Manual override >>"
            n399 = Dequeue Element(queue=w1084, timeout in ms (-1)=w1083, error in (no error)=w1085) -> (element=w1082:T10)  [unwired: 3 out]
            n400 = Equal?(x=w1081, y=u8 1) -> (x = y?=w1079:bool)
            n401 = case shown="\"None\", Default" w1082 {
              tunnel: [w1095 State_Type_Definitions."True Stop" ("Enum")] -> w1086
              tunnel: [w1098 w1115] -> w1087
              tunnel: [State_Type_Definitions."Idle" ("Enum") State_Type_Definitions."Shutdown" ("Enum")] -> w1088
              tunnel: w1079 -> [w1094 _]
              tunnel: w1078 -> [w1093 _]
              tunnel: w1077 -> [w1089 w1112]
              frame "None", Default {
                # "Stays in Task 5F until stepper reaches desired \nheight"
                # "T: Go back to idle, F: Continue with task\""
                # ">> Manual override >>"
                n402 = case shown="True" w1094 {
                  tunnel: [w1102 w1108] -> w1098
                  tunnel: w1089 -> [w1100 w1106]
                  frame False {
                    n403 = for {
                      tunnel: string[] ["Z STEPPER GRAB HEIGHT", "READ STEPPER VALUES"] ("element") -> [w1103] mode=indexing
                      shift-right: [w1105] -> w1102
                      shift-left: w1100 -> [w1104]
                      n404 = Enqueue Element(queue=w1104, element=w1103) -> (queue out=w1105:refnum<queue>)  [unwired: 2 in, 2 out]
                    }
                  }
                  frame True {
                    n405 = for {
                      shift-right: [w1110] -> w1108
                      shift-left: w1106 -> [w1111]
                      tunnel: string[] ["SET TIMER 5", "CLOSE CLAW", ""] -> [w1109] mode=indexing
                      n406 = Enqueue Element(queue=w1111, element=w1109) -> (queue out=w1110:refnum<queue>)  [unwired: 2 in, 2 out]
                    }
                  }
                }
                n407 = Or(x=w1094, y=w1093) -> (x .or. y?=w1096:bool)
                n408 = Select(t=State_Type_Definitions."True Stop" ("Enum"), s=w1093, f=State_Type_Definitions."Task 5G: CLOSE CLAW" ("Enum")) -> (s? t:f=w1090:T9)
                n409 = Select(t=w1090, s=w1096, f=State_Type_Definitions."Task 5F: ARM GRAB HEIGHT" ("Enum")) -> (s? t:f=w1095:T9)
              }
              frame "Exit" {
                n410 = for {
                  shift-right: [w1118] -> w1115
                  shift-left: w1112 -> [w1119]
                  tunnel: string[] ["STOP", "RESET ENCODERS", "RESET YAW", "ARDUINO MODE 0"] -> [w1117] mode=indexing
                  n411 = Enqueue Element(queue=w1119, element=w1117) -> (queue out=w1118:refnum<queue>)  [unwired: 2 in, 2 out]
                }
              }
            }
          }
          frame 22 {
            # ">>> yStepper command>>>"
            # ">> Manual override >>"
            n412 = Dequeue Element(queue=w1129, timeout in ms (-1)=w1128, error in (no error)=w1127) -> (element=w1126:T10)  [unwired: 3 out]
            n413 = case shown="\"None\", Default" w1126 {
              tunnel: [w1138 State_Type_Definitions."True Stop" ("Enum")] -> w1131
              tunnel: [w1141 w1158] -> w1124
              tunnel: [State_Type_Definitions."Idle" ("Enum") State_Type_Definitions."Shutdown" ("Enum")] -> w1123
              tunnel: w1125 -> [w1132 _]
              tunnel: w1130 -> [w1137 w1155]
              tunnel: w1121 -> [w1136 _]
              frame "None", Default {
                # ">> Is time up? >>"
                # "Determines if object is in range to pick up"
                # ">> Manual override >>"
                n414 = case shown="True" w1136 {
                  tunnel: [w1145 w1151] -> w1141
                  tunnel: w1137 -> [w1143 w1149]
                  frame False {
                    n415 = for {
                      tunnel: string[] ["CLOSE CLAW", "START TIMER"] ("element") -> [w1146] mode=indexing
                      shift-right: [w1148] -> w1145
                      shift-left: w1143 -> [w1147]
                      n416 = Enqueue Element(queue=w1147, element=w1146) -> (queue out=w1148:refnum<queue>)  [unwired: 2 in, 2 out]
                    }
                  }
                  frame True {
                    n417 = for {
                      shift-right: [w1153] -> w1151
                      shift-left: w1149 -> [w1154]
                      tunnel: string[] ["READ STEPPER VALUES", "", ""] -> [w1152] mode=indexing
                      n418 = Enqueue Element(queue=w1154, element=w1152) -> (queue out=w1153:refnum<queue>)  [unwired: 2 in, 2 out]
                    }
                  }
                }
                n419 = Or(x=w1136, y=w1132) -> (x .or. y?=w1139:bool)
                n420 = Select(t=State_Type_Definitions."True Stop" ("Enum"), s=w1132, f=State_Type_Definitions."Task 5H: RAISE ARM" ("Enum")) -> (s? t:f=w1134:T9)
                n421 = Select(t=w1134, s=w1139, f=State_Type_Definitions."Task 5G: CLOSE CLAW" ("Enum")) -> (s? t:f=w1138:T9)
              }
              frame "Exit" {
                n422 = for {
                  shift-right: [w1161] -> w1158
                  shift-left: w1155 -> [w1162]
                  tunnel: string[] ["STOP", "RESET ENCODERS", "RESET YAW", "ARDUINO MODE 0"] -> [w1160] mode=indexing
                  n423 = Enqueue Element(queue=w1162, element=w1160) -> (queue out=w1161:refnum<queue>)  [unwired: 2 in, 2 out]
                }
              }
            }
          }
          frame 23 {
            # ">>> yStepper command>>>"
            # ">> Manual override >>"
            n424 = Dequeue Element(queue=w1172, timeout in ms (-1)=w1171, error in (no error)=w1173) -> (element=w1170:T10)  [unwired: 3 out]
            n425 = Equal?(x=w1169, y=u8 60) -> (x = y?=w1167:bool)
            n426 = case shown="\"None\", Default" w1170 {
              tunnel: [w1183 State_Type_Definitions."True Stop" ("Enum")] -> w1174
              tunnel: [w1186 w1203] -> w1175
              tunnel: [State_Type_Definitions."Idle" ("Enum") State_Type_Definitions."Shutdown" ("Enum")] -> w1176
              tunnel: w1167 -> [w1182 _]
              tunnel: w1166 -> [w1181 _]
              tunnel: w1165 -> [w1177 w1200]
              frame "None", Default {
                # "Stays in Task 5_A until stepper reaches desired \nheight"
                # "T: Go back to idle, F: Continue with task\""
                # ">> Manual override >>"
                n427 = case shown="False" w1182 {
                  tunnel: [w1190 w1196] -> w1186
                  tunnel: w1177 -> [w1188 w1194]
                  frame False {
                    n428 = for {
                      tunnel: string[] ["Z STEPPER CAM HEIGHT", "READ STEPPER VALUES"] ("element") -> [w1191] mode=indexing
                      shift-right: [w1193] -> w1190
                      shift-left: w1188 -> [w1192]
                      n429 = Enqueue Element(queue=w1192, element=w1191) -> (queue out=w1193:refnum<queue>)  [unwired: 2 in, 2 out]
                    }
                  }
                  frame True {
                    n430 = for {
                      shift-right: [w1198] -> w1196
                      shift-left: w1194 -> [w1199]
                      tunnel: string[] ["ARDUINO - ULTRASONIC", "READ ULTRASONIC", ""] -> [w1197] mode=indexing
                      n431 = Enqueue Element(queue=w1199, element=w1197) -> (queue out=w1198:refnum<queue>)  [unwired: 2 in, 2 out]
                    }
                  }
                }
                n432 = Or(x=w1182, y=w1181) -> (x .or. y?=w1184:bool)
                n433 = Select(t=State_Type_Definitions."True Stop" ("Enum"), s=w1181, f=State_Type_Definitions."True Stop" ("Enum")) -> (s? t:f=w1178:T9)
                n434 = Select(t=w1178, s=w1184, f=State_Type_Definitions."Task 5H: RAISE ARM" ("Enum")) -> (s? t:f=w1183:T9)
              }
              frame "Exit" {
                n435 = for {
                  shift-right: [w1206] -> w1203
                  shift-left: w1200 -> [w1207]
                  tunnel: string[] ["STOP", "RESET ENCODERS", "RESET YAW", "ARDUINO MODE 0"] -> [w1205] mode=indexing
                  n436 = Enqueue Element(queue=w1207, element=w1205) -> (queue out=w1206:refnum<queue>)  [unwired: 2 in, 2 out]
                }
              }
            }
          }
          frame 24 {
            # ">>> yStepper command>>>"
            n437 = Dequeue Element(queue=w1216, timeout in ms (-1)=w1215, error in (no error)=w1214) -> (element=w1221:T10)  [unwired: 3 out]
            n438 = Equal?(x=w1212, y=u8 60) -> (x = y?=w1211:bool)
            n439 = case shown="\"None\", Default" w1221 {
              tunnel: [w1228 State_Type_Definitions."True Stop" ("Enum")] -> w1219
              tunnel: [w1227 w1245] -> w1218
              tunnel: [State_Type_Definitions."Idle" ("Enum") State_Type_Definitions."Shutdown" ("Enum")] -> w1220
              tunnel: w1217 -> [w1223 _]
              tunnel: w1213 -> [w1225 _]
              tunnel: w1211 -> [w1222 _]
              frame "None", Default {
                n440 = case shown="False" w1222 {
                  tunnel: [w1233 w1239] -> w1227
                  tunnel: w1225 -> [w1231 w1237]
                  frame False {
                    n441 = for {
                      tunnel: string[] ["Z STEPPER CAM HEIGHT", "READ STEPPER VALUES"] ("element") -> [w1234] mode=indexing
                      shift-right: [w1236] -> w1233
                      shift-left: w1231 -> [w1235]
                      n442 = Enqueue Element(queue=w1235, element=w1234) -> (queue out=w1236:refnum<queue>)  [unwired: 2 in, 2 out]
                    }
                  }
                  frame True {
                    n443 = for {
                      shift-right: [w1241] -> w1239
                      shift-left: w1237 -> [w1242]
                      tunnel: string[] ["CAM ACQ", "OPEN LOG CAM"] -> [w1240] mode=indexing
                      n444 = Enqueue Element(queue=w1242, element=w1240) -> (queue out=w1241:refnum<queue>)  [unwired: 2 in, 2 out]
                    }
                  }
                }
                n445 = Or(x=w1222, y=w1223) -> (x .or. y?=w1224:bool)
                n446 = Select(t=State_Type_Definitions."Task 6_B" ("Enum"), s=w1224, f=State_Type_Definitions."Task 6_A" ("Enum")) -> (s? t:f=w1228:T9)
              }
              frame "Exit" {
                n447 = for {
                  shift-right: [w1248] -> w1245
                  shift-left: _ -> [w1249]
                  tunnel: string[] ["STOP", "RESET ENCODERS", "RESET YAW", "ARDUINO MODE 0"] -> [w1247] mode=indexing
                  n448 = Enqueue Element(queue=w1249, element=w1247) -> (queue out=w1248:refnum<queue>)  [unwired: 2 in, 2 out]
                }
              }
            }
          }
          frame 25 {
            # ">>> yStepper command>>>"
            n449 = Dequeue Element(queue=w1260, timeout in ms (-1)=w1258, error in (no error)=w1259) -> (element=w1257:T10)  [unwired: 3 out]
            n450 = case shown="\"None\", Default" w1257 {
              tunnel: [w1267 State_Type_Definitions."True Stop" ("Enum")] -> w1253
              tunnel: [w1266 w1285] -> w1261
              tunnel: [State_Type_Definitions."Idle" ("Enum") State_Type_Definitions."Shutdown" ("Enum")] -> w1254
              tunnel: w1256 -> [w1262 _]
              tunnel: w1255 -> [w1264 _]
              tunnel: w1252 -> [w1263 w1282]
              frame "None", Default {
                # ">> Manual override >>"
                n451 = case shown="True" w1264 {
                  tunnel: [w1272 w1278] -> w1266
                  tunnel: w1263 -> [w1271 w1276]
                  frame False {
                    n452 = for {
                      shift-right: [w1275] -> w1272
                      shift-left: w1271 -> [w1274]
                      tunnel: string[] ["CAM ACQ", "PROCESS IMAGE", "OPEN CLAW"] -> [w1273] mode=indexing
                      n453 = Enqueue Element(queue=w1274, element=w1273) -> (queue out=w1275:refnum<queue>)  [unwired: 2 in, 2 out]
                    }
                  }
                  frame True {
                    n454 = for {
                      shift-right: [w1280] -> w1278
                      shift-left: w1276 -> [w1281]
                      tunnel: string[] ["CAM ACQ", "PROCESS IMAGE", "CLOSE CLAW"] -> [w1279] mode=indexing
                      n455 = Enqueue Element(queue=w1281, element=w1279) -> (queue out=w1280:refnum<queue>)  [unwired: 2 in, 2 out]
                    }
                  }
                }
                n456 = Select(t=State_Type_Definitions."True Stop" ("Enum"), s=w1262, f=State_Type_Definitions."Task 6_B" ("Enum")) -> (s? t:f=w1267:T9)
              }
              frame "Exit" {
                # ">> State after true stop >>"
                # ">> Goes to true stop >>"
                n457 = for {
                  shift-right: [w1288] -> w1285
                  shift-left: w1282 -> [w1289]
                  tunnel: string[] ["STOP", "RESET ENCODERS", "RESET YAW", ""] -> [w1287] mode=indexing
                  n458 = Enqueue Element(queue=w1289, element=w1287) -> (queue out=w1288:refnum<queue>)  [unwired: 2 in, 2 out]
                }
              }
            }
          }
          frame 26 {
          }
          frame 27 {
            # ">>> yStepper command>>>"
            # ">> Manual override >>"
            n459 = Dequeue Element(queue=w1304, timeout in ms (-1)=w1303, error in (no error)=w1305) -> (element=w1302:T10)  [unwired: 3 out]
            n460 = Equal?(x=w1301, y=u8 60) -> (x = y?=w1299:bool)
            n461 = case shown="\"None\", Default" w1302 {
              tunnel: [w1315 State_Type_Definitions."True Stop" ("Enum")] -> w1306
              tunnel: [w1318 w1335] -> w1307
              tunnel: [State_Type_Definitions."Idle" ("Enum") State_Type_Definitions."Shutdown" ("Enum")] -> w1308
              tunnel: w1299 -> [w1314 _]
              tunnel: w1298 -> [w1313 _]
              tunnel: w1297 -> [w1309 w1332]
              frame "None", Default {
                # "Stays in Task 5_A until stepper reaches desired \nheight"
                # "T: Go back to idle, F: Continue with task\""
                # ">> Manual override >>"
                n462 = case shown="True" w1314 {
                  tunnel: [w1322 w1328] -> w1318
                  tunnel: w1309 -> [w1320 w1326]
                  frame False {
                    n463 = for {
                      tunnel: string[] ["Z STEPPER CAM HEIGHT", "READ STEPPER VALUES"] ("element") -> [w1323] mode=indexing
                      shift-right: [w1325] -> w1322
                      shift-left: w1320 -> [w1324]
                      n464 = Enqueue Element(queue=w1324, element=w1323) -> (queue out=w1325:refnum<queue>)  [unwired: 2 in, 2 out]
                    }
                  }
                  frame True {
                    n465 = for {
                      shift-right: [w1330] -> w1328
                      shift-left: w1326 -> [w1331]
                      tunnel: string[] ["ARDUINO - ULTRASONIC", "READ ULTRASONIC", ""] -> [w1329] mode=indexing
                      n466 = Enqueue Element(queue=w1331, element=w1329) -> (queue out=w1330:refnum<queue>)  [unwired: 2 in, 2 out]
                    }
                  }
                }
                n467 = Or(x=w1314, y=w1313) -> (x .or. y?=w1316:bool)
                n468 = Select(t=State_Type_Definitions."True Stop" ("Enum"), s=w1313, f=State_Type_Definitions."Task 8B: MOVE TO BOX" ("Enum")) -> (s? t:f=w1310:T9)
                n469 = Select(t=w1310, s=w1316, f=State_Type_Definitions."Task 8A: RAISE ARM" ("Enum")) -> (s? t:f=w1315:T9)
              }
              frame "Exit" {
                n470 = for {
                  shift-right: [w1338] -> w1335
                  shift-left: w1332 -> [w1339]
                  tunnel: string[] ["STOP", "RESET ENCODERS", "RESET YAW", "ARDUINO MODE 0"] -> [w1337] mode=indexing
                  n471 = Enqueue Element(queue=w1339, element=w1337) -> (queue out=w1338:refnum<queue>)  [unwired: 2 in, 2 out]
                }
              }
            }
          }
          frame 28 {
            w1346 = u8 20 ("y")
            # ">>> yStepper command>>>"
            n472 = Less?(x=w1343, y=w1346) -> (x < y?=w1344:bool)
            n473 = Dequeue Element(queue=w1350, timeout in ms (-1)=w1349, error in (no error)=w1351) -> (element=w1348:T10)  [unwired: 3 out]
            n474 = Less?(x=w1342, y=w1346) -> (x < y?=w1345:bool)
            n475 = And(x=w1345, y=w1344) -> (x .and. y?=w1341:bool)
            n476 = case shown="\"None\", Default" w1348 {
              tunnel: [w1363 State_Type_Definitions."True Stop" ("Enum")] -> w1353
              tunnel: [w1366 w1383] -> w1352
              tunnel: [State_Type_Definitions."Idle" ("Enum") State_Type_Definitions."Shutdown" ("Enum")] -> w1354
              tunnel: w1356 -> [w1362 _]
              tunnel: w1355 -> [w1358 w1380]
              tunnel: w1341 -> [w1357 _]
              frame "None", Default {
                # "Stays in Task 5_B to capture image over 5 seconds"
                # "T: Go back to idle, F: Continue with task\""
                # ">> Manual override >>"
                n477 = case shown="True" w1357 {
                  tunnel: [w1370 w1376] -> w1366
                  tunnel: w1358 -> [w1368 w1374]
                  frame False {
                    n478 = for {
                      tunnel: string[] ["FORWARD", "READ ULTRASONIC", "READ NAVX"] ("element") -> [w1371] mode=indexing
                      shift-right: [w1373] -> w1370
                      shift-left: w1368 -> [w1372]
                      n479 = Enqueue Element(queue=w1372, element=w1371) -> (queue out=w1373:refnum<queue>)  [unwired: 2 in, 2 out]
                    }
                  }
                  frame True {
                    n480 = for {
                      shift-right: [w1378] -> w1376
                      shift-left: w1374 -> [w1379]
                      tunnel: string[] ["STOP", "RESET ENCODERS", "OPEN LOG CAM", "SET TIMER 2", "OPEN IMAQ REF"] -> [w1377] mode=indexing
                      n481 = Enqueue Element(queue=w1379, element=w1377) -> (queue out=w1378:refnum<queue>)  [unwired: 2 in, 2 out]
                    }
                  }
                }
                n482 = Or(x=w1357, y=w1362) -> (x .or. y?=w1364:bool)
                n483 = Select(t=State_Type_Definitions."True Stop" ("Enum"), s=w1362, f=State_Type_Definitions."Task 8C: CAM BURST" ("Enum")) -> (s? t:f=w1359:T9)
                n484 = Select(t=w1359, s=w1364, f=State_Type_Definitions."Task 8B: MOVE TO BOX" ("Enum")) -> (s? t:f=w1363:T9)
              }
              frame "Exit" {
                n485 = for {
                  shift-right: [w1386] -> w1383
                  shift-left: w1380 -> [w1387]
                  tunnel: string[] ["STOP", "RESET ENCODERS", "RESET YAW", "ARDUINO MODE 0"] -> [w1385] mode=indexing
                  n486 = Enqueue Element(queue=w1387, element=w1385) -> (queue out=w1386:refnum<queue>)  [unwired: 2 in, 2 out]
                }
              }
            }
          }
          frame 29 {
            # ">>> Motor control cluster >>>"
            # ">>> yStepper command>>>"
            # ">> Manual override >>"
            n487 = Dequeue Element(queue=w1397, timeout in ms (-1)=w1396, error in (no error)=w1395) -> (element=w1394:T10)  [unwired: 3 out]
            n488 = case shown="\"None\", Default" w1394 {
              tunnel: [w1406 State_Type_Definitions."True Stop" ("Enum")] -> w1399
              tunnel: [w1409 w1426] -> w1392
              tunnel: [State_Type_Definitions."Idle" ("Enum") State_Type_Definitions."Shutdown" ("Enum")] -> w1391
              tunnel: w1393 -> [w1400 _]
              tunnel: w1398 -> [w1405 w1423]
              tunnel: w1389 -> [w1404 _]
              frame "None", Default {
                # ">> Is time up? >>"
                # "Determines if object is in range to pick up"
                # ">> Manual override >>"
                n489 = case shown="True" w1404 {
                  tunnel: [w1413 w1419] -> w1409
                  tunnel: w1405 -> [w1411 w1417]
                  frame False {
                    n490 = for {
                      tunnel: string[] ["CAM ACQ", "START TIMER"] ("element") -> [w1414] mode=indexing
                      shift-right: [w1416] -> w1413
                      shift-left: w1411 -> [w1415]
                      n491 = Enqueue Element(queue=w1415, element=w1414) -> (queue out=w1416:refnum<queue>)  [unwired: 2 in, 2 out]
                    }
                  }
                  frame True {
                    n492 = for {
                      shift-right: [w1421] -> w1419
                      shift-left: w1417 -> [w1422]
                      tunnel: string[] ["CAM CLOSE", "PROCESS IMAGE", "SET TIMER 5"] -> [w1420] mode=indexing
                      n493 = Enqueue Element(queue=w1422, element=w1420) -> (queue out=w1421:refnum<queue>)  [unwired: 2 in, 2 out]
                    }
                  }
                }
                n494 = Or(x=w1404, y=w1400) -> (x .or. y?=w1407:bool)
                n495 = Select(t=State_Type_Definitions."True Stop" ("Enum"), s=w1400, f=State_Type_Definitions."Task 8D: PROCESS IMAGE" ("Enum")) -> (s? t:f=w1402:T9)
                n496 = Select(t=w1402, s=w1407, f=State_Type_Definitions."Task 8C: CAM BURST" ("Enum")) -> (s? t:f=w1406:T9)
              }
              frame "Exit" {
                n497 = for {
                  shift-right: [w1429] -> w1426
                  shift-left: w1423 -> [w1430]
                  tunnel: string[] ["STOP", "RESET ENCODERS", "RESET YAW", "ARDUINO MODE 0"] -> [w1428] mode=indexing
                  n498 = Enqueue Element(queue=w1430, element=w1428) -> (queue out=w1429:refnum<queue>)  [unwired: 2 in, 2 out]
                }
              }
            }
          }
          frame 30 {
            # ">>> yStepper command>>>"
            n499 = Dequeue Element(queue=w1437, timeout in ms (-1)=w1436, error in (no error)=w1435) -> (element=w1434:T10)  [unwired: 3 out]
            n500 = case shown="\"None\", Default" w1434 {
              tunnel: [w1449 State_Type_Definitions."True Stop" ("Enum")] -> w1441
              tunnel: [w1452 w1469] -> w1440
              tunnel: [State_Type_Definitions."Idle" ("Enum") State_Type_Definitions."Shutdown" ("Enum")] -> w1442
              tunnel: w1438 -> [w1448 _]
              tunnel: w1439 -> [w1444 w1466]
              tunnel: w1432 -> [w1443 _]
              frame "None", Default {
                # ">> T: Breaks out of state loop; F: Stays in loop>>"
                # ">> Manual override >>"
                # ">> Checks if time is up>>"
                # "Stays in Task 5D until the object is detected"
                # "T: Go back to idle, F: Continue with task\""
                # ">> Manual override >>"
                n501 = case shown="False" w1443 {
                  tunnel: [w1456 w1462] -> w1452
                  tunnel: w1444 -> [w1454 w1460]
                  frame False {
                    n502 = for {
                      tunnel: string[] ["START TIMER", "PROCESS IMAGE", ""] ("element") -> [w1457] mode=indexing
                      shift-right: [w1459] -> w1456
                      shift-left: w1454 -> [w1458]
                      n503 = Enqueue Element(queue=w1458, element=w1457) -> (queue out=w1459:refnum<queue>)  [unwired: 2 in, 2 out]
                    }
                  }
                  frame True {
                    n504 = for {
                      shift-right: [w1464] -> w1462
                      shift-left: w1460 -> [w1465]
                      tunnel: string[] ["RESET ENCODERS", "", ""] -> [w1463] mode=indexing
                      n505 = Enqueue Element(queue=w1465, element=w1463) -> (queue out=w1464:refnum<queue>)  [unwired: 2 in, 2 out]
                    }
                  }
                }
                n506 = Or(x=w1443, y=w1448) -> (x .or. y?=w1450:bool)
                n507 = Select(t=State_Type_Definitions."True Stop" ("Enum"), s=w1448, f=State_Type_Definitions."Task 8E: ROBOT ADJUST" ("Enum")) -> (s? t:f=w1445:T9)
                n508 = Select(t=w1445, s=w1450, f=State_Type_Definitions."Task 8D: PROCESS IMAGE" ("Enum")) -> (s? t:f=w1449:T9)
              }
              frame "Exit" {
                n509 = for {
                  shift-right: [w1472] -> w1469
                  shift-left: w1466 -> [w1473]
                  tunnel: string[] ["STOP", "RESET ENCODERS", "RESET YAW", "ARDUINO MODE 0"] -> [w1471] mode=indexing
                  n510 = Enqueue Element(queue=w1473, element=w1471) -> (queue out=w1472:refnum<queue>)  [unwired: 2 in, 2 out]
                }
              }
            }
          }
          frame 31 {
            # ">>> Motor control cluster >>>"
            # ">>> yStepper command>>>"
            n511 = Dequeue Element(queue=w1489, timeout in ms (-1)=w1488, error in (no error)=w1487) -> (element=w1486:T10)  [unwired: 3 out]
            n512 = Subtract(x=w1484, y=300.0) -> (x-y=w1482:dbl)
            "x-y" <- w1482
            n513 = formula code="if (error < -80 && error >-300){\ndistance = -20;\nxSpeed = -30;\n}\n\nelse if (error <= 61&&error >= -80){\ndistance = -15;\nxSpeed = -30;\n}\n\nelse if (error <= -26 && error >= -60){\ndistance = -10;\nxSpeed = -30;\n}\n\nelse if (error >= -25 && error <= 25){\ndistance = 0;\nxSpeed = 0;\n}\n\nelse if (error >= 51 && error <= 80){\ndistance = 10;\nxSpeed = 30;\n}\n\nelse if (error >= 81 && error <= 100){\ndistance = 15;\nxSpeed = 30;\n}\n\nelse if (error >= 101 && error <= 120){\ndistance = 20;\nxSpeed = 30;\n}\n\nelse if (error >= 121 && error <= 150){\ndistance = 25;\nxSpeed = 30;\n}\n\nelse if (error < 250){\ndistance = 30;\nxSpeed = 30;\n}\n\nelse{\ndistance = 0;\nxSpeed = 0;\n}"("error"=w1482) -> ("distance"=w1477:dbl, "xSpeed"=w1479:dbl)
            n514 = formula code="if (target > 0){\nif (current  >= target)\noutput = 1;\n}\n\nelse if (target == 0){\nif (current == target)\noutput = 1;\n}\n\nelse if (target < 0){\nif (current <= target)\noutput = 1;\n}\n\nelse\noutput = 0;"("target"=w1477, "current"=w1478) -> ("output"=w1476:dbl)
            n515 = Bundle By Name(cluster=w1481, "xSpeed"=w1479) -> (w1480:T12)
            n516 = Equal?(x=w1476, y=1.0) -> (x = y?=w1474:bool)
            n517 = case shown="\"None\", Default" w1486 {
              tunnel: [w1501 State_Type_Definitions."True Stop" ("Enum")] -> w1493
              tunnel: [w1504 w1521] -> w1492
              tunnel: [State_Type_Definitions."Idle" ("Enum") State_Type_Definitions."Shutdown" ("Enum")] -> w1494
              tunnel: w1490 -> [w1500 _]
              tunnel: w1491 -> [w1496 w1518]
              tunnel: w1474 -> [w1495 _]
              frame "None", Default {
                # ">> T: Breaks out of state loop; F: Stays in loop>>"
                # ">> Manual override >>"
                # ">> Checks if time is up>>"
                # "Stays in Task 5D until the object is detected"
                # "T: Go back to idle, F: Continue with task\""
                # ">> Manual override >>"
                n518 = case shown="False" w1495 {
                  tunnel: [w1508 w1514] -> w1504
                  tunnel: w1496 -> [w1506 w1512]
                  frame False {
                    n519 = for {
                      tunnel: string[] ["X AXIS - SLOW", "READ ENCODERS", "READ NAVX"] ("element") -> [w1509] mode=indexing
                      shift-right: [w1511] -> w1508
                      shift-left: w1506 -> [w1510]
                      n520 = Enqueue Element(queue=w1510, element=w1509) -> (queue out=w1511:refnum<queue>)  [unwired: 2 in, 2 out]
                    }
                  }
                  frame True {
                    n521 = for {
                      shift-right: [w1516] -> w1514
                      shift-left: w1512 -> [w1517]
                      tunnel: string[] ["SET TIMER 2", "STOP", "READ STEPPER VALUES", ""] -> [w1515] mode=indexing
                      n522 = Enqueue Element(queue=w1517, element=w1515) -> (queue out=w1516:refnum<queue>)  [unwired: 2 in, 2 out]
                    }
                  }
                }
                n523 = Or(x=w1495, y=w1500) -> (x .or. y?=w1502:bool)
                n524 = Select(t=State_Type_Definitions."True Stop" ("Enum"), s=w1500, f=State_Type_Definitions."Task 8H: ARM ADJUST" ("Enum")) -> (s? t:f=w1497:T9)
                n525 = Select(t=w1497, s=w1502, f=State_Type_Definitions."Task 8E: ROBOT ADJUST" ("Enum")) -> (s? t:f=w1501:T9)
              }
              frame "Exit" {
                n526 = for {
                  shift-right: [w1524] -> w1521
                  shift-left: w1518 -> [w1525]
                  tunnel: string[] ["STOP", "RESET ENCODERS", "RESET YAW", "ARDUINO MODE 0"] -> [w1523] mode=indexing
                  n527 = Enqueue Element(queue=w1525, element=w1523) -> (queue out=w1524:refnum<queue>)  [unwired: 2 in, 2 out]
                }
              }
            }
          }
          frame 32 {
            # ">>> Motor control cluster >>>"
            # ">>> yStepper command>>>"
            # ">> Manual override >>"
            n528 = Dequeue Element(queue=w1535, timeout in ms (-1)=w1534, error in (no error)=w1533) -> (element=w1532:T10)  [unwired: 3 out]
            n529 = case shown="\"None\", Default" w1532 {
              tunnel: [w1544 State_Type_Definitions."True Stop" ("Enum")] -> w1537
              tunnel: [w1547 w1564] -> w1530
              tunnel: [State_Type_Definitions."Idle" ("Enum") State_Type_Definitions."Shutdown" ("Enum")] -> w1529
              tunnel: w1531 -> [w1538 _]
              tunnel: w1536 -> [w1543 w1561]
              tunnel: w1527 -> [w1542 _]
              frame "None", Default {
                # ">> Is time up? >>"
                # "Determines if object is in range to pick up"
                # ">> Manual override >>"
                n530 = case shown="True" w1542 {
                  tunnel: [w1551 w1557] -> w1547
                  tunnel: w1543 -> [w1549 w1555]
                  frame False {
                    n531 = for {
                      tunnel: string[] ["CAM ACQ", "START TIMER"] ("element") -> [w1552] mode=indexing
                      shift-right: [w1554] -> w1551
                      shift-left: w1549 -> [w1553]
                      n532 = Enqueue Element(queue=w1553, element=w1552) -> (queue out=w1554:refnum<queue>)  [unwired: 2 in, 2 out]
                    }
                  }
                  frame True {
                    n533 = for {
                      shift-right: [w1559] -> w1557
                      shift-left: w1555 -> [w1560]
                      tunnel: string[] ["CAM CLOSE", "PROCESS IMAGE", "SET TIMER 3"] -> [w1558] mode=indexing
                      n534 = Enqueue Element(queue=w1560, element=w1558) -> (queue out=w1559:refnum<queue>)  [unwired: 2 in, 2 out]
                    }
                  }
                }
                n535 = Or(x=w1542, y=w1538) -> (x .or. y?=w1545:bool)
                n536 = Select(t=State_Type_Definitions."True Stop" ("Enum"), s=w1538, f=State_Type_Definitions."Task 8G: PROCESS IMAGE 2" ("Enum")) -> (s? t:f=w1540:T9)
                n537 = Select(t=w1540, s=w1545, f=State_Type_Definitions."Task 8F: CAM BURST 2" ("Enum")) -> (s? t:f=w1544:T9)
              }
              frame "Exit" {
                n538 = for {
                  shift-right: [w1567] -> w1564
                  shift-left: w1561 -> [w1568]
                  tunnel: string[] ["STOP", "RESET ENCODERS", "RESET YAW", "ARDUINO MODE 0"] -> [w1566] mode=indexing
                  n539 = Enqueue Element(queue=w1568, element=w1566) -> (queue out=w1567:refnum<queue>)  [unwired: 2 in, 2 out]
                }
              }
            }
          }
          frame 33 {
            # ">>> yStepper command>>>"
            n540 = Dequeue Element(queue=w1575, timeout in ms (-1)=w1574, error in (no error)=w1573) -> (element=w1572:T10)  [unwired: 3 out]
            n541 = case shown="\"None\", Default" w1572 {
              tunnel: [w1587 State_Type_Definitions."True Stop" ("Enum")] -> w1579
              tunnel: [w1590 w1607] -> w1578
              tunnel: [State_Type_Definitions."Idle" ("Enum") State_Type_Definitions."Shutdown" ("Enum")] -> w1580
              tunnel: w1576 -> [w1586 _]
              tunnel: w1577 -> [w1582 w1604]
              tunnel: w1570 -> [w1581 _]
              frame "None", Default {
                # ">> T: Breaks out of state loop; F: Stays in loop>>"
                # ">> Manual override >>"
                # ">> Checks if time is up>>"
                # "Stays in Task 5D until the object is detected"
                # "T: Go back to idle, F: Continue with task\""
                # ">> Manual override >>"
                n542 = case shown="False" w1581 {
                  tunnel: [w1594 w1600] -> w1590
                  tunnel: w1582 -> [w1592 w1598]
                  frame False {
                    n543 = for {
                      tunnel: string[] ["START TIMER", "PROCESS IMAGE", ""] ("element") -> [w1595] mode=indexing
                      shift-right: [w1597] -> w1594
                      shift-left: w1592 -> [w1596]
                      n544 = Enqueue Element(queue=w1596, element=w1595) -> (queue out=w1597:refnum<queue>)  [unwired: 2 in, 2 out]
                    }
                  }
                  frame True {
                    n545 = for {
                      shift-right: [w1602] -> w1600
                      shift-left: w1598 -> [w1603]
                      tunnel: string[] ["READ STEPPER VALUES", "Y STEPPER CONTROL", ""] -> [w1601] mode=indexing
                      n546 = Enqueue Element(queue=w1603, element=w1601) -> (queue out=w1602:refnum<queue>)  [unwired: 2 in, 2 out]
                    }
                  }
                }
                n547 = Or(x=w1581, y=w1586) -> (x .or. y?=w1588:bool)
                n548 = Select(t=State_Type_Definitions."True Stop" ("Enum"), s=w1586, f=State_Type_Definitions."Task 8H: ARM ADJUST" ("Enum")) -> (s? t:f=w1583:T9)
                n549 = Select(t=w1583, s=w1588, f=State_Type_Definitions."Task 8G: PROCESS IMAGE 2" ("Enum")) -> (s? t:f=w1587:T9)
              }
              frame "Exit" {
                n550 = for {
                  shift-right: [w1610] -> w1607
                  shift-left: w1604 -> [w1611]
                  tunnel: string[] ["STOP", "RESET ENCODERS", "RESET YAW", "ARDUINO MODE 0"] -> [w1609] mode=indexing
                  n551 = Enqueue Element(queue=w1611, element=w1609) -> (queue out=w1610:refnum<queue>)  [unwired: 2 in, 2 out]
                }
              }
            }
          }
          frame 34 {
            # ">>> yStepper command>>>"
            n552 = Dequeue Element(queue=w1624, timeout in ms (-1)=w1625, error in (no error)=w1626) -> (element=w1628:T10)  [unwired: 3 out]
            n553 = formula code="if (pos <= 81)\ny = 40;\n\nelse if (pos >= 81 &&pos <= 120)\ny = 37;\n\nelse if (pos >= 121 && pos <= 140)\ny = 28;\n\nelse if (pos >= 141 && pos <= 170)\ny = 25;\n\nelse if (pos >= 171 &&pos <= 200) \ny = 20;\n\nelse if (pos >= 201&& pos <= 210)\ny = 15;\n\nelse if (pos >= 211 && pos <= 230)\ny = 10;\n\nelse if (pos >= 231 && pos <= 320)\ny = 8;\n\nelse if (pos > 320)\ny = 0;"("pos"=w1616) -> ("y"=w1619:dbl)
            n554 = To Unsigned Byte Integer(number=w1619) -> (unsigned 8bit integer=w1614:u8)
            n555 = Equal?(x=w1615, y=w1614) -> (x = y?=w1613:bool)
            n556 = case shown="\"None\", Default" w1628 {
              tunnel: [w1635 State_Type_Definitions."True Stop" ("Enum")] -> w1622
              tunnel: [w1638 w1655] -> w1620
              tunnel: [State_Type_Definitions."Idle" ("Enum") State_Type_Definitions."Shutdown" ("Enum")] -> w1621
              tunnel: w1627 -> [w1634 _]
              tunnel: w1623 -> [w1630 w1652]
              tunnel: w1613 -> [w1629 _]
              frame "None", Default {
                # ">> T: Breaks out of state loop; F: Stays in loop>>"
                # ">> Manual override >>"
                # ">> Checks if time is up>>"
                # "Stays in Task 5D until the object is detected"
                # "T: Go back to idle, F: Continue with task\""
                # ">> Manual override >>"
                n557 = case shown="False" w1629 {
                  tunnel: [w1642 w1648] -> w1638
                  tunnel: w1630 -> [w1640 w1646]
                  frame False {
                    n558 = for {
                      tunnel: string[] ["READ STEPPER VALUES", "Y STEPPER CONTROL", ""] ("element") -> [w1643] mode=indexing
                      shift-right: [w1645] -> w1642
                      shift-left: w1640 -> [w1644]
                      n559 = Enqueue Element(queue=w1644, element=w1643) -> (queue out=w1645:refnum<queue>)  [unwired: 2 in, 2 out]
                    }
                  }
                  frame True {
                    n560 = for {
                      shift-right: [w1650] -> w1648
                      shift-left: w1646 -> [w1651]
                      tunnel: string[] ["DISPOSE BUFFERS", "READ STEPPER VALUES", ""] -> [w1649] mode=indexing
                      n561 = Enqueue Element(queue=w1651, element=w1649) -> (queue out=w1650:refnum<queue>)  [unwired: 2 in, 2 out]
                    }
                  }
                }
                n562 = Or(x=w1629, y=w1634) -> (x .or. y?=w1636:bool)
                n563 = Select(t=State_Type_Definitions."True Stop" ("Enum"), s=w1634, f=State_Type_Definitions."Task 8I: ARM GRAB HEIGHT" ("Enum")) -> (s? t:f=w1631:T9)
                n564 = Select(t=w1631, s=w1636, f=State_Type_Definitions."Task 8H: ARM ADJUST" ("Enum")) -> (s? t:f=w1635:T9)
              }
              frame "Exit" {
                n565 = for {
                  shift-right: [w1658] -> w1655
                  shift-left: w1652 -> [w1659]
                  tunnel: string[] ["STOP", "RESET ENCODERS", "RESET YAW", "ARDUINO MODE 0"] -> [w1657] mode=indexing
                  n566 = Enqueue Element(queue=w1659, element=w1657) -> (queue out=w1658:refnum<queue>)  [unwired: 2 in, 2 out]
                }
              }
            }
            n567 = Bundle By Name(cluster=w1618, "yStepper desired"=w1614) -> (w1617:T14)
          }
          frame 35 {
            # ">>> Motor control cluster >>>"
            # ">>> yStepper command>>>"
            # ">> Manual override >>"
            n568 = Dequeue Element(queue=w1669, timeout in ms (-1)=w1668, error in (no error)=w1670) -> (element=w1667:T10)  [unwired: 3 out]
            n569 = Equal?(x=w1666, y=u8 1) -> (x = y?=w1664:bool)
            n570 = case shown="\"None\", Default" w1667 {
              tunnel: [w1680 State_Type_Definitions."True Stop" ("Enum")] -> w1671
              tunnel: [w1683 w1700] -> w1672
              tunnel: [State_Type_Definitions."Idle" ("Enum") State_Type_Definitions."Shutdown" ("Enum")] -> w1673
              tunnel: w1664 -> [w1679 _]
              tunnel: w1663 -> [w1678 _]
              tunnel: w1662 -> [w1674 w1697]
              frame "None", Default {
                # "Stays in Task 5F until stepper reaches desired \nheight"
                # "T: Go back to idle, F: Continue with task\""
                # ">> Manual override >>"
                n571 = case shown="True" w1679 {
                  tunnel: [w1687 w1693] -> w1683
                  tunnel: w1674 -> [w1685 w1691]
                  frame False {
                    n572 = for {
                      tunnel: string[] ["Z STEPPER GRAB HEIGHT", "READ STEPPER VALUES"] ("element") -> [w1688] mode=indexing
                      shift-right: [w1690] -> w1687
                      shift-left: w1685 -> [w1689]
                      n573 = Enqueue Element(queue=w1689, element=w1688) -> (queue out=w1690:refnum<queue>)  [unwired: 2 in, 2 out]
                    }
                  }
                  frame True {
                    n574 = for {
                      shift-right: [w1695] -> w1693
                      shift-left: w1691 -> [w1696]
                      tunnel: string[] ["SET TIMER 2", "CLOSE CLAW", ""] -> [w1694] mode=indexing
                      n575 = Enqueue Element(queue=w1696, element=w1694) -> (queue out=w1695:refnum<queue>)  [unwired: 2 in, 2 out]
                    }
                  }
                }
                n576 = Or(x=w1679, y=w1678) -> (x .or. y?=w1681:bool)
                n577 = Select(t=State_Type_Definitions."True Stop" ("Enum"), s=w1678, f=State_Type_Definitions."Task 8J: CLOSE CLAW" ("Enum")) -> (s? t:f=w1675:T9)
                n578 = Select(t=w1675, s=w1681, f=State_Type_Definitions."Task 8I: ARM GRAB HEIGHT" ("Enum")) -> (s? t:f=w1680:T9)
              }
              frame "Exit" {
                n579 = for {
                  shift-right: [w1703] -> w1700
                  shift-left: w1697 -> [w1704]
                  tunnel: string[] ["STOP", "RESET ENCODERS", "RESET YAW", "ARDUINO MODE 0"] -> [w1702] mode=indexing
                  n580 = Enqueue Element(queue=w1704, element=w1702) -> (queue out=w1703:refnum<queue>)  [unwired: 2 in, 2 out]
                }
              }
            }
          }
          frame 36 {
            # ">>> yStepper command>>>"
            # ">> Manual override >>"
            n581 = Dequeue Element(queue=w1714, timeout in ms (-1)=w1713, error in (no error)=w1712) -> (element=w1711:T10)  [unwired: 3 out]
            n582 = case shown="\"None\", Default" w1711 {
              tunnel: [w1723 State_Type_Definitions."True Stop" ("Enum")] -> w1716
              tunnel: [w1726 w1743] -> w1709
              tunnel: [State_Type_Definitions."Idle" ("Enum") State_Type_Definitions."Shutdown" ("Enum")] -> w1708
              tunnel: w1710 -> [w1717 _]
              tunnel: w1715 -> [w1722 w1740]
              tunnel: w1706 -> [w1721 _]
              frame "None", Default {
                # ">> Is time up? >>"
                # "Determines if object is in range to pick up"
                # ">> Manual override >>"
                n583 = case shown="True" w1721 {
                  tunnel: [w1730 w1736] -> w1726
                  tunnel: w1722 -> [w1728 w1734]
                  frame False {
                    n584 = for {
                      tunnel: string[] ["CLOSE CLAW", "START TIMER"] ("element") -> [w1731] mode=indexing
                      shift-right: [w1733] -> w1730
                      shift-left: w1728 -> [w1732]
                      n585 = Enqueue Element(queue=w1732, element=w1731) -> (queue out=w1733:refnum<queue>)  [unwired: 2 in, 2 out]
                    }
                  }
                  frame True {
                    n586 = for {
                      shift-right: [w1738] -> w1736
                      shift-left: w1734 -> [w1739]
                      tunnel: string[] ["READ STEPPER VALUES", "", ""] -> [w1737] mode=indexing
                      n587 = Enqueue Element(queue=w1739, element=w1737) -> (queue out=w1738:refnum<queue>)  [unwired: 2 in, 2 out]
                    }
                  }
                }
                n588 = Or(x=w1721, y=w1717) -> (x .or. y?=w1724:bool)
                n589 = Select(t=State_Type_Definitions."True Stop" ("Enum"), s=w1717, f=State_Type_Definitions."Task 8K: RAISE MY SWORD" ("Enum")) -> (s? t:f=w1719:T9)
                n590 = Select(t=w1719, s=w1724, f=State_Type_Definitions."Task 8J: CLOSE CLAW" ("Enum")) -> (s? t:f=w1723:T9)
              }
              frame "Exit" {
                n591 = for {
                  shift-right: [w1746] -> w1743
                  shift-left: w1740 -> [w1747]
                  tunnel: string[] ["STOP", "RESET ENCODERS", "RESET YAW", "ARDUINO MODE 0"] -> [w1745] mode=indexing
                  n592 = Enqueue Element(queue=w1747, element=w1745) -> (queue out=w1746:refnum<queue>)  [unwired: 2 in, 2 out]
                }
              }
            }
          }
          frame 37 {
            # ">>> yStepper command>>>"
            # ">> Manual override >>"
            n593 = Dequeue Element(queue=w1757, timeout in ms (-1)=w1756, error in (no error)=w1758) -> (element=w1755:T10)  [unwired: 3 out]
            n594 = Equal?(x=w1754, y=u8 60) -> (x = y?=w1752:bool)
            n595 = case shown="\"None\", Default" w1755 {
              tunnel: [w1768 State_Type_Definitions."True Stop" ("Enum")] -> w1759
              tunnel: [w1771 w1788] -> w1760
              tunnel: [State_Type_Definitions."Idle" ("Enum") State_Type_Definitions."Shutdown" ("Enum")] -> w1761
              tunnel: w1752 -> [w1767 _]
              tunnel: w1751 -> [w1766 _]
              tunnel: w1750 -> [w1762 w1785]
              frame "None", Default {
                # "Stays in Task 5_A until stepper reaches desired \nheight"
                # "T: Go back to idle, F: Continue with task\""
                # ">> Manual override >>"
                n596 = case shown="True" w1767 {
                  tunnel: [w1775 w1781] -> w1771
                  tunnel: w1762 -> [w1773 w1779]
                  frame False {
                    n597 = for {
                      tunnel: string[] ["Z STEPPER CAM HEIGHT", "READ STEPPER VALUES"] ("element") -> [w1776] mode=indexing
                      shift-right: [w1778] -> w1775
                      shift-left: w1773 -> [w1777]
                      n598 = Enqueue Element(queue=w1777, element=w1776) -> (queue out=w1778:refnum<queue>)  [unwired: 2 in, 2 out]
                    }
                  }
                  frame True {
                    n599 = for {
                      shift-right: [w1783] -> w1781
                      shift-left: w1779 -> [w1784]
                      tunnel: string[] ["CAM CLOSE", "DISPOSE ALL BUFFERS", ""] -> [w1782] mode=indexing
                      n600 = Enqueue Element(queue=w1784, element=w1782) -> (queue out=w1783:refnum<queue>)  [unwired: 2 in, 2 out]
                    }
                  }
                }
                n601 = Or(x=w1767, y=w1766) -> (x .or. y?=w1769:bool)
                n602 = Select(t=State_Type_Definitions."True Stop" ("Enum"), s=w1766, f=State_Type_Definitions."True Stop" ("Enum")) -> (s? t:f=w1763:T9)
                n603 = Select(t=w1763, s=w1769, f=State_Type_Definitions."Task 8K: RAISE MY SWORD" ("Enum")) -> (s? t:f=w1768:T9)
              }
              frame "Exit" {
                n604 = for {
                  shift-right: [w1791] -> w1788
                  shift-left: w1785 -> [w1792]
                  tunnel: string[] ["STOP", "RESET ENCODERS", "RESET YAW", "ARDUINO MODE 0"] -> [w1790] mode=indexing
                  n605 = Enqueue Element(queue=w1792, element=w1790) -> (queue out=w1791:refnum<queue>)  [unwired: 2 in, 2 out]
                }
              }
            }
          }
          frame 38 {
            # ">> Stepper height reeached >>"
            # ">>> yStepper command>>>"
            # ">> Manual override >>"
            n606 = Dequeue Element(queue=w1803, timeout in ms (-1)=w1798, error in (no error)=w1802) -> (element=w1806:T10)  [unwired: 3 out]
            n607 = Equal?(x=w1800, y=u8 40) -> (x = y?=w1804:bool)
            n608 = case shown="\"None\", Default" w1806 {
              tunnel: [w1817 State_Type_Definitions."True Stop" ("Enum")] -> w1796
              tunnel: [w1815 w1832] -> w1795
              tunnel: w1799 -> [w1814 _]
              tunnel: w1801 -> [w1808 _]
              tunnel: [State_Type_Definitions."Idle" ("Enum") State_Type_Definitions."Shutdown" ("Enum")] -> w1797
              tunnel: w1804 -> [w1807 _]
              frame "None", Default {
                # ">> WIill proceed to part ii if not manual override >>"
                # ">>If ENABLE or Trigger is set to true>>"
                n609 = Or(x=w1807, y=w1808) -> (x .or. y?=w1809:bool)
                n610 = case shown="False" w1807 {
                  tunnel: [w1820 w1826] -> w1815
                  tunnel: w1814 -> [w1819 w1825]
                  frame False {
                    n611 = for {
                      shift-right: [w1822] -> w1820
                      shift-left: w1819 -> [w1823]
                      tunnel: string[] ["Z STEPPER BOX HEIGHT", "READ STEPPER VALUES"] ("element") -> [w1821] mode=indexing
                      n612 = Enqueue Element(queue=w1823, element=w1821) -> (queue out=w1822:refnum<queue>)  [unwired: 2 in, 2 out]
                    }
                  }
                  frame True {
                    n613 = for {
                      shift-right: [w1828] -> w1826
                      shift-left: w1825 -> [w1829]
                      tunnel: string[] ["ARDUINO - ULTRASONIC", "READ ULTRASONIC", "", "", "", ""] -> [w1827] mode=indexing
                      n614 = Enqueue Element(queue=w1829, element=w1827) -> (queue out=w1828:refnum<queue>)  [unwired: 2 in, 2 out]
                    }
                  }
                }
                n615 = Select(t=State_Type_Definitions."True Stop" ("Enum"), s=w1808, f=State_Type_Definitions."Task 9B: Rotate to Angle" ("Enum")) -> (s? t:f=w1811:T9)
                n616 = Select(t=w1811, s=w1809, f=State_Type_Definitions."Task 9A: Raise Arm" ("Enum")) -> (s? t:f=w1817:T9)
              }
              frame "Exit" {
                n617 = for {
                  shift-right: [w1835] -> w1832
                  shift-left: _ -> [w1836]
                  tunnel: string[] ["STOP", "RESET ENCODERS", "RESET YAW", ""] -> [w1834] mode=indexing
                  n618 = Enqueue Element(queue=w1836, element=w1834) -> (queue out=w1835:refnum<queue>)  [unwired: 2 in, 2 out]
                }
              }
            }
          }
          frame 39 {
            # ">>> yStepper command>>>"
            n619 = Dequeue Element(queue=w1849, timeout in ms (-1)=w1848, error in (no error)=w1847) -> (element=w1851:T10)  [unwired: 3 out]
            n620 = In Range and Coerce(upper limit=65.0, x=w1841, lower limit=55.0) -> (In Range?=w1838:bool)  [unwired: 1 out]
            n621 = case shown="\"None\", Default" w1851 {
              tunnel: w1842 -> [w1854 _]
              tunnel: [w1862 State_Type_Definitions."True Stop" ("Enum")] -> w1844
              tunnel: w1850 -> [w1860 w1878]
              tunnel: [w1859 w1877] -> w1843
              tunnel: [State_Type_Definitions."Idle" ("Enum") State_Type_Definitions."Shutdown" ("Enum")] -> w1845
              tunnel: w1838 -> [w1852 _]
              frame "None", Default {
                n622 = Or(x=w1852, y=w1854) -> (x .or. y?=w1853:bool)
                n623 = case shown="True" w1852 {
                  tunnel: w1860 -> [w1865 w1871]
                  tunnel: [w1864 w1869] -> w1859
                  frame False {
                    n624 = for {
                      shift-right: [w1867] -> w1864
                      shift-left: w1865 -> [w1868]
                      tunnel: string[] ["READ NAVX", "R-ACW"] ("element") -> [w1866] mode=indexing
                      n625 = Enqueue Element(queue=w1868, element=w1866) -> (queue out=w1867:refnum<queue>)  [unwired: 2 in, 2 out]
                    }
                  }
                  frame True {
                    n626 = for {
                      shift-right: [w1873] -> w1869
                      shift-left: w1871 -> [w1874]
                      tunnel: string[] ["STOP", "RESET ENCODERS", "RESET YAW", ""] -> [w1872] mode=indexing
                      n627 = Enqueue Element(queue=w1874, element=w1872) -> (queue out=w1873:refnum<queue>)  [unwired: 2 in, 2 out]
                    }
                  }
                }
                n628 = Select(t=State_Type_Definitions."True Stop" ("Enum"), s=w1854, f=State_Type_Definitions."Task 9C: Rotation alignmnet") -> (s? t:f=w1856:u16)
                n629 = Select(t=w1856, s=w1853, f=State_Type_Definitions."Task 9B: Rotate to Angle" ("Enum")) -> (s? t:f=w1862:u16)
              }
              frame "Exit" {
                n630 = for {
                  shift-right: [w1881] -> w1877
                  shift-left: w1878 -> [w1882]
                  tunnel: string[] ["STOP", "RESET ENCODERS", "RESET YAW", ""] -> [w1880] mode=indexing
                  n631 = Enqueue Element(queue=w1882, element=w1880) -> (queue out=w1881:refnum<queue>)  [unwired: 2 in, 2 out]
                }
              }
            }
          }
          frame 39 {
            # ">>> Motor control cluster >>>"
            # ">>Line Detected>>"
            # ">>Action Queue>>"
            # ">>> yStepper command>>>"
            n632 = Dequeue Element(queue=w1893, timeout in ms (-1)=w1892, error in (no error)=w1891) -> (element=w1894:T10)  [unwired: 3 out]
            n633 = case shown="\"None\", Default" w1894 {
              tunnel: w1889 -> [w1895 _]
              tunnel: [w1905 State_Type_Definitions."True Stop" ("Enum")] -> w1886
              tunnel: w1890 -> [w1903 w1921]
              tunnel: [w1902 w1920] -> w1885
              tunnel: [State_Type_Definitions."Idle" ("Enum") State_Type_Definitions."Shutdown" ("Enum")] -> w1888
              tunnel: w1883 -> [w1896 _]
              frame "None", Default {
                n634 = Or(x=w1895, y=w1896) -> (x .or. y?=w1897:bool)
                n635 = case shown="False" w1896 {
                  tunnel: w1903 -> [w1908 w1914]
                  tunnel: [w1907 w1912] -> w1902
                  frame False {
                    n636 = for {
                      shift-right: [w1910] -> w1907
                      shift-left: w1908 -> [w1911]
                      tunnel: string[] ["READ IR", "READ LINE SENSOR", "FORWARD - IR ASSIST"] ("element") -> [w1909] mode=indexing
                      n637 = Enqueue Element(queue=w1911, element=w1909) -> (queue out=w1910:refnum<queue>)  [unwired: 2 in, 2 out]
                    }
                  }
                  frame True {
                    n638 = for {
                      shift-right: [w1916] -> w1912
                      shift-left: w1914 -> [w1917]
                      tunnel: string[] ["STOP", "RESET ENCODERS", "RESET YAW", ""] -> [w1915] mode=indexing
                      n639 = Enqueue Element(queue=w1917, element=w1915) -> (queue out=w1916:refnum<queue>)  [unwired: 2 in, 2 out]
                    }
                  }
                }
                n640 = Select(t=State_Type_Definitions."True Stop" ("Enum"), s=w1895, f=State_Type_Definitions."Task 9D: Move Forward") -> (s? t:f=w1899:u16)
                n641 = Select(t=w1899, s=w1897, f=State_Type_Definitions."Task 9C: Rotation alignmnet" ("Enum")) -> (s? t:f=w1905:u16)
              }
              frame "Exit" {
                n642 = for {
                  shift-right: [w1924] -> w1920
                  shift-left: w1921 -> [w1925]
                  tunnel: string[] ["STOP", "RESET ENCODERS", "RESET YAW", ""] -> [w1923] mode=indexing
                  n643 = Enqueue Element(queue=w1925, element=w1923) -> (queue out=w1924:refnum<queue>)  [unwired: 2 in, 2 out]
                }
              }
            }
          }
          frame 40 {
            # ">> Manual override >>"
            # ">>Table Detected>>"
            # ">>> Motor control cluster >>>"
            # ">>Line Detected>>"
            # ">>Action Queue>>"
            # ">>> yStepper command>>>"
            n644 = Less Or Equal?(x=w1927, y=15.0) -> (x <= y?=w1926:bool)
            n645 = Dequeue Element(queue=w1938, timeout in ms (-1)=w1937, error in (no error)=w1936) -> (element=w1939:T10)  [unwired: 3 out]
            n646 = case shown="\"None\", Default" w1939 {
              tunnel: w1934 -> [w1940 _]
              tunnel: [w1950 State_Type_Definitions."True Stop" ("Enum")] -> w1931
              tunnel: w1935 -> [w1948 w1966]
              tunnel: [w1947 w1965] -> w1930
              tunnel: [State_Type_Definitions."Idle" ("Enum") State_Type_Definitions."Shutdown" ("Enum")] -> w1933
              tunnel: w1926 -> [w1941 _]
              frame "None", Default {
                n647 = Or(x=w1940, y=w1941) -> (x .or. y?=w1942:bool)
                n648 = case shown="True" w1941 {
                  tunnel: w1948 -> [w1953 w1959]
                  tunnel: [w1952 w1957] -> w1947
                  frame False {
                    n649 = for {
                      shift-right: [w1955] -> w1952
                      shift-left: w1953 -> [w1956]
                      tunnel: string[] ["READ IR", "FORWARD - IR ASSIST", ""] ("element") -> [w1954] mode=indexing
                      n650 = Enqueue Element(queue=w1956, element=w1954) -> (queue out=w1955:refnum<queue>)  [unwired: 2 in, 2 out]
                    }
                  }
                  frame True {
                    n651 = for {
                      shift-right: [w1961] -> w1957
                      shift-left: w1959 -> [w1962]
                      tunnel: string[] ["STOP", "RESET ENCODERS", "RESET YAW", ""] -> [w1960] mode=indexing
                      n652 = Enqueue Element(queue=w1962, element=w1960) -> (queue out=w1961:refnum<queue>)  [unwired: 2 in, 2 out]
                    }
                  }
                }
                n653 = Select(t=State_Type_Definitions."True Stop" ("Enum"), s=w1940, f=State_Type_Definitions."True Stop") -> (s? t:f=w1944:T9)
                n654 = Select(t=w1944, s=w1942, f=State_Type_Definitions."Task 9D: Move Forward" ("Enum")) -> (s? t:f=w1950:u16)
              }
              frame "Exit" {
                n655 = for {
                  shift-right: [w1969] -> w1965
                  shift-left: w1966 -> [w1970]
                  tunnel: string[] ["STOP", "RESET ENCODERS", "RESET YAW", ""] -> [w1968] mode=indexing
                  n656 = Enqueue Element(queue=w1970, element=w1968) -> (queue out=w1969:refnum<queue>)  [unwired: 2 in, 2 out]
                }
              }
            }
          }
          frame 41 {
            # ">> Stepper height reeached >>"
            # ">>> yStepper command>>>"
            # ">> Manual override >>"
            n657 = Dequeue Element(queue=w1981, timeout in ms (-1)=w1976, error in (no error)=w1980) -> (element=w1984:T10)  [unwired: 3 out]
            n658 = Equal?(x=w1978, y=u8 40) -> (x = y?=w1982:bool)
            n659 = case shown="\"None\", Default" w1984 {
              tunnel: [w1995 State_Type_Definitions."True Stop" ("Enum")] -> w1974
              tunnel: [w1993 w2011] -> w1973
              tunnel: w1977 -> [w1992 w2008]
              tunnel: w1979 -> [w1986 _]
              tunnel: [State_Type_Definitions."Idle" ("Enum") State_Type_Definitions."Shutdown" ("Enum")] -> w1975
              tunnel: w1982 -> [w1985 _]
              frame "None", Default {
                # ">> WIill proceed to part ii if not manual override >>"
                # ">>If ENABLE or Trigger is set to true>>"
                n660 = Or(x=w1985, y=w1986) -> (x .or. y?=w1987:bool)
                n661 = case shown="False" w1985 {
                  tunnel: [w1998 w2004] -> w1993
                  tunnel: w1992 -> [w1997 w2003]
                  frame False {
                    n662 = for {
                      shift-right: [w2000] -> w1998
                      shift-left: w1997 -> [w2001]
                      tunnel: string[] ["Z STEPPER BOX HEIGHT", "READ STEPPER VALUES"] ("element") -> [w1999] mode=indexing
                      n663 = Enqueue Element(queue=w2001, element=w1999) -> (queue out=w2000:refnum<queue>)  [unwired: 2 in, 2 out]
                    }
                  }
                  frame True {
                    n664 = for {
                      shift-right: [w2006] -> w2004
                      shift-left: w2003 -> [w2007]
                      tunnel: string[] ["READ IR", "", "", "", "", ""] -> [w2005] mode=indexing
                      n665 = Enqueue Element(queue=w2007, element=w2005) -> (queue out=w2006:refnum<queue>)  [unwired: 2 in, 2 out]
                    }
                  }
                }
                n666 = Select(t=State_Type_Definitions."True Stop" ("Enum"), s=w1986, f=State_Type_Definitions."Task A: MOVE FORWARD" ("Enum")) -> (s? t:f=w1989:u16)
                n667 = Select(t=w1989, s=w1987, f=State_Type_Definitions."Task A: RAISE ARM TO HEIGHT" ("Enum")) -> (s? t:f=w1995:u16)
              }
              frame "Exit" {
                n668 = for {
                  shift-right: [w2014] -> w2011
                  shift-left: w2008 -> [w2015]
                  tunnel: string[] ["STOP", "RESET ENCODERS", "RESET YAW", ""] -> [w2013] mode=indexing
                  n669 = Enqueue Element(queue=w2015, element=w2013) -> (queue out=w2014:refnum<queue>)  [unwired: 2 in, 2 out]
                }
              }
            }
          }
          frame 42 {
            # ">>> Motor control cluster >>>"
            # ">>> yStepper command>>>"
            # ">>Object detected>>"
            n670 = Dequeue Element(queue=w2024, timeout in ms (-1)=w2023, error in (no error)=w2022) -> (element=w2029:T10)  [unwired: 3 out]
            n671 = Less Or Equal?(x=w2018, y=30.0) -> (x <= y?=w2016:bool)
            "Table obstruct" <- w2016
            n672 = case shown="\"None\", Default" w2029 {
              tunnel: w2016 -> [w2032 _]
              tunnel: [w2039 State_Type_Definitions."True Stop" ("Enum")] -> w2028
              tunnel: w2021 -> [w2031 _]
              tunnel: w2025 -> [w2038 w2055]
              tunnel: [w2037 w2056] -> w2027
              tunnel: [State_Type_Definitions."Idle" ("Enum") State_Type_Definitions."Shutdown" ("Enum")] -> w2026
              frame "None", Default {
                n673 = case shown="False" w2032 {
                  tunnel: w2038 -> [w2042 w2049]
                  tunnel: [w2043 w2048] -> w2037
                  frame False {
                    n674 = for {
                      tunnel: string[] ["READ IR", "FORWARD", "READ NAVX"] ("element") -> [w2044] mode=indexing
                      shift-right: [w2046] -> w2043
                      shift-left: w2042 -> [w2045]
                      n675 = Enqueue Element(queue=w2045, element=w2044) -> (queue out=w2046:refnum<queue>)  [unwired: 2 in, 2 out]
                    }
                  }
                  frame True {
                    n676 = for {
                      shift-right: [w2051] -> w2048
                      shift-left: w2049 -> [w2052]
                      tunnel: string[] ["RESET ENCODERS", "READ NAVX", "READ ENCODERS"] -> [w2050] mode=indexing
                      n677 = Enqueue Element(queue=w2052, element=w2050) -> (queue out=w2051:refnum<queue>)  [unwired: 2 in, 2 out]
                    }
                  }
                }
                n678 = Or(x=w2032, y=w2031) -> (x .or. y?=w2030:bool)
                n679 = Select(t=State_Type_Definitions."True Stop" ("Enum"), s=w2031, f=State_Type_Definitions."True Stop" ("Enum")) -> (s? t:f=w2033:T9)
                n680 = Select(t=w2033, s=w2030, f=State_Type_Definitions."Task A: MOVE FORWARD" ("Enum")) -> (s? t:f=w2039:u16)
              }
              frame "Exit" {
                n681 = for {
                  shift-right: [w2059] -> w2056
                  shift-left: w2055 -> [w2060]
                  tunnel: string[] ["STOP", "RESET ENCODERS", "RESET YAW", "ARDUINO MODE 0"] -> [w2058] mode=indexing
                  n682 = Enqueue Element(queue=w2060, element=w2058) -> (queue out=w2059:refnum<queue>)  [unwired: 2 in, 2 out]
                }
              }
            }
          }
        }
      }
    }
    n683 = local write "Green LED"(w206) -> ()
  }
  n684 = while {
    stop <- w2717 stop-if-true
    n685 = call "MOTOR CONTROL WITH PID AE.vi"("AE Mode"=MOTOR_CONTROL_WITH_PID_AE_DATA_MODE_TYPE_DEF."Read from AE") -> ("Speed & distance"=→"Speed & distance":T4)  [unwired: 3 in]
    n686 = call "FGV Bool.vi"("Init/Read/Write State"=States_for_Action_Engine."Read") -> ("Output node"=w2717:bool)  [unwired: 2 in, 1 out]
    n687 = Wait (ms)(milliseconds to wait=u32 5) -> ()  [unwired: 1 out]
  }
  n688 = while {
    stop <- w2722 stop-if-true
    n689 = call <vilib>:"RT Get CPU Loads.vi"() -> ("CPU loads"=→"CPU loads":T8[])  [unwired: 10 in, 1 out]
    n690 = Wait (ms)(milliseconds to wait=u32 100) -> ()  [unwired: 1 out]
    n691 = call "FGV Bool.vi"("Init/Read/Write State"=States_for_Action_Engine."Read") -> ("Output node"=w2722:bool)  [unwired: 2 in, 1 out]
  }
  n692 = call <vilib>:"DIO Close.vi"("error in (no error)"=w22, "DIO Info In"=w25) -> ()  [unwired: 9 in, 1 out]
  n693 = call <vilib>:"DIO Close.vi"("error in (no error)"=w32, "DIO Info In"=w34) -> ()  [unwired: 9 in, 1 out]
  n694 = call <vilib>:"NavX Close.vi"("error in (no error)"=w9, "NavX Info In"=w8) -> ()  [unwired: 9 in, 1 out]
  n695 = call <vilib>:"DIO Close.vi"("error in (no error)"=w27, "DIO Info In"=w29) -> ()  [unwired: 9 in, 1 out]
  n696 = call <vilib>:"DIO Close.vi"("error in (no error)"=w16, "DIO Info In"=w17) -> ()  [unwired: 9 in, 1 out]
  n697 = call <vilib>:"DIO Close.vi"("error in (no error)"=w11, "DIO Info In"=w12) -> ()  [unwired: 9 in, 1 out]
  n698 = Merge Errors "Merge Errors"(w62, w61) -> (w44:errorcluster)
  n699 = Merge Errors(w48, w44) -> (w43:errorcluster)
  n700 = Destroy User Event(user event=w65, error in=w43) -> ()  [unwired: 1 out]
  n701 = Destroy User Event(user event=w66, error in=w43) -> ()  [unwired: 1 out]
  n702 = Unregister For Events(event registration refnum=w57, error in=w43) -> ()  [unwired: 1 out]
  n703 = Release Queue(queue=w39, error in (no error)=w43) -> (error out=→"Queue Errors":errorcluster)  [unwired: 1 in, 2 out]
  n704 = Release Queue(queue=w56, error in (no error)=w43) -> ()  [unwired: 1 in, 3 out]
